vi "reg_visu OPC2.vi"(7 "object_name":string="W1", 9 "Останов\nпрограммы":bool) -> ()   [LabVIEW 2019]
uses:
  projects/Additivs/Regulators/PROG/GM1_201007/enums/AI.ctl
  Heating/ctl/general_init_client.ctl
  OPC/OPC UA Client.ctl
  <vilib>/OPCUA/controls/OPC UA Client Refnum.ctl
  <vilib>/OPCUA/controls/NodeId.ctl
  <vilib>/OPCUA/controls/NodeIds.ctl
  <vilib>/OPCUA/controls/Subscription ID.ctl
  <vilib>/OPCUA/controls/Write Variant Request.ctl
  <vilib>/OPCUA/controls/Write Status.ctl
  <vilib>/OPCUA/controls/Subscription Data Change.ctl
  <vilib>/OPCUA/controls/Data Type.ctl
  <vilib>/OPCUA/controls/OPC UA StatusCode.ctl
  Database/ctl/Coninfo.ctl
  Inputs/Ctl/Parameter State.ctl
  Alarms/Ctl/ALRs_State.ctl
  ctl/Y_short.ctl
  Inputs/Ctl/Parameter State short.ctl
  projects/Additivs/Regulators/PROG/GM1_201007/enums/KFM.ctl
  projects/Additivs/Regulators/PROG/GM1_201007/enums/PAR.ctl
  projects/Additivs/Regulators/PROG/GM1_201007/enums/DI.ctl
  projects/Additivs/Regulators/PROG/GM1_201007/enums/DI_FAST.ctl
  projects/Additivs/Regulators/PROG/GM1_201007/enums/AO.ctl
  projects/Additivs/Regulators/PROG/GM1_201007/enums/DO.ctl
  projects/Additivs/Regulators/PROG/GM1_201007/enums/ALR.ctl
  projects/Additivs/Regulators/PROG/GM1_201007/enums/System.ctl
  projects/Additivs/Regulators/PROG/GM1_201007/enums/REG.ctl
  bronkhorst/bronkhorstColumns.ctl
  <vilib>/picture/picture.llb/imagedata.ctl
  ctl/Ys_short.ctl
  389b3f70-cfa1-4025-b690-dd9bbc3cc1e4.vi
  cf2ac22c-c8a5-4ec0-ba3c-9dae82546773.vi
  Database/PostgreSQL2LabVIEW/libpqUtility/src/PQconnect.vi
  Database/PostgreSQL2LabVIEW/libpqUtility/src/PQclose.vi
  Database/select_initial_all.vi
  <vilib>/NI/AMC/Create Single Message.vi
  <vilib>/NI/AMC/Update Message Routing Info.vi
  <vilib>/NI/AMC/Read Termination Message.vi
  Transform/JSON to array.vi
  Database/PostgreSQL2LabVIEW/libpqlv/src/PQfinish.vi
  Database/PostgreSQL2LabVIEW/libpqlv/src/PQconnectdb.vi
  Database/PostgreSQL2LabVIEW/libpqlv/src/PQerrorMessage.vi
  Database/PostgreSQL2LabVIEW/libpqlv/src/PQstatus.vi
  <vilib>/dlg_ctls.llb/Space Constant.vi
  <vilib>/JDP Science/JSONtext/Find Multiple Items.vi
  <vilib>/JDP Science/JSONtext/String Subset.vi
  <vilib>/JDP Science/JSONtext/support/Strip Quotes and Unescape.vi
  <vilib>/JDP Science/JSONtext/support/Unescape JSON string.vi
  <vilib>/Utility/config.llb/Read Key (String).vi
  <vilib>/OPCUA/client/Multiple Read String Array.vi
  Database/PostgreSQL2LabVIEW/libpqUtility/src/PQgetTable.vi
  Database/Progress.vi
  <vilib>/OPCUA/client/Multiple Read ByteString Array.vi
  <vilib>/NI/AMC/Send Message.vi
  <vilib>/NI/AMC/Globals.vi
  <vilib>/OPCUA/client/Multiple Read String.vi
  <vilib>/JDP Science/JSONtext/JSON text to Variant.vi
  <vilib>/OPCUA/client/Multiple Write Variant.vi
  <vilib>/JDP Science/JSONtext/Parsing/Parse Full Path or Item Name.vi
  <vilib>/JDP Science/JSONtext/Offset/Find Item Locations by Path.vi
  <vilib>/JDP Science/JSONtext/Get Array Elements.vi
  Reg visu/Reg visu.lvclass
  <vilib>/JDP Science/JSONtext/LVClass Serializer/JSONtext LVClass Serializer.lvclass
  Heating/ctl/Z_State.ctl
  Heating/Heating.lvlib
  Heating/ctl/Y_state.ctl
  Heating/ctl/Y_source.ctl
  Heating/ctl/ZM_State.ctl
  <vilib>/NI/AMC/AMC.lvlib
  <vilib>/OPCUA/NI OPC UA Client.lvlib
  Database/PostgreSQL.lvlib
  <vilib>/Utility/config.llb/NI_LVConfig.lvlib
  projects/Additivs/Regulators/PROG/GM1_201007/enums/Param_h0gm1.lvlib
  Inputs/Inputs.lvlib
  control.lvlib
  OPC/OPC addons.lvlib
  Inputs/Ctl/DI short.ctl
  Alarms/Alarms.lvlib
  Heating/ctl/ZY_control.ctl
  Alarms/Ctl/ALR_Status_short.ctl
  Heating/ctl/Y_short.ctl
  Heating/ctl/Z.ctl
  Heating/ctl/ZY_state_short.ctl
  projects/Additivs/Regulators/PROG/GM1_201007/enums/scada_prog_state.ctl
  Heating/ctl/YQ2/YQ2.xctl
  Heating/ctl/Z_OnSwitch/Z_OnSwitch.xctl
  Heating/ctl/ZY_state_OPC.ctl
  7b03969a-a950-4454-9689-61267dd49491.vi
  fdeea6ee-2705-42e7-9783-53477a0f0781.vi
  00ce5b65-c19c-4f2f-b5a6-2d8b920d64b8.vi
  d49def32-a249-4c88-86f5-dd42ff10ee1e.vi
  847353ff-c4dc-4a0d-82d8-8a8c8b1dd027.vi
  96cb8638-67ee-45ab-9e65-4cb433c703bb.vi
  5d0f38f1-9d99-409f-81fc-f0eb7cf3d60e.vi
  fe7cfdb3-b4e0-46ae-bded-47b821cc5e2e.vi
  96416696-a13a-4191-9eaf-5b72f20cf204.vi
  bronkhorst/bronkhorst_reg.lvclass
  Reg visu1/Reg visu/Reg visu1.lvclass
  Heating/ctl/Z_source.ctl
  <vilib>/OPCUA/client/Multiple Read UInt32 Array.vi
  <vilib>/OPCUA/client/Multiple Read Double Array.vi
  <vilib>/OPCUA/client/Multiple Read Int32 Array.vi
  <vilib>/OPCUA/client/Multiple Read Bool Array.vi
panel:
  in  "Stop":bool caption="Останов программы"
  out "GM1QN1_XQ01":dbl caption="расход" format="%#.0f"
  in  "password data DB":string
  in  "password system DB":string
  in  "N 20":i32
  in  "N 19":i32
  in  "N 18":i32=16
  in  "N 17":i32=15
  in  "N 16":i32=14
  in  "N 15":i32=13
  in  "N 14":i32=12
  in  "N 13":i32=11
  in  "N 12":i32=10
  in  "N 11":i32=9
  in  "N 10":i32
  in  "N 9":i32
  in  "N 8":i32=8
  in  "N 7":i32=7
  in  "N 6":i32=6
  in  "N 5":i32=5
  in  "N 4":i32=4
  in  "N 3":i32=3
  in  "N 2":i32=2
  in  "N 1":i32=1
  out "Control Name":string="object_full_name"
  in  "gas 5":string="Осн."
  in  "gas 4":string="ОСНОВНОЙ 2"
  in  "gas 3":string="ОСНОВНОЙ 1"
  in  "HT1 emergency stop":bool caption="Аварийный сброс"
  in  "Reset":bool
  in  "Start":bool
  out "PV 2":dbl(slide) scale=0.0..50.0 scale format="%#_4g"
  in  "tick":u32=100 caption="Время цикла основной программы" min=5 max=1000 step=1
  out "EB3BP1_XQ01":dbl caption="kPa" format="%#.1f"
  in  "AI_enum":T1
  out "CPU %":dbl(slide) scale=0.0..100.0
  in  "message name":string="AI redefine"
  in  "process":bool
  in  "gas":string="РАБОЧИЕ ГАЗЫ"
  in  "gas 2":string="ПНГ1"
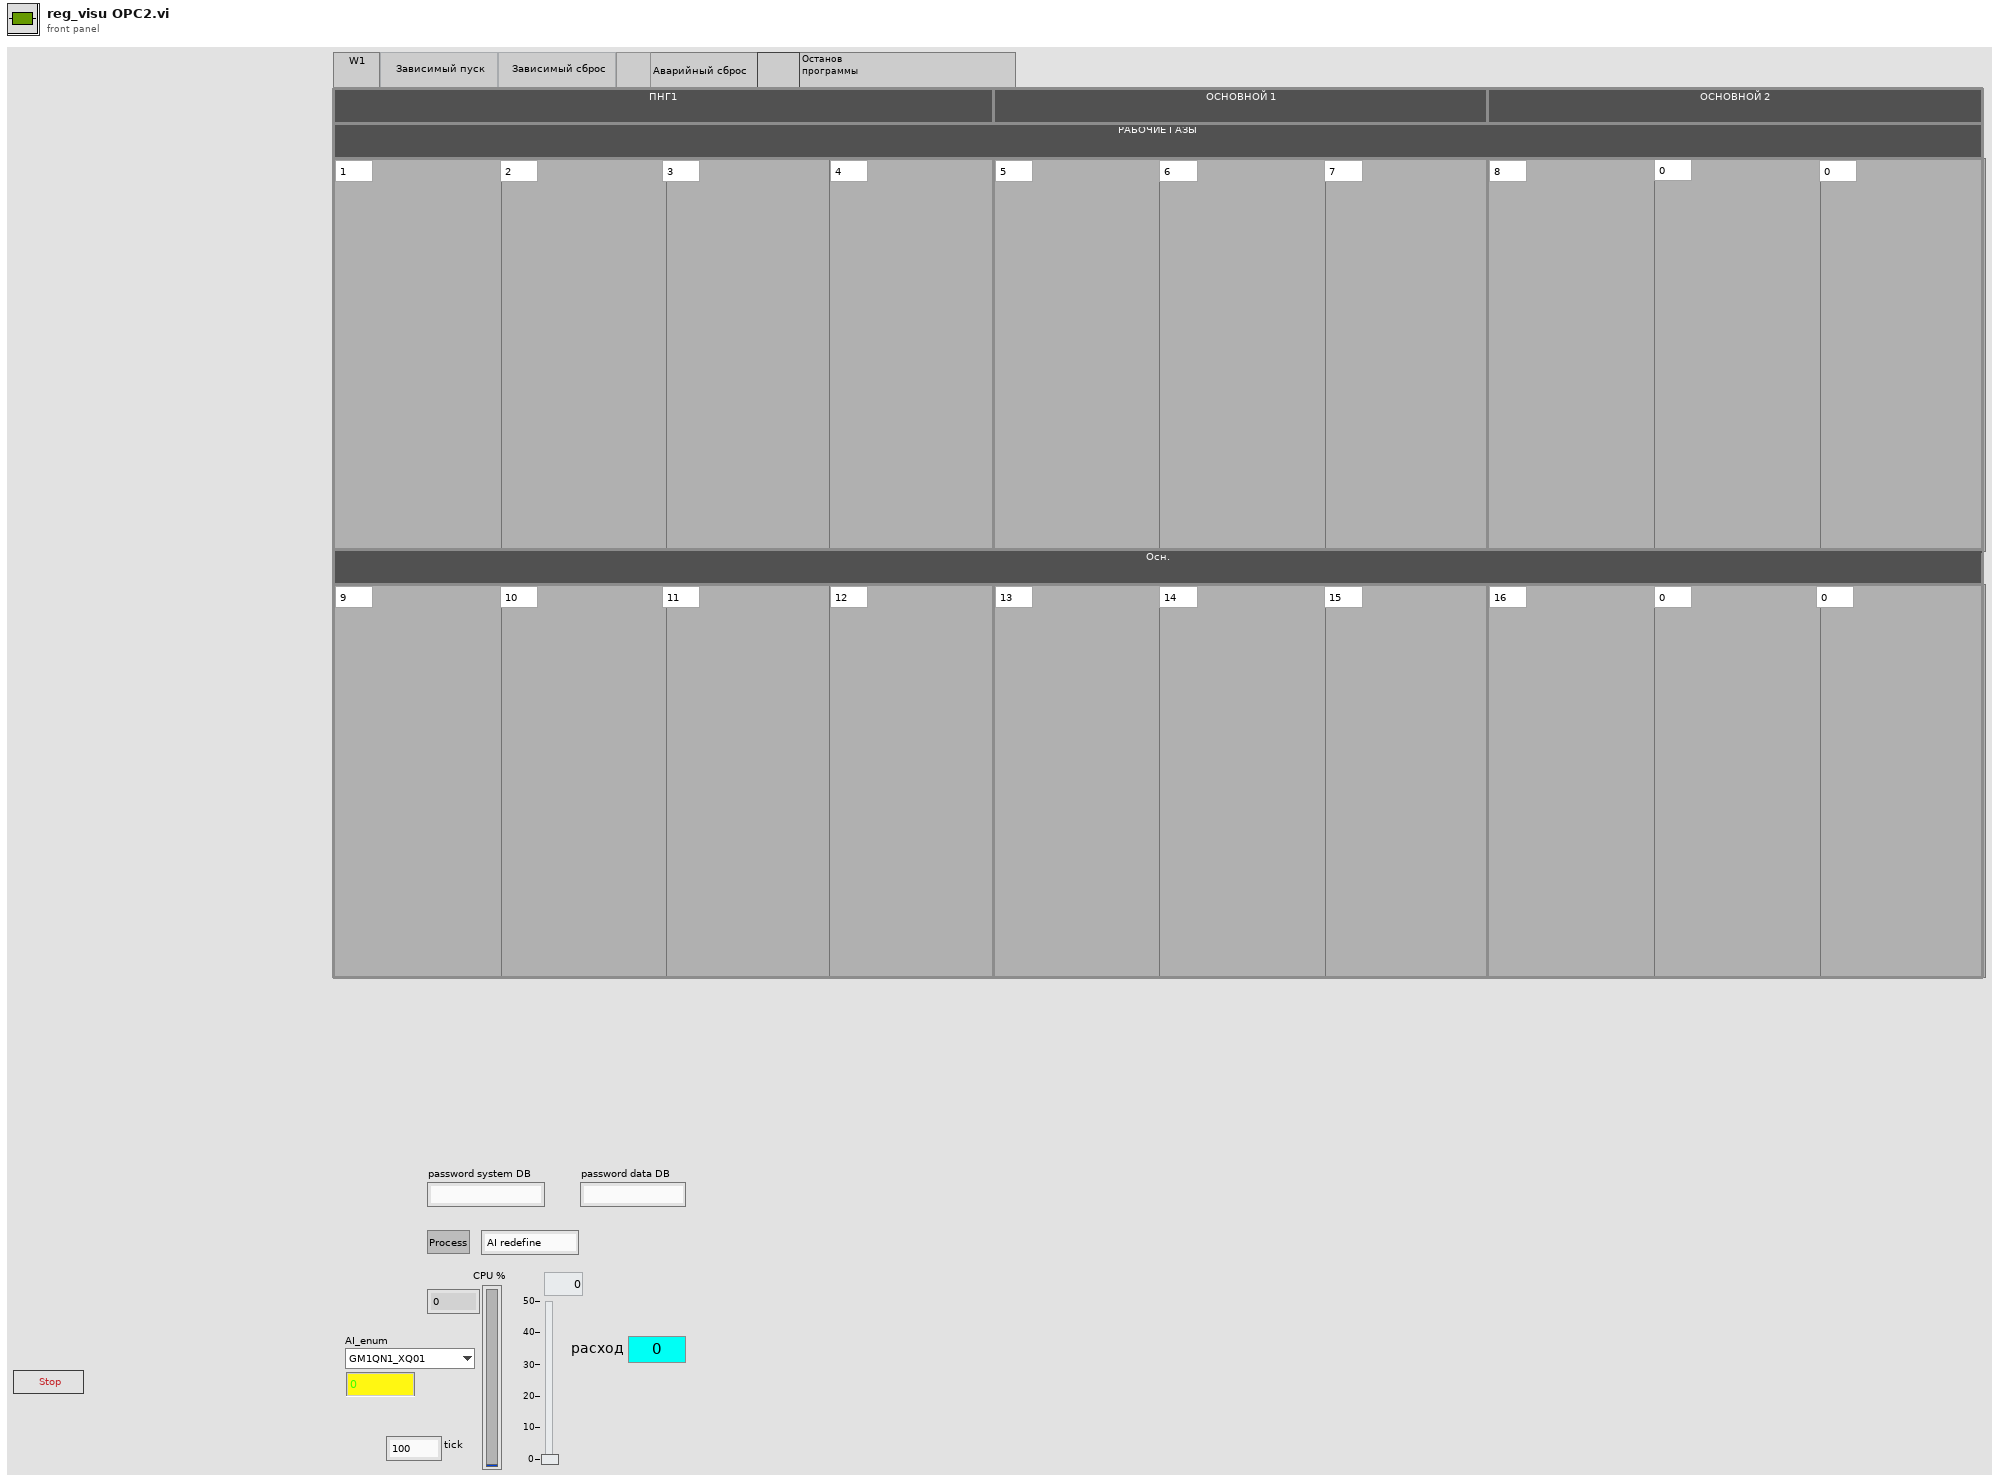
[diagram p1: front panel]
types:
  T1 = typedef "Param_h0gm1.lvlib/AI.ctl" = enum16{"GM1QN1_XQ01", "GM1QN2_XQ01", "GM1QN3_XQ01", "GM1QN4_XQ01", "GM1QN5_XQ01", "GM1QN6_XQ01", "GM1QN7_XQ01", "GM1QN8_XQ01", "GM1QN9_XQ01", "GM1QN10_XQ01", "GM1QN11_XQ01", "GM1QN12_XQ01", "GM1QN13_XQ01", "GM1QN14_XQ01", "GM1QN15_XQ01", "GM1QN16_XQ01", "GM1QN17_XQ01", "GM1QN18_XQ01", "GM1QN19_XQ01", "GM1QN20_XQ01", "GM1QN21_XQ01", "GM1QN22_XQ01", "GM1QN23_XQ01", "GM1QN1_XQ02", "GM1QN2_XQ02", "GM1QN3_XQ02", "GM1QN4_XQ02", "GM1QN5_XQ02", "GM1QN6_XQ02", "GM1QN7_XQ02", "GM1QN8_XQ02", "GM1QN9_XQ02", "GM1QN10_XQ02", "GM1QN11_XQ02", "GM1QN12_XQ02", "GM1QN13_XQ02", "GM1QN14_XQ02", "GM1QN15_XQ02", "GM1QN16_XQ02", "GM1QN17_XQ02", "GM1QN18_XQ02", "GM1QN19_XQ02", "GM1QN20_XQ02", "GM1QN21_XQ02", "GM1QN22_XQ02", "GM1QN23_XQ02"}
  T2 = typedef "Heating.lvlib/general_init_client.ctl" = enum16{"Init Data", "Init TMPs", "Read system DB param", "Read data DB param", "Read OPC param", "Read Enums", "Read Reg param", "Connect to OPC", "Read Param", "Read AI param", "AI references", "AI reorder", "AI reorder1", "AI Descriptions", "AI Descriptions1", "Read DI param", "Read AO param", "Read DO param", "Read ALR param", "Read control param", "Read state param", "Init save progs", "Init ALR Listbox symbols", "Init Y defs", "Init Shared Variables", "Exit"}
  T3 = typedef "AMC.lvlib/Message Queue.ctl" = refnum<queue>
  T4 = typedef "PostgreSQL.lvlib/Coninfo.ctl" = cluster{"host":string, "port":string, "client_encoding":string, "dbname":string, "user":string, "password":string}
  T5 = typedef "bronkhorst_reg.lvclass/bronkhorstColumns.ctl" = enum16{"instrument_range_max", "auto_value", "alr_value", "output_k", "output_set_time", "group", "process_units", "process_gas", "fcode", "fcode_full", "shortname"}
  T6 = typedef "NodeIds.ctl" = T7[]
  T7 = typedef "NodeId.ctl" = string
  T8 = typedef "Inputs.lvlib/DI short.ctl" = cluster{"DI":bool[], "DI_State":T9[], "DI_ALRState":errorcluster[]}
  T9 = typedef "Inputs.lvlib/Parameter State.ctl" = cluster{"code":i32, "visible":bool, "color":u32, "source":string}
  T10 = typedef "Alarms.lvlib/ALRs_State.ctl" = cluster{"ALR not block":bool[], "ALR":bool[], "ALR blocked":bool[], "ALR ON":bool[], "code":i32[], "level":i32[][], "t ms":u32[], "ack state":enum32{"not", "tripped", "reset", "ack"}[], "color":u32[]}
  T11 = typedef "control.lvlib/Y_short.ctl" = cluster{"Y_Source":u8, "Y_SetState":u8, "SP_Set":dbl, "SP":dbl, "PV":dbl, "PV_State":T12, "Y_preSet":dbl, "Y_Set":dbl, "Y":dbl, "Y_State":T12, "YB":bool}
  T12 = typedef "Inputs.lvlib/Parameter State short.ctl" = cluster{"code":i32, "visible":bool, "color":u32}
  T13 = cluster{"connect":bool, "gas":string, "Y_State":T11}
  T14 = cluster{"KFM":string[], "PAR":string[], "AI":string[], "DI":string[], "DI_fast":string[], "AO":string[], "Regs":string[], "DO":string[], "ALR":string[], "System":string[]}
  T15 = cluster{"name":string, "OPC port":string, "security policy":cluster{"message mode":enum16{"None", "Sign", "Sign and Encrypt"}, "security":enum16{"Basic256", "Basic128Rsa15"}}}
  T16 = typedef "OPC addons.lvlib/OPC UA Client.ctl" = cluster{"Client refnum":T17, "Folders":T7[], "node IDs":T6, "subscription IDs":T18[], "requests":T19[], "data change event":refnum<user-event>, "Event Reg":refnum<event-registration>}
  T17 = typedef "OPC UA Client Refnum.ctl" = refnum<k21>
  T18 = typedef "Subscription ID.ctl" = u32
  T19 = typedef "Write Variant Request.ctl" = cluster{"node ID":T7, "value":variant, "timestamp (current time)":timestamp, "node status":T20}
  T20 = typedef "Write Status.ctl" = u32
  T21 = cluster{"object_name":string, "N_KFMs":i32, "N_regs":i32, "Server":cluster{"name":string, "OPC port":string, "security policy":cluster{"message mode":enum16{"None", "Sign", "Sign and Encrypt"}, "security":enum16{"Basic256", "Basic128Rsa15"}}}, "Enums":cluster{"KFM":string[], "PAR":string[], "AI":string[], "DI":string[], "DI_fast":string[], "AO":string[], "Regs":string[], "DO":string[], "ALR":string[], "System":string[]}, "OPC UA":T16, "system DB":T4, "data DB":T4, "CPU_utilization":refnum<k21>, "AI_refs":refnum<vi>[], "AI_events":refnum<event-registration>, "AI_Descriptions":string[][], "DI_Descriptions":string[], "ALR_Descriptions":string[]}
  T22 = cluster{"connect":bool, "gas":string, "Y_State":T11}[]
  T23 = cluster{"AI_reorder_table":i32[], "AI":dbl[], "AIP":dbl[][], "AIState":T9[], "AIALRState":errorcluster[], "DI_reorder_table":i32[], "DI":bool[], "DIP":dbl[][], "DI_State":T9[], "ALR_State":T10, "ALR_Names":string[], "RegsParam":dbl[][], "Regs_State":cluster{"connect":bool, "gas":string, "Y_State":T11}[], "Regs_Descriptions":string[][], "RegRefs":refnum<vi>[], "system msg":string}
  T24 = typedef "NI_LVConfig.lvlib/Config Data RefNum.ctl" = refnum<k1>
  T25 = cluster{"[0]":string, "[1]":string, "[2]":string, "[3]":string, "[4]":string}
  T26 = typedef "Param_h0gm1.lvlib/REG.ctl" = enum16{"GM1QN1", "GM1QN2", "GM1QN3", "GM1QN4", "GM1QN5", "GM1QN6", "GM1QN7", "GM1QN8", "GM1QN9", "GM1QN10", "GM1QN11", "GM1QN12", "GM1QN13", "GM1QN14", "GM1QN15", "GM1QN16", "GM1QN17", "GM1QN18", "GM1QN19", "GM1QN20", "GM1QN21", "GM1QN22", "GM1QN23"}
  T27 = typedef "Param_h0gm1.lvlib/System.ctl" = enum16{"GM3HT1", "GM3HT2", "EB2TB1", "EB2TB2", "EB2TB3", "EB3TB1", "EB3TB2", "EB3TB3"}
  T28 = typedef "Param_h0gm1.lvlib/ALR.ctl" = enum16{"GM1JBA1JA1_CONN", "GM1JBA1JA2_CONN", "GM1JBA2JA1_CONN", "GM1JBA2JA2_CONN", "GM1JBA3JA1_CONN", "GM1QN1XQ01_SERR", "GM1QN2XQ01_SERR", "GM1QN3XQ01_SERR", "GM1QN4XQ01_SERR", "GM1QN5XQ01_SERR", "GM1QN6XQ01_SERR", "GM1QN7XQ01_SERR", "GM1QN8XQ01_SERR", "GM1QN9XQ01_SERR", "GM1QN10XQ01_SERR", "GM1QN11XQ01_SERR", "GM1QN12XQ01_SERR", "GM1QN13XQ01_SERR", "GM1QN14XQ01_SERR", "GM1QN15XQ01_SERR", "GM1QN16XQ01_SERR", "GM1QN17XQ01_SERR", "GM1QN18XQ01_SERR", "GM1QN19XQ01_SERR", "GM1QN20XQ01_SERR", "GM1QN21XQ01_SERR", "GM1QN22XQ01_SERR", "GM1QN23XQ01_SERR"}
  T29 = typedef "Param_h0gm1.lvlib/DO.ctl" = enum16{"GM1FZ1_YB47"}
  T30 = typedef "Param_h0gm1.lvlib/AO.ctl" = enum16{"GM1QN1_YQ01", "GM1QN2_YQ01", "GM1QN3_YQ01", "GM1QN4_YQ01", "GM1QN5_YQ01", "GM1QN6_YQ01", "GM1QN7_YQ01", "GM1QN8_YQ01", "GM1QN9_YQ01", "GM1QN10_YQ01", "GM1QN11_YQ01", "GM1QN12_YQ01", "GM1QN13_YQ01", "GM1QN14_YQ01", "GM1QN15_YQ01", "GM1QN16_YQ01", "GM1QN17_YQ01", "GM1QN18_YQ01", "GM1QN19_YQ01", "GM1QN20_YQ01", "GM1QN21_YQ01", "GM1QN22_YQ01", "GM1QN23_YQ01"}
  T31 = typedef "Param_h0gm1.lvlib/DI_FAST.ctl" = enum16{"W1.KF_XB01", "W1.KF_XB02", "W1.KF_XB03", "W1.KF_XB04", "W1.KF_XB05", "W1.KF_XB06", "W1.KF_XB07", "W1.KF_XB08", "W1.KF_XB09", "W1.KF_XB10", "W1.KF_XB11", "W1.KF_XB12", "W1.KF_XB13", "W1.KF_XB14", "W1.KF_XB15", "W1.KF_XB16"}
  T32 = typedef "Param_h0gm1.lvlib/DI.ctl" = enum16{"GM1FZ1_XB19"}
  T33 = typedef "Param_h0gm1.lvlib/PAR.ctl" = enum16{"GM1QN1_alr_value", "GM1QN1_auto_value", "GM1QN1_output_set_time", "GM1QN1_group", "GM1QN1_process_gas", "GM1QN2_alr_value", "GM1QN2_auto_value", "GM1QN2_output_set_time", "GM1QN2_group", "GM1QN2_process_gas", "GM1QN3_alr_value", "GM1QN3_auto_value", "GM1QN3_output_set_time", "GM1QN3_group", "GM1QN3_process_gas", "GM1QN4_alr_value", "GM1QN4_auto_value", "GM1QN4_output_set_time", "GM1QN4_group", "GM1QN4_process_gas", "GM1QN5_alr_value", "GM1QN5_auto_value", "GM1QN5_output_set_time", "GM1QN5_group", "GM1QN5_process_gas", "GM1QN6_alr_value", "GM1QN6_auto_value", "GM1QN6_output_set_time", "GM1QN6_group", "GM1QN6_process_gas", "GM1QN7_alr_value", "GM1QN7_auto_value", "GM1QN7_output_set_time", "GM1QN7_group", "GM1QN7_process_gas", "GM1QN8_alr_value", "GM1QN8_auto_value", "GM1QN8_output_set_time", "GM1QN8_group", "GM1QN8_process_gas", "GM1QN9_alr_value", "GM1QN9_auto_value", "GM1QN9_output_set_time", "GM1QN9_group", "GM1QN9_process_gas", "GM1QN10_alr_value", "GM1QN10_auto_value", "GM1QN10_output_set_time", "GM1QN10_group", "GM1QN10_process_gas", "GM1QN11_alr_value", "GM1QN11_auto_value", "GM1QN11_output_set_time", "GM1QN11_group", "GM1QN11_process_gas", "GM1QN12_alr_value", "GM1QN12_auto_value", "GM1QN12_output_set_time", "GM1QN12_group", "GM1QN12_process_gas", "GM1QN13_alr_value", "GM1QN13_auto_value", "GM1QN13_output_set_time", "GM1QN13_group", "GM1QN13_process_gas", "GM1QN14_alr_value", "GM1QN14_auto_value", "GM1QN14_output_set_time", "GM1QN14_group", "GM1QN14_process_gas", "GM1QN15_alr_value", "GM1QN15_auto_value", "GM1QN15_output_set_time", "GM1QN15_group", "GM1QN15_process_gas", "GM1QN16_alr_value", "GM1QN16_auto_value", "GM1QN16_output_set_time", "GM1QN16_group", "GM1QN16_process_gas", "GM1QN17_alr_value", "GM1QN17_auto_value", "GM1QN17_output_set_time", "GM1QN17_group", "GM1QN17_process_gas", "GM1QN18_alr_value", "GM1QN18_auto_value", "GM1QN18_output_set_time", "GM1QN18_group", "GM1QN18_process_gas", "GM1QN19_alr_value", "GM1QN19_auto_value", "GM1QN19_output_set_time", "GM1QN19_group", "GM1QN19_process_gas", "GM1QN20_alr_value", "GM1QN20_auto_value", "GM1QN20_output_set_time", "GM1QN20_group", "GM1QN20_process_gas", "GM1QN21_alr_value", "GM1QN21_auto_value", "GM1QN21_output_set_time", "GM1QN21_group", "GM1QN21_process_gas", "GM1QN22_alr_value", "GM1QN22_auto_value", "GM1QN22_output_set_time", "GM1QN22_group", "GM1QN22_process_gas", "GM1QN23_alr_value", "GM1QN23_auto_value", "GM1QN23_output_set_time", "GM1QN23_group", "GM1QN23_process_gas"}
  T34 = typedef "Param_h0gm1.lvlib/KFM.ctl" = enum16{"GM1JBA1_JA1", "GM1JBA1_JA2", "GM1JBA2_JA1", "GM1JBA2_JA2", "GM1JBA3_JA1"}
  T35 = cluster{"message mode":enum16{"None", "Sign", "Sign and Encrypt"}, "security":enum16{"Basic256", "Basic128Rsa15"}}
  T36 = typedef "OPC addons.lvlib/OPC tag.ctl" = cluster{"name":string, "data type":T37, "access level":T38, "description":string, "period":T39}
  T37 = typedef "Data Type.ctl" = u16
  T38 = typedef "OPC addons.lvlib/Access level.ctl" = enum16{"none", "read-only", "write-only", "read/write"}
  T39 = typedef "OPC addons.lvlib/Period.ctl" = enum16{"on_load", "100 ms", "500 ms", "1 s"}
  T40 = cluster{"sampling interval":dbl, "queue size":u32, "discard oldest":bool, "data change filter":cluster{"trigger":enum32{"Status", "StatusValue", "StatusValueTimestamp"}, "deadband type":enum32{"None", "Absolute", "Percent"}, "deadband value":dbl}}[]
  T41 = typedef "OPC UA StatusCode.ctl" = u32
  T42 = cluster{"node ID":T7, "values ":string[], "timestamp":timestamp, "status":T41}[]
  T43 = cluster{"node ID":T7, "values ":string[], "timestamp":timestamp, "status":T41}
  T44 = cluster{"Read Access":enum8{"Allowed", "Required", "None"}, "Write Access":enum8{"Allowed", "Required", "None"}}
  T45 = cluster{"node ID":T7, "values ":u8[][], "timestamp":timestamp, "status":T41}[]
  T46 = cluster{"node ID":T7, "values ":u8[][], "timestamp":timestamp, "status":T41}
  T47 = typedef "Heating.lvlib/ZY_control.ctl" = cluster{"Z_HSw":u8, "Z_HSetState":T48, "Y_HSw":u8, "Y_HSetState":T49, "SP":dbl, "Y_H":dbl, "Reset_ALR":bool}
  T48 = typedef "Heating.lvlib/Z_State.ctl" = enum8{"initialization", "alarm", "disabled", "not ready", "stop ready", "reserv", "switched off", "reserv2", "switched on", "check", "on min", "decrease out", "on", "increase out", "on max"}
  T49 = typedef "Heating.lvlib/Y_state.ctl" = enum8{"initialize", "alarm", "min", "stop", "hand", "auto", "max"}
  T50 = typedef "Heating.lvlib/ZY_state_short.ctl" = cluster{"Z":T51, "Y":T54, "ALR_Status":T56[]}
  T51 = typedef "Heating.lvlib/Z.ctl" = cluster{"Z_Source":T52, "Z_SetState":T48, "Z_State":T48, "Z_State_T":u32, "ZM_State":T53, "ZM_State_T":u32, "ALR  L1":bool, "ALR  L2":bool, "HH_run":u64}
  T52 = typedef "Heating.lvlib/Z_source.ctl" = enum8{"initialize", "local disabled", "local hand", "hand", "auto", "dist"}
  T53 = typedef "Heating.lvlib/ZM_State.ctl" = enum8{"initialization", "stop", "start_cmd", "contactor_on_cmd", "heating", "on", "stop_cmd", "power_down", "contactor_off_cmd", "cooling", "restart_delay"}
  T54 = typedef "Heating.lvlib/Y_short.ctl" = cluster{"Y_Source":T55, "Y_SetState":T49, "SP_Set":dbl, "SP":dbl, "PV":dbl, "Y_Set":dbl, "Y":dbl, "Y_State":T12, "YB":bool}
  T55 = typedef "Heating.lvlib/Y_source.ctl" = enum8{"initialize", "local disabled", "local hand", "hand", "auto", "dist"}
  T56 = typedef "Alarms.lvlib/ALR_Status_short.ctl" = cluster{"status":bool, "code":i32, "level":i32}
  T57 = typedef "imagedata.ctl" = cluster{"image type":i32, "image depth":i32, "image":u8[], "mask":u8[], "colors":u32[], "Rectangle":cluster{"left":i16, "top":i16, "right":i16, "bottom":i16}}
  T58 = typedef "AMC.lvlib/Message.ctl" = cluster{"name":string, "value":string, "attributes":T59, "receiver host":string, "receiver process":string, "source host":string, "source process":string, "priority message":bool, "acknowledge message":bool}
  T59 = typedef "Tools_KeyedArray.lvlib/KeyedArray.ctl" = cluster{"keys":string[], "values":string[]}
  T60 = cluster{"node ID":T7, "value ":string, "timestamp":timestamp, "status":T41}[]
  T61 = typedef "control.lvlib/Ys_short.ctl" = cluster{"connect":bool, "gas":string, "Y_State":T11}[]
  T62 = typedef "Param_h0gm1.lvlib/scada_prog_state.ctl" = enum16{"ReadAIParam", "ReadAIParam1", "ReadDIParam", "AI", "AI1", "AIValues", "AIValues1", "DI", "DiValues", "Alarms", "Messages", "TB1", "TB2", "TB3", "Control EB3", "Outputs", "Exit"}
  T63 = cluster{"connect":bool, "Z_Source":T55, "Z_State_heating":T48}
  T64 = typedef "Heating.lvlib/ZY_state_OPC.ctl" = cluster{"Z":cluster{"Z_Source":u8, "Z_SetState":u8, "Z_State":u8, "Z_State_T":u32, "ZM_State":u8, "ZM_State_T":u32, "ALR  L1":bool, "ALR  L2":bool, "HH_run":i32}, "Y":cluster{"Y_Source":u8, "Y_SetState":u8, "SP_Set":dbl, "SP":dbl, "PV":dbl, "Y_Set":dbl, "Y":dbl, "Y_State":cluster{"code":i32, "visible":bool, "color":u32}, "YB":bool}, "ALR_Status":cluster{"status":bool, "code":i32, "level":i32}[]}
  T65 = typedef "Heating.lvlib/ZY_state_short.ctl" = cluster{"Z":T66, "Y":T54, "ALR_Status":T56[]}
  T66 = typedef "Heating.lvlib/Z.ctl" = cluster{"Z_Source":T55, "Z_SetState":T48, "Z_State":T48, "Z_State_T":u32, "ZM_State":T53, "ZM_State_T":u32, "ALR  L1":bool, "ALR  L2":bool, "HH_run":i32}
  T67 = cluster{"node ID":T7, "values ":dbl[], "timestamp":timestamp, "status":T41}[]
  T68 = cluster{"node ID":T7, "values ":i32[], "timestamp":timestamp, "status":T41}[]
  T69 = cluster{"node ID":T7, "values ":dbl[], "timestamp":timestamp, "status":T41}
  T70 = cluster{"node ID":T7, "values ":i32[], "timestamp":timestamp, "status":T41}
  T71 = typedef "Inputs.lvlib/AI short.ctl" = cluster{"AI":dbl[], "AIState":T9[], "AIALRState":errorcluster[]}
  T72 = cluster{"node ID":T7, "values ":bool[], "timestamp":timestamp, "status":T41}[]
  T73 = cluster{"node ID":T7, "values ":bool[], "timestamp":timestamp, "status":T41}
  T74 = cluster{"node ID":T7, "values ":u32[], "timestamp":timestamp, "status":T41}[]
  T75 = cluster{"node ID":T7, "values ":u32[], "timestamp":timestamp, "status":T41}
  T76 = cluster{"node ID":T7, "value ":string, "timestamp":timestamp, "status":T41}
  T77 = typedef "Heating.lvlib/ZY_state_short.ctl" = cluster{"Z":T66, "Y":T78, "ALR_Status":T56[]}
  T78 = typedef "Heating.lvlib/Y_short.ctl" = cluster{"Y_Source":T55, "Y_SetState":T49, "SP_Set":dbl, "SP":dbl, "PV":dbl, "Y":dbl, "Y_State":T12, "YB":bool}
  T79 = enum32{"invalid app kind", "Development System", "Run Time System", "Student Edition", "Embedded LabVIEW", "Evaluation", "Custom"}
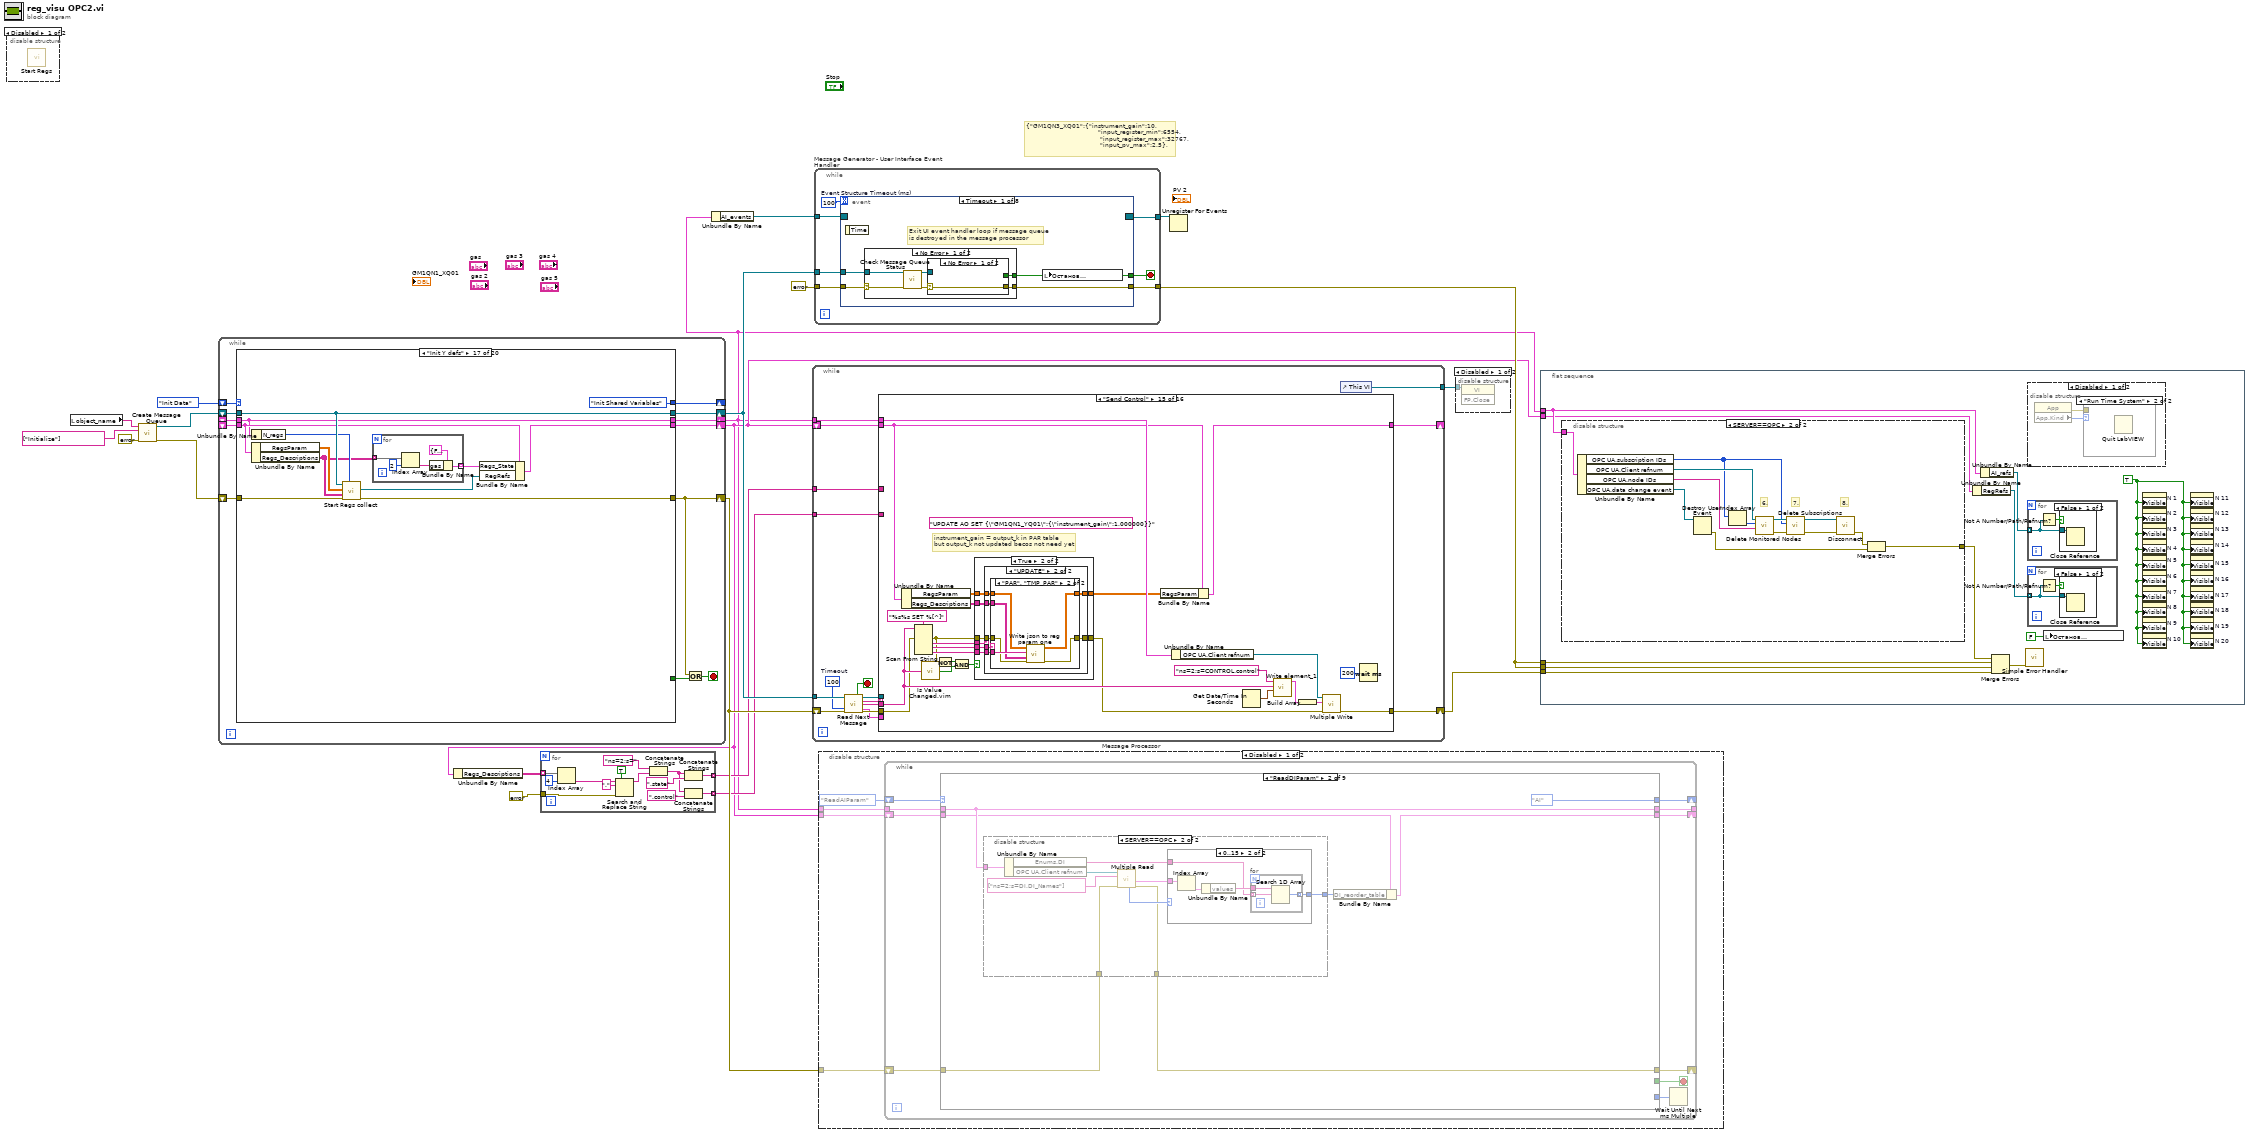
[diagram p0: block diagram]
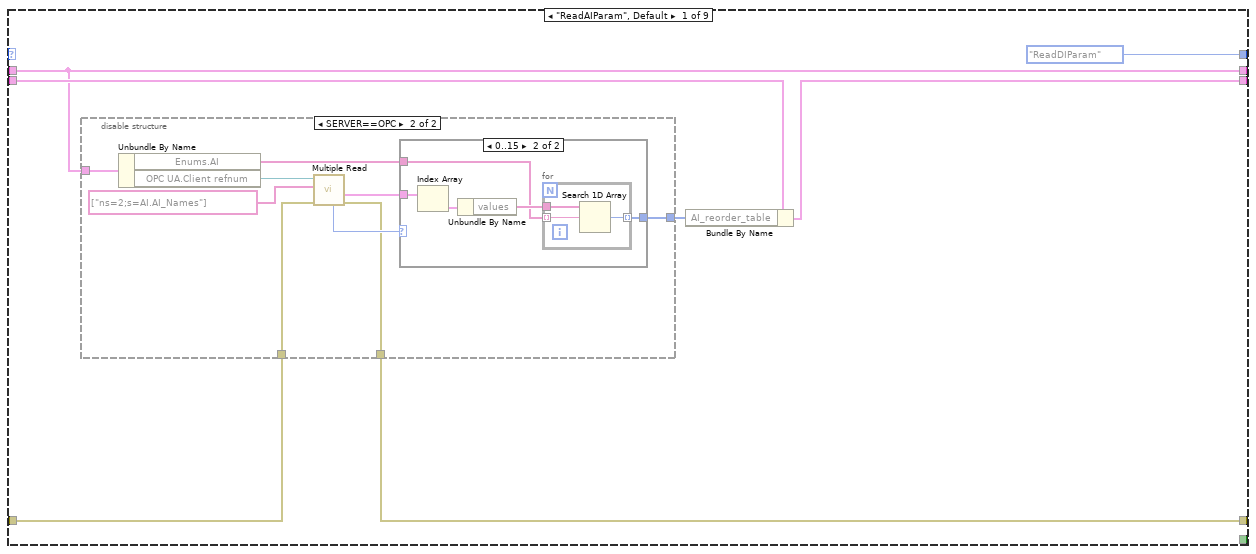
[diagram p2: hidden frame]
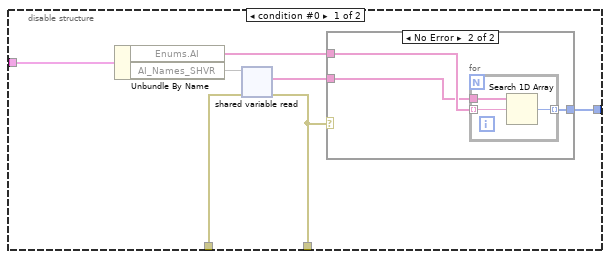
[diagram p3: hidden frame]
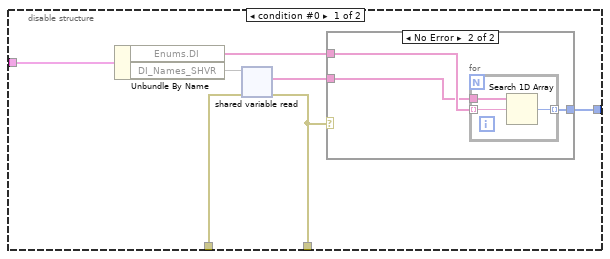
[diagram p6: hidden frame]
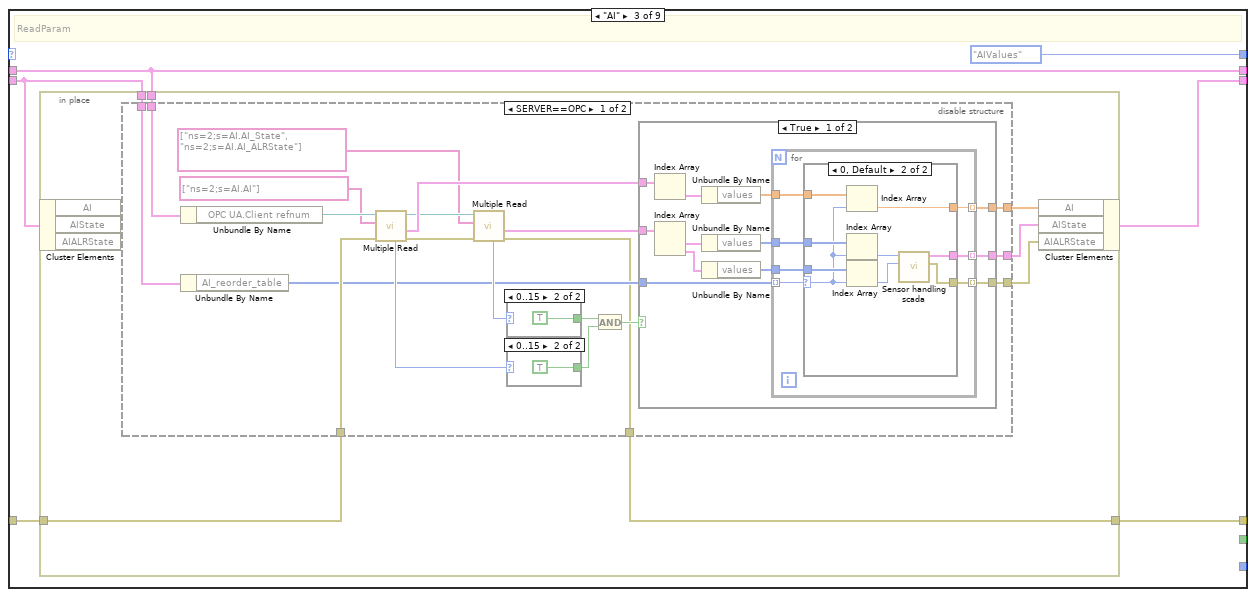
[diagram p9: hidden frame]
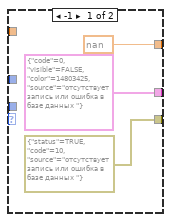
[diagram p12: hidden frame]
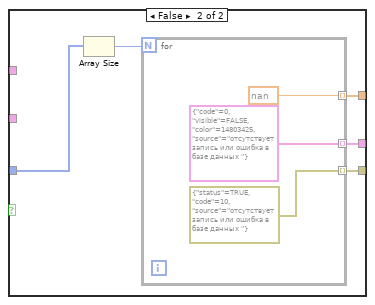
[diagram p13: hidden frame]
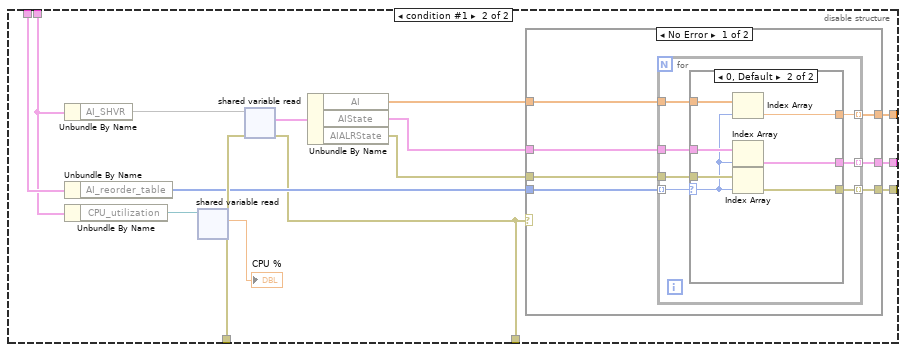
[diagram p14: hidden frame]
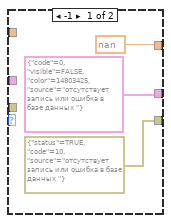
[diagram p15: hidden frame]
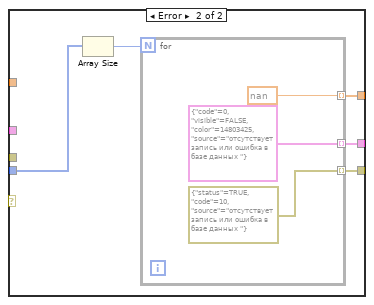
[diagram p16: hidden frame]
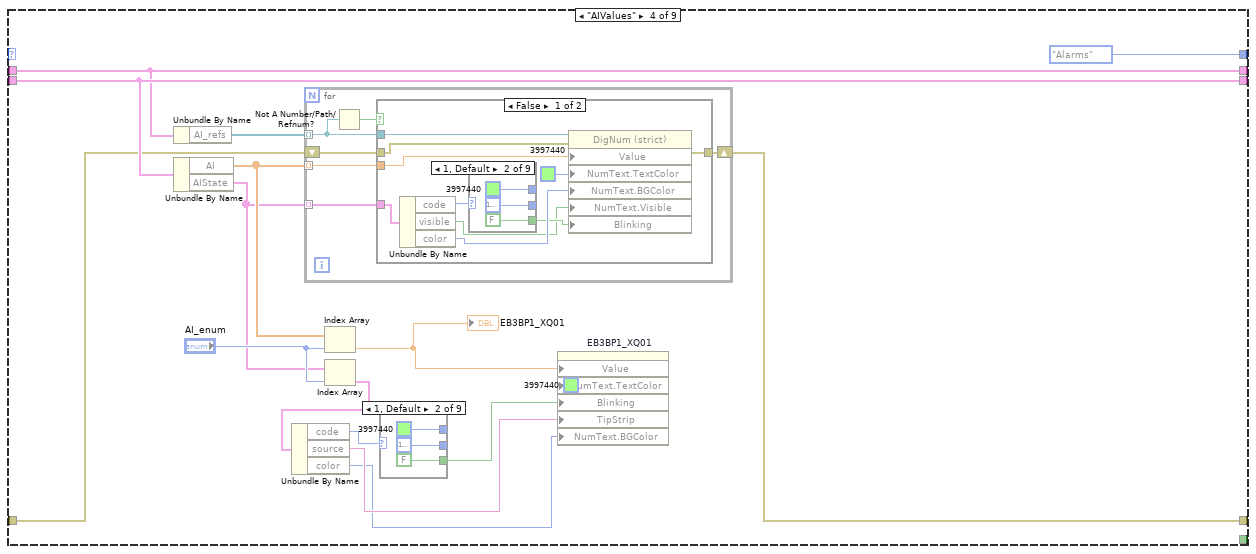
[diagram p17: hidden frame]
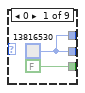
[diagram p18: hidden frame]
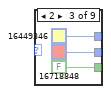
[diagram p19: hidden frame]
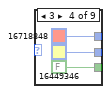
[diagram p20: hidden frame]
diagram:
  # "{\"GM1QN3_XQ01\":{\"instrument_gain\":10,\n                                    \"input_register_min\":6554,\n                                     \"input_register_max\":32767,\n                                     \"input_pv_max\":2.5},"
  n1 = disable-structure shown="Disabled" {
    frame Disabled {
      n2 = call "Start Regs.vi"() -> ()  [unwired: 11 in, 1 out]
    }
    frame Enabled {
    }
  }
  n3 = local read "object_name"() -> (w18:string)
  n4 = call <vilib>:"Create Message Queue.vi"("message queue name"=w18, "initial message names"=string[] ["Initialize"], "error in"=errorcluster {"status"=FALSE, "code"=0, "source"=""}) -> ("message queue out"=w13:T3, "error out"=w15:errorcluster)  [unwired: 11 in]
  n5 = while {
    shift-right: [w21] -> w9
    shift-left: w15 -> [w29]
    shift-right: [w32] -> w2
    shift-left: _ -> [w30]
    shift-right: [w28] -> _
    shift-left: general_init_client."Init Data" -> [w31]
    shift-right: [w25] -> w5
    shift-left: _ -> [w24]
    shift-right: [w22] -> w12
    shift-left: w13 -> [w23]
    stop <- w26 stop-if-true
    n6 = case shown="\"Init Y defs\"" w31 {
      tunnel: [w49 w71 w92 w139 w175 w204 w234 w239 w275 w300 w313 w340 w376 w419 w447 w474 w498 w512 w518 w521] -> w21
      selector: w31 -> [_ _ _ _ _ _ _ _ _ _ _ _ _ _ _ _ _ _ _ w524]
      tunnel: [w50 w69 w88 w135 w176 w218 w233 w240 w279 w299 w314 w342 w377 w421 w449 w487 w494 w509 w519 w522] -> w32
      tunnel: w30 -> [_ w69 w90 w137 w173 w220 w233 w238 w278 w299 w317 w339 w370 w418 w446 w487 w494 w509 w519 w522]
      tunnel: w29 -> [w49 w71 w99 w146 w172 w186 w235 w242 w276 w301 w318 w343 w371 w422 w450 w474 w499 w511 w518 w521]
      tunnel: [general_init_client."Init TMPs" general_init_client."Read system DB param" general_init_client."Read data DB param" general_init_client."Read OPC param" general_init_client."Read Enums" general_init_client."Read Reg param" general_init_client."Connect to OPC" general_init_client."AI references" general_init_client."AI reorder" general_init_client."AI Descriptions" general_init_client."Read DI param" general_init_client."Read ALR param" general_init_client."Read control param" general_init_client."Read state param" general_init_client."Init ALR Listbox symbols" general_init_client."Init Y defs" general_init_client."Init Shared Variables" general_init_client."Exit" general_init_client."Init Data" w523] -> w28
      tunnel: [_ _ _ _ _ _ _ _ _ _ _ _ _ _ _ _ _ _ TRUE _] -> w27
      tunnel: [w47 w64 w101 w148 w178 w222 w232 w243 w282 w298 w316 w341 w369 w420 w448 w490 w496 w508 w516 w526] -> w25
      tunnel: w24 -> [w47 _ w101 w148 w178 w222 w231 w243 w282 w297 w315 w341 w368 w420 w448 w490 w495 w508 w516 w526]
      tunnel: w23 -> [w48 w70 w100 w147 w177 w203 w237 w241 w284 w304 w326 w345 w379 w424 w452 w489 w501 w514 w515 w525]
      tunnel: [w48 w70 w100 w147 w177 w203 w237 w241 w284 w304 w326 w345 w379 w424 w452 w489 w501 w514 w515 w525] -> w22
      frame "Init Data" {
        w33 = refnum<vi>[] []  # AI_refs
        w34 = T4 {"host"="localhosh", "port"="5432", "client_encoding"="LATIN1", "dbname"="system", "user"="postgres", "password"=""}  # data DB
        w35 = refnum<event-registration> refnum  # AI_events
        w37 = 0  # N_regs
        w36 = 0  # N_KFMs
        w38 = T14 {"KFM"=[], "PAR"=[], "AI"=[], "DI"=[], "DI_fast"=[], "AO"=[], "Regs"=[], "DO"=[], "ALR"=[], "System"=[]}  # Enums
        w40 = string[] []  # DI_Descriptions
        w41 = string[][] []  # AI_Descriptions
        w39 = string[] []  # ALR_Descriptions
        w42 = refnum<k21> refnum  # CPU_utilization
        w44 = T15 {"name"="H1", "OPC port"="49580", "security policy"={"message mode"=enum."None", "security"=enum."Basic256"}}  # Server
        w46 = T4 {"host"="localhosh", "port"="5432", "client_encoding"="LATIN1", "dbname"="system", "user"="postgres", "password"=""}  # system DB
        w45 = T16 {"Client refnum"="", "Folders"=[], "node IDs"=[], "subscription IDs"=[], "requests"=[], "data change event"=refnum, "Event Reg"=refnum}  # OPC UA
        n7 = Bundle("object_name"="object_name", "N_KFMs"=w36, "N_regs"=w37, "Server"=w44, "Enums"=w38, "OPC UA"=w45, "system DB"=w46, "data DB"=w34, "CPU_utilization"=w42, "AI_refs"=w33, "AI_events"=w35, "AI_Descriptions"=w41, "DI_Descriptions"=w40, "ALR_Descriptions"=w39) -> (w50:T21)  [unwired: 1 in]
      }
      frame "Init TMPs" {
        w54 = T22 []  # Regs_State
        w55 = refnum<vi>[] []  # RegRefs
        w57 = string[][] []  # Regs_Descriptions
        w58 = dbl[][] []  # RegsParam
        w59 = string[] []  # ALR_Names
        w60 = T10 {"ALR not block"=[], "ALR"=[], "ALR blocked"=[], "ALR ON"=[], "code"=[], "level"=[], "t ms"=[], "ack state"=[], "color"=[]}  # ALR_State
        w56 = ""  # system msg
        w61 = i32[] []  # DI_reorder_table
        w63 = i32[] []  # AI_reorder_table
        w68 = T9[] []  # AIState
        w67 = errorcluster[] []  # AIALRState
        w66 = bool[] []  # DI
        w52 = dbl[][] []  # DIP
        w65 = T9[] []  # DI_State
        w53 = dbl[][] []  # AIP
        w62 = dbl[] []  # AI
        n8 = Bundle("AI_reorder_table"=w63, "AI"=w62, "AIP"=w53, "AIState"=w68, "AIALRState"=w67, "DI_reorder_table"=w61, "DI"=w66, "DIP"=w52, "DI_State"=w65, "ALR_State"=w60, "ALR_Names"=w59, "RegsParam"=w58, "Regs_State"=w54, "Regs_Descriptions"=w57, "RegRefs"=w55, "system msg"=w56) -> (w64:T23)  [unwired: 1 in]
      }
      frame "Read system DB param" {
        n9 = disable-structure shown="Default" {
          disable-tunnel: [w118 w119] -> w93
          frame condition #0 (active) {
            n10 = call <vilib>:"Application Directory.vi"() -> ("Application Directory"=w118:path)
          }
          frame condition #1 {
            n11 = call <vilib>:"Dflt Data Dir.vi"() -> ("App:Default Data Directory"=w119:path)
          }
        }
        n12 = Build Path(base path=w93, name or relative path=path "DB.ini" ("configuration file path")) -> (appended path=w98:path)
        n13 = Unbundle By Name(w90) -> ("system DB"=w82:T4)
        n14 = call <vilib>:"Open Config Data.vi"("error in (no error)"=w99, "configuration file path"=w98) -> ("error out"=w96:errorcluster, "refnum"=w95:T24)  [unwired: 7 in, 1 out]
        n15 = Empty String/Path?(string/path="password system DB") -> (empty?=w87:bool)
        n16 = case shown="True" w87 {
          tunnel: [w103 w104] -> w85
          tunnel: "password system DB" -> [w103 _]
          frame False {
          }
          frame True {
            n17 = String To Byte Array(string="Ъ«Р\u001dЛЈu#ш·/f'") -> (unsigned byte array=w109:u8[])
            n18 = String To Byte Array(string="ЉГ¤.уђF\u0017МЋ\u001aT\u0012Pн_") -> (unsigned byte array=w107:u8[])
            n19 = Exclusive Or(1:w107, 2:w109) -> (0:w106:u8[])
            n20 = Byte Array To String(unsigned byte array=w106) -> (string=w104:string)
          }
        }
        n21 = Cluster To Array(cluster=w82) -> (array=w81:string[])
        n22 = for {
          tunnel: "System_DB" ("key") -> [w114]
          tunnel: w81 -> [w112] mode=indexing
          shift-right: [w111] -> w74
          shift-left: w96 -> [w117]
          shift-right: [w110] -> w73
          shift-left: w95 -> [w116]
          tunnel: string[] ["host", "port", "clint_encoding", "dbname", "user"] -> [w115] mode=indexing
          tunnel: [w113] -> w83 mode=indexing
          n23 = call-poly <vilib>:"Read Key.vi"("section"=w114, "error in (no error)"=w117, "default value"=w112, "key"=w115, "refnum"=w116) -> ("error out"=w111:errorcluster, "value"=w113:string, "refnum out"=w110:T24)  [unwired: 3 in, 1 out]
        }
        n24 = Array To Cluster(array=w83) -> (cluster=w80:T25)
        n25 = call <vilib>:"Close Config Data.vi"("error in (no error)"=w74, "refnum"=w73) -> ("error out"=w92:errorcluster)  [unwired: 8 in, 1 out]
        n26 = Unbundle(w80) -> ("[0]"=w79:string, "[1]"=w78:string, "[2]"=w77:string, "[3]"=w76:string, "[4]"=w75:string)
        n27 = Bundle By Name(cluster=T4 {"host"="localhosh", "port"="5432", "client_encoding"="LATIN1", "dbname"="system", "user"="postgres", "password"=""} ("system DB"), "host"=w79, "port"=w78, "client_encoding"=w77, "dbname"=w76, "user"=w75, "password"=w85) -> (w89:T4)
        n28 = Bundle By Name(cluster=w90, "system DB"=w89) -> (w88:T21)
      }
      frame "Read data DB param" {
        n29 = disable-structure shown="Default" {
          disable-tunnel: [w165 w166] -> w140
          frame condition #0 (active) {
            n30 = call <vilib>:"Application Directory.vi"() -> ("Application Directory"=w165:path)
          }
          frame condition #1 {
            n31 = call <vilib>:"Dflt Data Dir.vi"() -> ("App:Default Data Directory"=w166:path)
          }
        }
        n32 = Build Path(base path=w140, name or relative path=path "DB.ini" ("configuration file path")) -> (appended path=w145:path)
        n33 = Unbundle By Name(w137) -> ("data DB"=w129:T4)
        n34 = call <vilib>:"Open Config Data.vi"("error in (no error)"=w146, "configuration file path"=w145) -> ("error out"=w143:errorcluster, "refnum"=w142:T24)  [unwired: 7 in, 1 out]
        n35 = Empty String/Path?(string/path="password data DB") -> (empty?=w134:bool)
        n36 = case shown="True" w134 {
          tunnel: [w150 w151] -> w132
          tunnel: "password data DB" -> [w150 _]
          frame False {
          }
          frame True {
            n37 = String To Byte Array(string="Ъ«Р\u001dЛЈu#ш·/f'") -> (unsigned byte array=w156:u8[])
            n38 = String To Byte Array(string="ЉГ¤.уђF\u0017МЋ\u001aT\u0012Pн_") -> (unsigned byte array=w154:u8[])
            n39 = Exclusive Or(1:w154, 2:w156) -> (0:w153:u8[])
            n40 = Byte Array To String(unsigned byte array=w153) -> (string=w151:string)
          }
        }
        n41 = Cluster To Array(cluster=w129) -> (array=w128:string[])
        n42 = for {
          tunnel: "Data_DB" ("key") -> [w161]
          tunnel: w128 -> [w159] mode=indexing
          shift-right: [w158] -> w121
          shift-left: w143 -> [w164]
          shift-right: [w157] -> w120
          shift-left: w142 -> [w163]
          tunnel: string[] ["host", "port", "clint_encoding", "dbname", "user"] -> [w162] mode=indexing
          tunnel: [w160] -> w130 mode=indexing
          n43 = call-poly <vilib>:"Read Key.vi"("section"=w161, "error in (no error)"=w164, "default value"=w159, "key"=w162, "refnum"=w163) -> ("error out"=w158:errorcluster, "value"=w160:string, "refnum out"=w157:T24)  [unwired: 3 in, 1 out]
        }
        n44 = Array To Cluster(array=w130) -> (cluster=w127:T25)
        n45 = call <vilib>:"Close Config Data.vi"("error in (no error)"=w121, "refnum"=w120) -> ("error out"=w139:errorcluster)  [unwired: 8 in, 1 out]
        n46 = Unbundle(w127) -> ("[0]"=w126:string, "[1]"=w125:string, "[2]"=w124:string, "[3]"=w123:string, "[4]"=w122:string)
        n47 = Bundle By Name(cluster=T4 {"host"="localhosh", "port"="5432", "client_encoding"="LATIN1", "dbname"="system", "user"="postgres", "password"=""} ("system DB"), "host"=w126, "port"=w125, "client_encoding"=w124, "dbname"=w123, "user"=w122, "password"=w132) -> (w136:T4)
        n48 = Bundle By Name(cluster=w137, "data DB"=w136) -> (w135:T21)
      }
      frame "Read OPC param" {
        n49 = disable-structure shown="Default" {
          disable-tunnel: [w180 w181] -> w170
          frame condition #0 (active) {
            n50 = call <vilib>:"Application Directory.vi"() -> ("Application Directory"=w180:path)
          }
          frame condition #1 {
            n51 = call <vilib>:"Dflt Data Dir.vi"() -> ("App:Default Data Directory"=w181:path)
          }
        }
        n52 = Build Path(base path=w170, name or relative path=path "DB.ini" ("configuration file path")) -> (appended path=w168:path)
        n53 = Unbundle By Name(w173) -> ("Server"=w169:T15)
        n54 = call "Read OPC ini param.vi"("error in (no error)"=w172, "configuration file path"=w168, "key"="Server", "Server in"=w169) -> ("error out"=w175:errorcluster, "Server out"=w174:T15)  [unwired: 6 in]
        n55 = Bundle By Name(cluster=w173, "Server"=w174) -> (w176:T21)
      }
      frame "Read Enums" {
        w190 = REG."GM1QN9"  # REG
        w187 = System."GM3HT1"  # System_enum
        w188 = ALR."GM1JBA1JA1_CONN"  # ALR_enum
        w189 = DO."GM1FZ1_YB47"  # DO_enum
        w191 = AO."GM1QN1_YQ01"  # AO_enum
        w192 = DI_FAST."W1.KF_XB01"  # DI_enum fast
        w193 = DI."GM1FZ1_XB19"  # DI_enum
        w194 = AI."GM1QN1_XQ01"  # AI_enum
        w195 = PAR."GM1QN1_output_set_time"  # PAR_enum
        w196 = KFM."GM1JBA1_JA1"  # KFM_enum
        w217 = T14 {"KFM"=[], "PAR"=[], "AI"=[], "DI"=[], "DI_fast"=[], "AO"=[], "Regs"=[], "DO"=[], "ALR"=[], "System"=[]}  # Enums
        n56 = call <userlib>:"Get Strings from Enum__ogtk.vi"("error in (no error)"=w186, "Enum"=w196) -> ("error out"=w210:errorcluster, "Enum Strings"=w183:string[])  [unwired: 6 in, 2 out]
        n57 = call <userlib>:"Get Strings from Enum__ogtk.vi"("error in (no error)"=w186, "Enum"=w195) -> ("error out"=w209:errorcluster, "Enum Strings"=w216:string[])  [unwired: 6 in, 2 out]
        n58 = call <userlib>:"Get Strings from Enum__ogtk.vi"("error in (no error)"=w186, "Enum"=w194) -> ("error out"=w208:errorcluster, "Enum Strings"=w215:string[])  [unwired: 6 in, 2 out]
        n59 = call <userlib>:"Get Strings from Enum__ogtk.vi"("error in (no error)"=w186, "Enum"=w193) -> ("error out"=w207:errorcluster, "Enum Strings"=w214:string[])  [unwired: 6 in, 2 out]
        n60 = call <userlib>:"Get Strings from Enum__ogtk.vi"("error in (no error)"=w186, "Enum"=w192) -> ("error out"=w206:errorcluster, "Enum Strings"=w213:string[])  [unwired: 6 in, 2 out]
        n61 = call <userlib>:"Get Strings from Enum__ogtk.vi"("error in (no error)"=w186, "Enum"=w191) -> ("error out"=w205:errorcluster, "Enum Strings"=w212:string[])  [unwired: 6 in, 2 out]
        n62 = call <userlib>:"Get Strings from Enum__ogtk.vi"("error in (no error)"=w186, "Enum"=w190) -> ("error out"=w200:errorcluster, "Enum Strings"=w182:string[])  [unwired: 6 in, 2 out]
        n63 = call <userlib>:"Get Strings from Enum__ogtk.vi"("error in (no error)"=w186, "Enum"=w189) -> ("error out"=w199:errorcluster, "Enum Strings"=w201:string[])  [unwired: 6 in, 2 out]
        n64 = call <userlib>:"Get Strings from Enum__ogtk.vi"("error in (no error)"=w186, "Enum"=w188) -> ("error out"=w198:errorcluster, "Enum Strings"=w211:string[])  [unwired: 6 in, 2 out]
        n65 = call <userlib>:"Get Strings from Enum__ogtk.vi"("error in (no error)"=w186, "Enum"=w187) -> ("error out"=w197:errorcluster)  [unwired: 6 in, 3 out]
        n66 = Bundle By Name(cluster=w217, "KFM"=w183, "PAR"=w216, "AI"=w215, "DI"=w214, "DI_fast"=w213, "AO"=w212, "Regs"=w182, "DO"=w201, "ALR"=w211, "System"=string[] []) -> (w219:T14)
        n67 = Array Size(array=w183) -> (size(s)=w185:i32)
        n68 = Array Size(array=w182) -> (size(s)=w184:i32)
        n69 = Merge Errors(w210, w209, w208, w207, w206, w205, w200, w199, w198, w197) -> (w204:errorcluster)
        n70 = Bundle By Name(cluster=w220, "N_KFMs"=w185, "N_regs"=w184, "Enums"=w219) -> (w218:T21)
      }
      frame "Read Reg param" {
        n71 = Unbundle By Name(w233) -> ("Enums.Regs"=w230:string[])
        n72 = Unbundle By Name(w233) -> ("system DB"=w228:T4)
        n73 = call <userlib>:"Get Strings from Enum__ogtk.vi"("error in (no error)"=w235, "Enum"=bronkhorstColumns."fcode" ("ParamColumns")) -> ("error out"=w225:errorcluster, "Enum Strings"=w224:string[])  [unwired: 6 in, 2 out]
        n74 = call "Get bronkhorst param from PGserver.vi"("conninfo"=w228, "error in (no error)"=w225, "RegParamColumns"=w224, "AIParamTable"="bronkhorst_1", "AIParameters"=w230) -> ("error out"=w234:errorcluster, "Names table"=w226:string[][], "Parameters table"=w227:dbl[][])  [unwired: 4 in]
        n75 = Bundle By Name(cluster=w231, "RegsParam"=w227, "Regs_Descriptions"=w226) -> (w232:T23)
      }
      frame "Connect to OPC" {
        n76 = disable-structure shown="SERVER==OPC" {
          disable-tunnel: w242 -> [w264 w270]
          disable-tunnel: [w263 w271] -> w240
          disable-tunnel: [w246 w270] -> w239
          disable-tunnel: w238 -> [w257 w271]
          disable-tunnel: w238 -> [w249 _]
          frame condition #0 (active) {
            w265 = TRUE  # trust any server
            # "1."
            n77 = Unbundle By Name(w249) -> ("Server.name"=w259:string, "Server.OPC port"=w255:string, "Server.security policy"=w245:T35)
            n78 = Concatenate Strings("opc.tcp://" ("server endpoint URL 2"), w259, ":" ("server endpoint URL 2"), w255) -> (w254:string)
            n79 = call <vilib>:"Connect.vi"("trust any server (F)"=w265, "error in (no error)"=w264, "security policy"=w245, "server endpoint URL"=w254) -> ("error out"=w267:errorcluster, "OPC UA client refnum out"=w268:T17)  [unwired: 5 in, 1 out]
            n80 = call <vilib>:"Create Subscription.vi"("error in (no error)"=w267, "publishing interval (1000 ms)"=100.0 ("update rate (1000 ms)"), "OPC UA client refnum in"=w268) -> ("error out"=w247:errorcluster, "OPC UA data change event"=w248:refnum<user-event>, "subscription ID out"=w261:T18, "OPC UA client refnum out"=w269:T17)  [unwired: 4 in, 1 out]
            n81 = call "OPC_server_param.vi"() -> ("Parameters"=w253:T36[])  [unwired: 11 in]
            n82 = call "Select OPC node IDs.vi"("OPC Params"=w253) -> ("parameters"=w250:T40, "requests"=w251:T19[], "node IDs"=w252:string[])  [unwired: 8 in]
            n83 = call <vilib>:"Add Monitored Data Nodes.vi"("monitoring parameters"=w250, "error in (no error)"=w247, "node IDs"=w252, "subscription ID in"=w261, "OPC UA client refnum in"=w269) -> ("error out"=w246:errorcluster, "OPC UA client refnum out"=w260:T17)  [unwired: 3 in, 2 out]
            n84 = Build Array(w261) -> (w262:T18[])
            n85 = Bundle By Name(cluster=w257, "OPC UA.data change event"=w248, "OPC UA.node IDs"=w252, "OPC UA.subscription IDs"=w262, "OPC UA.requests"=w251, "OPC UA.Client refnum"=w260) -> (w263:T21)
          }
          frame condition #1 {
          }
        }
      }
      frame "AI references" {
        n86 = Unbundle By Name(w278) -> ("Enums.AI"=w280:string[])
        n87 = Array Size(array=w280) -> (size(s)=w281:i32)
        n88 = for {
          N: w281 -> [_]
          tunnel: AI."GM1QN1_XQ01" ("AI_enum") -> [w289]
          tunnel: [w286] -> w274 mode=indexing
          tunnel: [w286] -> w272 mode=indexing if=w285
          i -> [w287]
          n89 = Coerce To Type(0:w287, 1:w289) -> (2:w288:T1)
          n90 = case shown="\"GM1QN1_XQ01\"" w288 {
            tunnel: [_ w291] -> w286
            tunnel: [_ TRUE] -> w285
            frame Default {
            }
            frame "GM1QN1_XQ01" {
              n91 = control-ref of="GM1QN1_XQ01"() -> (w291:refnum<vi>)
            }
          }
        }
        n92 = register-events(error in=w276, w272) -> (reference out=w273:refnum<event-registration>, error out=w275:errorcluster)  [unwired: 1 in]
        n93 = Bundle By Name(cluster=w278, "AI_refs"=w274, "AI_events"=w273) -> (w279:T21)
      }
      frame "AI reorder" {
        n94 = Unbundle By Name(w299) -> ("Enums.AI"=w292:string[], "OPC UA.Client refnum"=w294:T17)
        n95 = call-poly <vilib>:"Multiple Read.vi"("error in (no error)"=w301, "node IDs"=T6 ["ns=2;s=AI.AI_Names"] ("OPC UA.node IDs"), "OPC UA client refnum in"=w294) -> ("error out"=w300:errorcluster, "results"=w296:T42, "service status"=w295:T41)  [unwired: 5 in, 1 out]
        n96 = case shown="0..15" w295 {
          tunnel: w296 -> [_ w308]
          tunnel: w292 -> [_ w306]
          tunnel: [_ w305] -> w302
          frame 16.., Default {
          }
          frame 0..15 {
            n97 = Index Array(array=w308) -> (element=w309:T43)  [unwired: 1 in]
            n98 = Unbundle By Name(w309) -> ("values"=w307:string[])
            n99 = for {
              tunnel: w306 -> [w312] mode=indexing
              tunnel: w307 -> [w311]
              tunnel: [w310] -> w305 mode=indexing
              n100 = Search 1D Array(1D array=w311, element=w312) -> (index of element=w310:i32)  [unwired: 1 in]
            }
          }
        }
        n101 = Bundle By Name(cluster=w297, "AI_reorder_table"=w302) -> (w298:T23)
      }
      frame "AI Descriptions" {
        n102 = Unbundle By Name(w317) -> ("Enums.AI"=w322:string[], "system DB"=w320:T4)
        n103 = Unbundle By Name(w317) -> ("AI_refs"=w324:refnum<vi>[])
        n104 = call "Get AI param from PGserver sh2.vi"("conninfo"=w320, "error in (no error)"=w318, "AIParamTable"="fa_1", "AIParameters"=w322) -> ("error out"=w313:errorcluster, "Names table"=w319:string[][], "Parameters table"=w321:dbl[][])  [unwired: 5 in]
        n105 = for {
          tunnel: w319 -> [w336]
          tunnel: w324 -> [w334] mode=indexing
          i -> [w331]
          n106 = Not A Number/Path/Refnum?(number/path/refnum=w334) -> (NaN/Path/Refnum?=w335:bool)
          n107 = Index Array(array=w336, index (row) #1=w331, index (col) #1=2 ("disabled index (col)"), index (row) #2=w331, index (col) #2=3 ("disabled index (col)")) -> (element #1=w330:string, element #2=w328:string)
          n108 = Concatenate Strings(w330, "\r", w328) -> (w327:string)
          n109 = case shown="False" w335 {
            tunnel: w327 -> [w338 _]
            tunnel: w334 -> [w337 _]
            frame False {
              n110 = property on="Property Node" class="DigNum (strict)"(reference=w337, "TipStrip"=w338) -> ()  [unwired: 1 in, 2 out]
            }
            frame True {
            }
          }
        }
        n111 = Bundle By Name(cluster=w315, "AIP"=w321) -> (w316:T23)
        n112 = Bundle By Name(cluster=w317, "AI_Descriptions"=w319) -> (w314:T21)
      }
      frame "Read DI param" {
        n113 = disable-structure shown="SERVER==SHRV, Default" {
          disable-tunnel: w343 -> [w347 w362]
          disable-tunnel: [w346 w360] -> w342
          disable-tunnel: w339 -> [w346 w353]
          disable-tunnel: [w347 w351] -> w340
          disable-tunnel: w339 -> [_ w349]
          frame condition #0 (active) {
          }
          frame condition #1 {
            w348 = T44 {"Read Access"=enum."Allowed", "Write Access"=enum."None"} ("access")
            w357 = "ni.var.psp://" ("server endpoint URL 2")
            n114 = Unbundle By Name(w349) -> ("Server.name"=w356:string)
            n115 = Concatenate Strings(w357, w356, "/InputsVar/DI" ("server endpoint URL 2")) -> (w363:string)
            n116 = shared-variable-open ("AI_ref")(w363, w362, T8 {"DI"=[], "DI_State"=[], "DI_ALRState"=[]} ("DI"), w348) -> (w361:refnum<k21>, w359:errorcluster)
            n117 = Concatenate Strings(w357, w356, "/InputsVar/DI_fcode_full" ("server endpoint URL 2")) -> (w358:string)
            n118 = shared-variable-open ("AI_ref")(w358, w359, string[] [] ("AI"), w348) -> (w352:refnum<k21>, w351:errorcluster)
            n119 = Bundle By Name(cluster=w353, "AI_Descriptions"=w361, "DI_Descriptions"=w352) -> (w360:T21)
          }
        }
      }
      frame "Read ALR param" {
        n120 = Unbundle By Name(w368) -> ("ALR_State"=w374:T10)
        n121 = Unbundle By Name(w370) -> ("Enums.ALR"=w375:string[])
        n122 = Array Size(array=w375) -> (size(s)=w366:i32)
        n123 = call "ALR scada init.vi"("error in (no error)"=w371, "N_param"=w366, "ALR_State in"=w374) -> ("error out"=w372:errorcluster, "ALR_State out"=w373:T10)  [unwired: 7 in]
        n124 = disable-structure shown="SERVER==SHRV, Default" {
          disable-tunnel: w372 -> [w400 w404]
          disable-tunnel: [w399 w412] -> w377
          disable-tunnel: w370 -> [w398 w411]
          disable-tunnel: [w397 w401] -> w376
          disable-tunnel: w370 -> [_ w403]
          frame condition #0 {
            w385 = T44 {"Read Access"=enum."Allowed", "Write Access"=enum."None"} ("access")
            w384 = "ni.var.psp://" ("server endpoint URL 2")
            n125 = Unbundle By Name(w398) -> ("Server.name"=w383:string)
            n126 = Concatenate Strings(w384, w383, "/ALRVar/ALR_State" ("server endpoint URL 2")) -> (w395:string)
            n127 = shared-variable-open ("AI_ref")(w395, w400, T10 {"ALR not block"=[], "ALR"=[], "ALR blocked"=[], "ALR ON"=[], "code"=[], "level"=[], "t ms"=[], "ack state"=[], "color"=[]} ("ALR_State"), w385) -> (w394:refnum<k21>, w393:errorcluster)
            n128 = Concatenate Strings(w384, w383, "/ALRVar/ALR_Descriptions" ("server endpoint URL 2")) -> (w392:string)
            n129 = shared-variable-open ("AI_ref")(w392, w393, string[] [] ("ALR_Names"), w385) -> (w380:refnum<k21>, w386:errorcluster)
            n130 = Concatenate Strings(w384, w383, "/Var/Total" ("server endpoint URL 2")) -> (w388:string)
            n131 = shared-variable-open ("AI_ref")(w388, w386, 0.0 ("CPU_utilization"), w385) -> (w381:refnum<k21>, w397:errorcluster)
            n132 = Bundle By Name(cluster=w398, "ALR_Descriptions"=w394, "ALR_Descriptions_SHRV"=w380, "CPU_utilization"=w381) -> (w399:T21)
          }
          frame condition #1 (active) {
            n133 = Unbundle By Name(w403) -> ("OPC UA.Client refnum"=w407:T17)
            n134 = call-poly <vilib>:"Multiple Read.vi"("error in (no error)"=w404, "node IDs"=T6 ["ns=2;s=ALR.ALR_Descriptions"] ("OPC UA.node IDs"), "OPC UA client refnum in"=w407) -> ("error out"=w401:errorcluster, "results"=w409:T45)  [unwired: 5 in, 2 out]
            n135 = Index Array(array=w409) -> (element=w410:T46)  [unwired: 1 in]
            n136 = Unbundle By Name(w410) -> ("values"=w408:u8[][])
            n137 = for {
              tunnel: w408 -> [w417] mode=indexing
              tunnel: [w415] -> w402 mode=indexing
              tunnel: u8[] [0] ("unsigned byte array") -> [w413]
              n138 = Byte Array To String(unsigned byte array=w417) -> (string=w416:string)
              n139 = Byte Array To String(unsigned byte array=w413) -> (string=w414:string)
              n140 = Match Pattern(string=w416, regular expression=w414) -> (before substring=w415:string)  [unwired: 1 in, 3 out]
            }
            n141 = Bundle By Name(cluster=w411, "ALR_Descriptions"=w402) -> (w412:T21)
          }
        }
        n142 = Initialize Array("", w366) -> (w365:string[])
        n143 = Bundle By Name(cluster=w368, "ALR_State"=w373, "ALR_Names"=w365) -> (w369:T23)
      }
      frame "Read control param" {
        n144 = disable-structure shown="SERVER==SHRV, Default" {
          disable-tunnel: w422 -> [w426 w443]
          disable-tunnel: [w425 w442] -> w421
          disable-tunnel: w418 -> [w425 w439]
          disable-tunnel: [w426 _] -> w419
          disable-tunnel: w418 -> [_ w438]
          frame condition #0 (active) {
          }
          frame condition #1 {
            w427 = T47 {"Z_HSw"=0, "Z_HSetState"=enum."stop ready", "Y_HSw"=0, "Y_HSetState"=enum."hand", "SP"=0.0, "Y_H"=0.0, "Reset_ALR"=FALSE} ("ZY_control")
            w435 = T44 {"Read Access"=enum."Allowed", "Write Access"=enum."Allowed"} ("access")
            w434 = "ni.var.psp://" ("server endpoint URL 2")
            n145 = Unbundle By Name(w438) -> ("Server.name"=w433:string)
            n146 = Concatenate Strings(w434, w433, "/Var/EB2TB1_control" ("server endpoint URL 2")) -> (w444:string)
            n147 = shared-variable-open ("AI_ref")(w444, w443, w427, w435) -> (w430:refnum<k21>, w441:errorcluster)
            n148 = Concatenate Strings(w434, w433, "/Var/EB2TB2_control" ("server endpoint URL 2")) -> (w440:string)
            n149 = shared-variable-open ("AI_ref")(w440, w441, w427, w435) -> (w429:refnum<k21>, w436:errorcluster)
            n150 = Concatenate Strings(w434, w433, "/Var/EB2TB3_control" ("server endpoint URL 2")) -> (w437:string)
            n151 = shared-variable-open ("AI_ref")(w437, w436, w427, w435) -> (w428:refnum<k21>)  [unwired: 1 out]
            n152 = Bundle By Name(cluster=w439, "CPU_utilization"=w430, "AI_Descriptions"=w429, "ALR_Descriptions"=w428) -> (w442:T21)
          }
        }
      }
      frame "Read state param" {
        n153 = disable-structure shown="SERVER==SHRV, Default" {
          disable-tunnel: w450 -> [w454 w471]
          disable-tunnel: [w453 w470] -> w449
          disable-tunnel: w446 -> [w453 w467]
          disable-tunnel: [w454 _] -> w447
          disable-tunnel: w446 -> [_ w466]
          frame condition #0 (active) {
          }
          frame condition #1 {
            w455 = T50 {"Z"={"Z_Source"=enum."hand", "Z_SetState"=enum."stop ready", "Z_State"=enum."initialization", "Z_State_T"=0, "ZM_State"=enum."initialization", "ZM_State_T"=0, "ALR  L1"=FALSE, "ALR  L2"=FALSE, "HH_run"=0}, "Y"={"Y_Source"=enum."hand", "Y_SetState"=enum."hand", "SP_Set"=0.0, "SP"=0.0, "PV"=0.0, "Y_Set"=0.0, "Y"=0.0, "Y_State"={"code"=0, "visible"=FALSE, "color"=0}, "YB"=FALSE}, "ALR_Status"=[]} ("AI")
            w463 = T44 {"Read Access"=enum."Allowed", "Write Access"=enum."Allowed"} ("access")
            w462 = "ni.var.psp://" ("server endpoint URL 2")
            n154 = Unbundle By Name(w466) -> ("Server.name"=w461:string)
            n155 = Concatenate Strings(w462, w461, "/Var/EB2TB1_state" ("server endpoint URL 2")) -> (w472:string)
            n156 = shared-variable-open ("AI_ref")(w472, w471, w455, w463) -> (w458:refnum<k21>, w469:errorcluster)
            n157 = Concatenate Strings(w462, w461, "/Var/EB2TB2_state" ("server endpoint URL 2")) -> (w468:string)
            n158 = shared-variable-open ("AI_ref")(w468, w469, w455, w463) -> (w457:refnum<k21>, w464:errorcluster)
            n159 = Concatenate Strings(w462, w461, "/Var/EB2TB3_state" ("server endpoint URL 2")) -> (w465:string)
            n160 = shared-variable-open ("AI_ref")(w465, w464, w455, w463) -> (w456:refnum<k21>)  [unwired: 1 out]
            n161 = Bundle By Name(cluster=w467, "AI_refs"=w458, "DI_Descriptions"=w457, "EB2TB3_state"=w456) -> (w470:T21)
          }
        }
      }
      frame "Init ALR Listbox symbols" {
        w483 = T57 {"image type"=0, "image depth"=24, "image"=[153, 204, 51, 153, 204, 51, 153, 204, 51, 153, 204, 51, 153, 204, 51, 153, 204, 51, 153, 204, 51, 153, 204, 51, 153, 204, 51, 153, 204, 51, 153, 204, 51, 153, 204, 51, 153, 204, 51, 153, 204, 51, 153, 204, 51, 153, 204, 51, 153, 204, 51, 153, 204, 51, 153, 204, 51, 153, 204, 51, 153, 204, 51, 153, 204, 51, 153, 204, 51, 153, 204, 51, 153, 204, 51, 153, 204, 51, 153, 204, 51, 153, 204, 51, 153, 204, 51, 153, 204, 51, 153, 204, 51, 153, 204, 51, 153, 204, 51, 153, 204, 51, 153, 204, 51, 153, 204, 51, 255, 255, 255, 255, 255, 255, 153, 204, 51, 153, 204, 51, 153, 204, 51, 153, 204, 51, 153, 204, 51, 153, 204, 51, 153, 204, 51, 153, 204, 51, 153, 204, 51, 153, 204, 51, 153, 204, 51, 153, 204, 51, 153, 204, 51, 153, 204, 51, 153, 204, 51, 255, 255, 255, 255, 255, 255, 255, 255, 255, 153, 204, 51, 153, 204, 51, 153, 204, 51, 153, 204, 51, 153, 204, 51, 153, 204, 51, 153, 204, 51, 153, 204, 51, 153, 204, 51, 153, 204, 51, 153, 204, 51, 153, 204, 51, 153, 204, 51, 153, 204, 51, 153, 204, 51, 255, 255, 255, 255, 255, 255, 255, 255, 255, 153, 204, 51, 153, 204, 51, 153, 204, 51, 153, 204, 51, 153, 204, 51, 153, 204, 51, 153, 204, 51, 153, 204, 51, 153, 204, 51, 153, 204, 51, 153, 204, 51, 153, 204, 51, 153, 204, 51, 153, 204, 51, 153, 204, 51, 255, 255, 255, 255, 255, 255, 255, 255, 255, 153, 204, 51, 153, 204, 51, 153, 204, 51, 153, 204, 51, 153, 204, 51, 153, 204, 51, 153, 204, 51, 153, 204, 51, 153, 204, 51, 153, 204, 51, 153, 204, 51, 153, 204, 51, 153, 204, 51, 153, 204, 51, 153, 204, 51, 255, 255, 255, 255, 255, 255, 255, 255, 255, 153, 204, 51, 153, 204, 51, 153, 204, 51, 255, 255, 255, 153, 204, 51, 153, 204, 51, 153, 204, 51, 153, 204, 51, 153, 204, 51, 153, 204, 51, 153, 204, 51, 153, 204, 51, 153, 204, 51, 153, 204, 51, 153, 204, 51, 255, 255, 255, 255, 255, 255, 255, 255, 255, 153, 204, 51, 255, 255, 255, 255, 255, 255, 153, 204, 51, 153, 204, 51, 153, 204, 51, 153, 204, 51, 153, 204, 51, 153, 204, 51, 153, 204, 51, 153, 204, 51, 153, 204, 51, 153, 204, 51, 153, 204, 51, 153, 204, 51, 255, 255, 255, 255, 255, 255, 255, 255, 255, 255, 255, 255, 255, 255, 255, 255, 255, 255, 153, 204, 51, 153, 204, 51, 153, 204, 51, 153, 204, 51, 153, 204, 51, 153, 204, 51, 153, 204, 51, 153, 204, 51, 153, 204, 51, 153, 204, 51, 153, 204, 51, 153, 204, 51, 255, 255, 255, 255, 255, 255, 255, 255, 255, 255, 255, 255, 255, 255, 255, 153, 204, 51, 153, 204, 51, 153, 204, 51, 153, 204, 51, 153, 204, 51, 153, 204, 51, 153, 204, 51, 153, 204, 51, 153, 204, 51, 153, 204, 51, 153, 204, 51, 255, 255, 255, 255, 255, 255, 255, 255, 255, 255, 255, 255, 255, 255, 255, 255, 255, 255, 153, 204, 51, 153, 204, 51, 153, 204, 51, 153, 204, 51, 153, 204, 51, 153, 204, 51, 153, 204, 51, 153, 204, 51, 153, 204, 51, 153, 204, 51, 255, 255, 255, 255, 255, 255, 255, 255, 255, 255, 255, 255, 255, 255, 255, 255, 255, 255, 255, 255, 255, 255, 255, 255, 153, 204, 51, 153, 204, 51, 153, 204, 51, 153, 204, 51, 153, 204, 51, 153, 204, 51, 153, 204, 51, 153, 204, 51, 153, 204, 51, 153, 204, 51, 153, 204, 51, 255, 255, 255, 255, 255, 255, 255, 255, 255, 255, 255, 255, 255, 255, 255, 255, 255, 255, 153, 204, 51, 153, 204, 51, 153, 204, 51, 153, 204, 51, 153, 204, 51, 153, 204, 51, 153, 204, 51, 153, 204, 51, 153, 204, 51, 153, 204, 51, 153, 204, 51, 153, 204, 51, 153, 204, 51, 153, 204, 51, 255, 255, 255, 255, 255, 255, 255, 255, 255, 153, 204, 51, 153, 204, 51, 153, 204, 51, 153, 204, 51, 153, 204, 51, 153, 204, 51, 153, 204, 51, 153, 204, 51, 153, 204, 51, 153, 204, 51, 153, 204, 51, 153, 204, 51, 153, 204, 51, 153, 204, 51, 153, 204, 51, 153, 204, 51, 153, 204, 51, 153, 204, 51, 153, 204, 51, 153, 204, 51, 153, 204, 51, 153, 204, 51, 153, 204, 51, 153, 204, 51, 153, 204, 51, 153, 204, 51, 153, 204, 51, 153, 204, 51, 153, 204, 51, 153, 204, 51, 153, 204, 51, 153, 204, 51, 153, 204, 51, 153, 204, 51, 153, 204, 51, 153, 204, 51, 153, 204, 51, 153, 204, 51, 153, 204, 51, 153, 204, 51, 153, 204, 51, 153, 204, 51, 153, 204, 51, 153, 204, 51, 153, 204, 51, 153, 204, 51, 153, 204, 51, 153, 204, 51, 153, 204, 51, 153, 204, 51, 153, 204, 51, 153, 204, 51, 153, 204, 51, 153, 204, 51], "mask"=[], "colors"=[], "Rectangle"={"left"=0, "top"=0, "right"=17, "bottom"=17}}  # green down arrow
        w475 = T57 {"image type"=0, "image depth"=24, "image"=array[867 elements], "mask"=[], "colors"=[], "Rectangle"={"left"=0, "top"=0, "right"=17, "bottom"=17}}  # gray
        w485 = T57 {"image type"=0, "image depth"=24, "image"=[77, 77, 77, 77, 77, 77, 77, 77, 77, 77, 77, 77, 77, 77, 77, 77, 77, 77, 77, 77, 77, 77, 77, 77, 77, 77, 77, 77, 77, 77, 77, 77, 77, 77, 77, 77, 77, 77, 77, 77, 77, 77, 77, 77, 77, 77, 77, 77, 77, 77, 77, 77, 77, 77, 77, 77, 77, 77, 77, 77, 77, 77, 77, 77, 77, 77, 77, 77, 77, 77, 77, 77, 77, 77, 77, 77, 77, 77, 77, 77, 77, 77, 77, 77, 77, 77, 77, 77, 77, 77, 77, 77, 77, 77, 77, 77, 77, 77, 77, 77, 77, 77, 77, 77, 77, 77, 77, 77, 77, 77, 77, 77, 77, 77, 77, 77, 77, 77, 77, 77, 77, 77, 77, 77, 77, 77, 77, 77, 77, 77, 77, 77, 77, 77, 77, 77, 77, 77, 77, 77, 77, 77, 77, 77, 77, 77, 77, 77, 77, 77, 77, 77, 77, 77, 77, 77, 77, 77, 77, 77, 77, 77, 77, 77, 77, 77, 77, 77, 77, 77, 77, 77, 77, 77, 77, 77, 77, 77, 77, 77, 77, 77, 77, 77, 77, 77, 77, 77, 77, 77, 77, 77, 77, 77, 77, 77, 77, 77, 77, 77, 77, 77, 77, 77, 77, 77, 77, 77, 77, 77, 77, 77, 77, 77, 77, 77, 77, 77, 77, 77, 77, 77, 77, 77, 77, 77, 77, 77, 77, 77, 77, 77, 77, 77, 77, 77, 77, 77, 77, 77, 77, 77, 77, 77, 77, 77, 77, 77, 77, 77, 77, 77, 77, 77, 77, 77, 77, 77, 77, 77, 77, 77, 77, 77, 77, 77, 77, 77, 77, 77, 77, 77, 77, 77, 77, 77, 77, 77, 77, 77, 77, 77, 77, 77, 77, 77, 77, 77, 77, 77, 77, 77, 77, 77, 77, 77, 77, 77, 77, 77, 77, 77, 77, 77, 77, 77, 77, 77, 77, 77, 77, 77, 77, 77, 77, 77, 77, 77, 77, 77, 77, 77, 77, 77, 77, 77, 77, 77, 77, 77, 77, 77, 77, 77, 77, 77, 77, 77, 77, 77, 77, 77, 77, 77, 77, 77, 77, 77, 77, 77, 77, 77, 77, 77, 77, 77, 77, 77, 77, 77, 77, 77, 77, 77, 77, 77, 77, 77, 77, 77, 77, 77, 77, 77, 77, 77, 77, 77, 77, 77, 77, 77, 77, 77, 77, 77, 77, 77, 77, 77, 77, 77, 77, 77, 77, 77, 77, 77, 77, 77, 77, 77, 77, 77, 77, 77, 77, 77, 77, 77, 77, 77, 77, 77, 77, 77, 77, 77, 77, 77, 77, 77, 77, 77, 77, 77, 77, 77, 77, 77, 77, 77, 77, 77, 77, 77, 77, 77, 77, 77, 77, 77, 77, 77, 77, 77, 77, 77, 77, 77, 77, 77, 77, 77, 77, 77, 77, 77, 77, 77, 77, 77, 77, 77, 77, 77, 77, 77, 77, 77, 77, 77, 77, 77, 77, 77, 77, 77, 77, 77, 77, 77, 77, 77, 77, 77, 77, 77, 77, 77, 77, 77, 77, 77, 77, 77, 77, 77, 77, 77, 77, 77, 77, 77, 77, 77, 77, 77, 77, 77, 77, 77, 77, 77, 77, 77, 77, 77, 77, 77, 77, 77, 77, 77, 77, 77, 77, 77, 77, 77, 77, 77, 77, 77, 77, 77, 77, 77, 77, 77, 77, 77, 77, 77, 77, 77, 77, 77, 77, 77, 77, 77, 77, 77, 77, 77, 77, 77, 77, 77, 77, 77, 77, 77, 77, 77, 77, 77, 77, 77, 77, 77, 77, 77, 77, 77, 77, 77, 77, 77, 77, 77, 77, 77, 77, 77, 77, 77, 77, 77, 77, 77, 77, 77, 77, 77, 77, 77, 77, 77, 77, 77, 77, 77, 77, 77, 77, 77, 77, 77, 77, 77, 77, 77, 77, 77, 77, 77, 77, 77, 77, 77, 77, 77, 77, 77, 77, 77, 77, 77, 77, 77, 77, 77, 77, 77, 77, 77, 77, 77, 77, 77, 77, 77, 77, 77, 77, 77, 77, 77, 77, 77, 77, 77, 77, 77, 77, 77, 77, 77, 77, 77, 77, 77, 77, 77, 77, 77, 77, 77, 77, 77, 77, 77, 77, 77, 77, 77, 77, 77, 77, 77, 77, 77, 77, 77, 77, 77, 77, 77, 77, 77, 77, 77, 77, 77, 77, 77, 77, 77, 77, 77, 77, 77, 77, 77, 77, 77, 77, 77, 77, 77, 77, 77, 77, 77, 77, 77, 77, 77, 77, 77, 77, 77, 77, 77, 77, 77, 77, 77, 77, 77, 77, 77, 77, 77, 77, 77, 77, 77, 77, 77, 77, 77, 77, 77, 77, 77, 77, 77, 77, 77, 77, 77, 77, 77, 77, 77, 77, 77, 77, 77, 77, 77, 77, 77, 77, 77, 77, 77, 77, 77, 77, 77, 77, 77, 77, 77, 77, 77, 77, 77, 77, 77, 77, 77, 77, 77, 77, 77, 77, 77, 77, 77, 77, 77, 77, 77, 77, 77, 77, 77, 77, 77, 77, 77, 77, 77, 77, 77, 77, 77, 77, 77, 77, 77, 77, 77, 77, 77, 77, 77, 77, 77, 77, 77, 77, 77, 77, 77, 77, 77, 77, 77, 77, 77, 77, 77, 77, 77, 77, 77, 77, 77, 77, 77, 77, 77, 77, 77, 77, 77, 77, 77, 77, 77, 77, 77, 77, 77, 77, 77, 77, 77, 77, 77, 77], "mask"=[], "colors"=[], "Rectangle"={"left"=0, "top"=0, "right"=17, "bottom"=17}}  # brown
        w484 = T57 {"image type"=0, "image depth"=24, "image"=[77, 77, 77, 77, 77, 77, 77, 77, 77, 77, 77, 77, 77, 77, 77, 77, 77, 77, 77, 77, 77, 77, 77, 77, 77, 77, 77, 77, 77, 77, 77, 77, 77, 77, 77, 77, 77, 77, 77, 77, 77, 77, 77, 77, 77, 77, 77, 77, 77, 77, 77, 77, 77, 77, 77, 77, 77, 77, 77, 77, 77, 77, 77, 77, 77, 77, 77, 77, 77, 77, 77, 77, 77, 77, 77, 77, 77, 77, 77, 77, 77, 77, 77, 77, 77, 77, 77, 77, 77, 77, 77, 77, 77, 77, 77, 77, 77, 77, 77, 77, 77, 77, 77, 77, 77, 77, 77, 77, 77, 77, 77, 77, 77, 77, 77, 77, 77, 77, 77, 77, 77, 77, 77, 77, 77, 77, 77, 77, 77, 77, 77, 77, 77, 77, 77, 77, 77, 77, 77, 77, 77, 77, 77, 77, 77, 77, 77, 77, 77, 77, 77, 77, 77, 77, 77, 77, 77, 77, 77, 77, 77, 77, 77, 77, 77, 77, 77, 77, 77, 77, 77, 77, 77, 77, 77, 77, 77, 77, 77, 77, 195, 195, 195, 195, 195, 195, 255, 255, 255, 255, 255, 255, 255, 255, 255, 77, 77, 77, 77, 77, 77, 77, 77, 77, 77, 77, 77, 77, 77, 77, 77, 77, 77, 77, 77, 77, 77, 77, 77, 77, 77, 77, 77, 77, 77, 255, 255, 255, 255, 255, 255, 255, 255, 255, 255, 255, 255, 255, 255, 255, 255, 255, 255, 255, 255, 255, 77, 77, 77, 77, 77, 77, 77, 77, 77, 77, 77, 77, 77, 77, 77, 77, 77, 77, 77, 77, 77, 77, 77, 77, 77, 77, 77, 77, 77, 77, 77, 77, 77, 255, 255, 255, 255, 255, 255, 255, 255, 255, 255, 255, 255, 255, 255, 255, 221, 221, 221, 77, 77, 77, 77, 77, 77, 77, 77, 77, 77, 77, 77, 77, 77, 77, 77, 77, 77, 77, 77, 77, 77, 77, 77, 77, 77, 77, 77, 77, 77, 77, 77, 77, 77, 77, 77, 255, 255, 255, 255, 255, 255, 255, 255, 255, 255, 255, 255, 195, 195, 195, 77, 77, 77, 77, 77, 77, 77, 77, 77, 77, 77, 77, 77, 77, 77, 77, 77, 77, 77, 77, 77, 77, 77, 77, 77, 77, 77, 77, 77, 77, 77, 77, 77, 255, 255, 255, 255, 255, 255, 255, 255, 255, 255, 255, 255, 255, 255, 255, 127, 127, 127, 77, 77, 77, 77, 77, 77, 77, 77, 77, 77, 77, 77, 77, 77, 77, 77, 77, 77, 77, 77, 77, 77, 77, 77, 77, 77, 77, 77, 77, 77, 255, 255, 255, 255, 255, 255, 255, 255, 255, 77, 77, 77, 255, 255, 255, 255, 255, 255, 77, 77, 77, 77, 77, 77, 77, 77, 77, 77, 77, 77, 77, 77, 77, 77, 77, 77, 77, 77, 77, 77, 77, 77, 77, 77, 77, 77, 77, 77, 255, 255, 255, 255, 255, 255, 255, 255, 255, 77, 77, 77, 77, 77, 77, 77, 77, 77, 255, 255, 255, 77, 77, 77, 77, 77, 77, 77, 77, 77, 77, 77, 77, 77, 77, 77, 77, 77, 77, 77, 77, 77, 77, 77, 77, 77, 77, 77, 255, 255, 255, 255, 255, 255, 255, 255, 255, 77, 77, 77, 77, 77, 77, 77, 77, 77, 77, 77, 77, 77, 77, 77, 77, 77, 77, 77, 77, 77, 77, 77, 77, 77, 77, 77, 77, 77, 77, 77, 77, 77, 77, 77, 77, 77, 77, 77, 255, 255, 255, 255, 255, 255, 255, 255, 255, 77, 77, 77, 77, 77, 77, 77, 77, 77, 77, 77, 77, 77, 77, 77, 77, 77, 77, 77, 77, 77, 77, 77, 77, 77, 77, 77, 77, 77, 77, 77, 77, 77, 77, 77, 77, 77, 77, 77, 255, 255, 255, 255, 255, 255, 255, 255, 255, 77, 77, 77, 77, 77, 77, 77, 77, 77, 77, 77, 77, 77, 77, 77, 77, 77, 77, 77, 77, 77, 77, 77, 77, 77, 77, 77, 77, 77, 77, 77, 77, 77, 77, 77, 77, 77, 77, 77, 255, 255, 255, 255, 255, 255, 255, 255, 255, 77, 77, 77, 77, 77, 77, 77, 77, 77, 77, 77, 77, 77, 77, 77, 77, 77, 77, 77, 77, 77, 77, 77, 77, 77, 77, 77, 77, 77, 77, 77, 77, 77, 77, 77, 77, 77, 77, 77, 77, 77, 77, 255, 255, 255, 255, 255, 255, 77, 77, 77, 77, 77, 77, 77, 77, 77, 77, 77, 77, 77, 77, 77, 77, 77, 77, 77, 77, 77, 77, 77, 77, 77, 77, 77, 77, 77, 77, 77, 77, 77, 77, 77, 77, 77, 77, 77, 77, 77, 77, 77, 77, 77, 77, 77, 77, 77, 77, 77, 77, 77, 77, 77, 77, 77, 77, 77, 77, 77, 77, 77, 77, 77, 77, 77, 77, 77, 77, 77, 77, 77, 77, 77, 77, 77, 77, 77, 77, 77, 77, 77, 77, 77, 77, 77, 77, 77, 77, 77, 77, 77, 77, 77, 77, 77, 77, 77, 77, 77, 77, 77, 77, 77, 77, 77, 77, 77, 77, 77, 77, 77, 77, 77, 77, 77, 77, 77, 77, 77, 77, 77, 77, 77, 77, 77, 77, 77, 77, 77, 77, 77, 77, 77, 77, 77, 77, 77, 77, 77], "mask"=[], "colors"=[], "Rectangle"={"left"=0, "top"=0, "right"=17, "bottom"=17}}  # brown up arrow
        w482 = T57 {"image type"=0, "image depth"=24, "image"=[77, 77, 77, 77, 77, 77, 77, 77, 77, 77, 77, 77, 77, 77, 77, 77, 77, 77, 77, 77, 77, 77, 77, 77, 77, 77, 77, 77, 77, 77, 77, 77, 77, 77, 77, 77, 77, 77, 77, 77, 77, 77, 77, 77, 77, 77, 77, 77, 77, 77, 77, 77, 77, 77, 77, 77, 77, 77, 77, 77, 77, 77, 77, 77, 77, 77, 77, 77, 77, 77, 77, 77, 77, 77, 77, 77, 77, 77, 77, 77, 77, 77, 77, 77, 77, 77, 77, 249, 248, 249, 249, 244, 249, 77, 77, 77, 77, 77, 77, 77, 77, 77, 77, 77, 77, 77, 77, 77, 77, 77, 77, 77, 77, 77, 77, 77, 77, 77, 77, 77, 77, 77, 77, 77, 77, 77, 77, 77, 77, 77, 77, 77, 77, 77, 77, 255, 255, 255, 251, 250, 250, 255, 251, 255, 77, 77, 77, 77, 77, 77, 77, 77, 77, 77, 77, 77, 77, 77, 77, 77, 77, 77, 77, 77, 77, 77, 77, 77, 77, 77, 77, 77, 77, 77, 77, 77, 77, 77, 77, 77, 77, 77, 77, 77, 77, 77, 245, 244, 244, 243, 240, 241, 77, 77, 77, 77, 77, 77, 77, 77, 77, 77, 77, 77, 77, 77, 77, 77, 77, 77, 77, 77, 77, 77, 77, 77, 77, 77, 77, 77, 77, 77, 77, 77, 77, 77, 77, 77, 77, 77, 77, 77, 77, 77, 255, 251, 255, 245, 244, 244, 243, 240, 241, 77, 77, 77, 77, 77, 77, 77, 77, 77, 77, 77, 77, 77, 77, 77, 77, 77, 77, 77, 77, 77, 77, 77, 77, 77, 77, 77, 77, 77, 77, 77, 77, 77, 77, 77, 77, 77, 77, 77, 77, 77, 77, 244, 243, 243, 247, 241, 247, 170, 170, 170, 77, 77, 77, 77, 77, 77, 77, 77, 77, 77, 77, 77, 77, 77, 77, 77, 77, 77, 77, 77, 77, 77, 77, 77, 77, 77, 77, 77, 77, 77, 77, 77, 77, 77, 77, 77, 77, 77, 77, 250, 247, 250, 240, 235, 239, 247, 241, 247, 77, 77, 77, 77, 77, 77, 77, 77, 77, 77, 77, 77, 77, 77, 77, 77, 77, 77, 77, 77, 77, 77, 77, 77, 77, 77, 77, 77, 77, 77, 77, 77, 77, 77, 77, 77, 77, 77, 77, 77, 77, 77, 251, 245, 252, 245, 238, 245, 170, 170, 170, 77, 77, 77, 77, 77, 77, 77, 77, 77, 77, 77, 77, 77, 77, 77, 77, 77, 77, 77, 77, 77, 77, 77, 77, 77, 77, 77, 77, 77, 77, 77, 77, 77, 77, 77, 77, 77, 77, 77, 246, 243, 245, 239, 237, 238, 221, 222, 220, 77, 77, 77, 77, 77, 77, 77, 77, 77, 77, 77, 77, 77, 77, 77, 77, 77, 77, 77, 77, 77, 77, 77, 77, 255, 255, 255, 255, 255, 255, 255, 255, 255, 77, 77, 77, 77, 77, 77, 77, 77, 77, 239, 236, 238, 232, 230, 230, 77, 77, 77, 77, 77, 77, 77, 77, 77, 77, 77, 77, 77, 77, 77, 77, 77, 77, 77, 77, 77, 77, 77, 77, 77, 77, 77, 170, 170, 170, 255, 255, 255, 255, 255, 255, 77, 77, 77, 77, 77, 77, 249, 241, 249, 233, 231, 231, 237, 231, 236, 77, 77, 77, 77, 77, 77, 77, 77, 77, 77, 77, 77, 77, 77, 77, 77, 77, 77, 77, 77, 77, 77, 77, 77, 77, 77, 77, 77, 77, 77, 255, 255, 255, 255, 255, 255, 237, 243, 234, 221, 231, 218, 237, 234, 236, 230, 228, 228, 170, 170, 170, 77, 77, 77, 77, 77, 77, 77, 77, 77, 77, 77, 77, 77, 77, 77, 77, 77, 77, 77, 77, 77, 77, 77, 77, 77, 77, 77, 77, 77, 77, 77, 77, 77, 170, 170, 170, 234, 232, 232, 230, 229, 229, 229, 226, 227, 217, 216, 215, 77, 77, 77, 77, 77, 77, 77, 77, 77, 77, 77, 77, 77, 77, 77, 77, 77, 77, 77, 77, 77, 77, 77, 77, 77, 77, 77, 77, 77, 77, 77, 77, 77, 77, 77, 77, 170, 170, 170, 234, 232, 232, 230, 229, 229, 229, 226, 227, 77, 77, 77, 77, 77, 77, 77, 77, 77, 77, 77, 77, 77, 77, 77, 77, 77, 77, 77, 77, 77, 77, 77, 77, 77, 77, 77, 77, 77, 77, 77, 77, 77, 77, 77, 77, 77, 77, 77, 77, 77, 77, 237, 232, 236, 234, 229, 233, 170, 170, 170, 77, 77, 77, 77, 77, 77, 77, 77, 77, 77, 77, 77, 77, 77, 77, 77, 77, 77, 77, 77, 77, 77, 77, 77, 77, 77, 77, 77, 77, 77, 77, 77, 77, 77, 77, 77, 77, 77, 77, 77, 77, 77, 77, 77, 77, 77, 77, 77, 77, 77, 77, 77, 77, 77, 77, 77, 77, 77, 77, 77, 77, 77, 77, 77, 77, 77, 77, 77, 77, 77, 77, 77, 77, 77, 77, 77, 77, 77, 77, 77, 77, 77, 77, 77, 77, 77, 77, 77, 77, 77, 77, 77, 77, 77, 77, 77, 77, 77, 77, 77, 77, 77, 77, 77, 77, 77, 77, 77, 77, 77, 77, 77, 77, 77, 77, 77, 77, 77, 77, 77, 77, 77, 77, 77, 77, 77, 77, 77, 77], "mask"=[], "colors"=[], "Rectangle"={"left"=0, "top"=0, "right"=17, "bottom"=17}}  # brown ok
        w476 = T57 {"image type"=0, "image depth"=24, "image"=[77, 77, 77, 77, 77, 77, 77, 77, 77, 77, 77, 77, 77, 77, 77, 77, 77, 77, 77, 77, 77, 77, 77, 77, 77, 77, 77, 77, 77, 77, 77, 77, 77, 77, 77, 77, 77, 77, 77, 77, 77, 77, 77, 77, 77, 77, 77, 77, 77, 77, 77, 77, 77, 77, 77, 77, 77, 77, 77, 77, 77, 77, 77, 77, 77, 77, 77, 77, 77, 77, 77, 77, 77, 77, 77, 77, 77, 77, 77, 77, 77, 77, 77, 77, 77, 77, 77, 77, 77, 77, 77, 77, 77, 77, 77, 77, 77, 77, 77, 77, 77, 77, 77, 77, 77, 77, 77, 77, 77, 77, 77, 77, 77, 77, 77, 77, 77, 77, 77, 77, 77, 77, 77, 77, 77, 77, 77, 77, 77, 77, 77, 77, 77, 77, 77, 77, 77, 77, 77, 77, 77, 153, 204, 51, 153, 204, 51, 77, 77, 77, 77, 77, 77, 77, 77, 77, 77, 77, 77, 77, 77, 77, 77, 77, 77, 77, 77, 77, 77, 77, 77, 77, 77, 77, 77, 77, 77, 77, 77, 77, 77, 77, 77, 77, 77, 77, 77, 77, 77, 153, 204, 51, 153, 204, 51, 153, 204, 51, 77, 77, 77, 77, 77, 77, 77, 77, 77, 77, 77, 77, 77, 77, 77, 77, 77, 77, 77, 77, 77, 77, 77, 77, 77, 77, 77, 77, 77, 77, 77, 77, 77, 77, 77, 77, 77, 77, 77, 77, 77, 77, 153, 204, 51, 153, 204, 51, 99, 156, 0, 77, 77, 77, 77, 77, 77, 77, 77, 77, 77, 77, 77, 77, 77, 77, 77, 77, 77, 77, 77, 77, 77, 77, 77, 77, 77, 77, 77, 77, 77, 77, 77, 77, 77, 77, 77, 77, 77, 77, 153, 204, 51, 153, 204, 51, 153, 204, 51, 77, 77, 77, 77, 77, 77, 77, 77, 77, 77, 77, 77, 77, 77, 77, 77, 77, 77, 77, 77, 77, 77, 77, 77, 77, 77, 77, 77, 77, 77, 77, 77, 77, 77, 77, 77, 77, 77, 77, 77, 77, 77, 153, 204, 51, 153, 204, 51, 99, 156, 0, 77, 77, 77, 77, 77, 77, 77, 77, 77, 77, 77, 77, 77, 77, 77, 77, 77, 77, 77, 77, 77, 77, 77, 77, 77, 77, 77, 77, 77, 77, 77, 77, 77, 77, 77, 77, 77, 77, 77, 153, 204, 51, 153, 204, 51, 153, 204, 51, 77, 77, 77, 77, 77, 77, 77, 77, 77, 77, 77, 77, 77, 77, 77, 77, 77, 77, 77, 77, 77, 77, 77, 77, 77, 77, 77, 77, 77, 77, 77, 77, 77, 77, 77, 77, 77, 77, 77, 77, 77, 77, 153, 204, 51, 153, 204, 51, 99, 156, 0, 77, 77, 77, 77, 77, 77, 77, 77, 77, 77, 77, 77, 77, 77, 77, 77, 77, 77, 77, 77, 77, 77, 77, 77, 77, 77, 77, 77, 77, 77, 77, 77, 77, 77, 77, 77, 77, 77, 77, 153, 204, 51, 153, 204, 51, 153, 204, 51, 77, 77, 77, 77, 77, 77, 77, 77, 77, 77, 77, 77, 77, 77, 77, 77, 77, 77, 77, 77, 77, 77, 77, 77, 153, 204, 51, 153, 204, 51, 153, 204, 51, 77, 77, 77, 77, 77, 77, 77, 77, 77, 153, 204, 51, 153, 204, 51, 99, 156, 0, 77, 77, 77, 77, 77, 77, 77, 77, 77, 77, 77, 77, 77, 77, 77, 77, 77, 77, 77, 77, 77, 77, 77, 77, 99, 156, 0, 153, 204, 51, 153, 204, 51, 77, 77, 77, 77, 77, 77, 153, 204, 51, 153, 204, 51, 153, 204, 51, 77, 77, 77, 77, 77, 77, 77, 77, 77, 77, 77, 77, 77, 77, 77, 77, 77, 77, 77, 77, 77, 77, 77, 77, 77, 77, 77, 77, 77, 77, 153, 204, 51, 153, 204, 51, 153, 204, 51, 153, 204, 51, 153, 204, 51, 153, 204, 51, 99, 156, 0, 77, 77, 77, 77, 77, 77, 77, 77, 77, 77, 77, 77, 77, 77, 77, 77, 77, 77, 77, 77, 77, 77, 77, 77, 77, 77, 77, 77, 77, 77, 77, 77, 77, 99, 156, 0, 153, 204, 51, 153, 204, 51, 153, 204, 51, 99, 156, 0, 77, 77, 77, 77, 77, 77, 77, 77, 77, 77, 77, 77, 77, 77, 77, 77, 77, 77, 77, 77, 77, 77, 77, 77, 77, 77, 77, 77, 77, 77, 77, 77, 77, 77, 77, 77, 99, 156, 0, 153, 204, 51, 153, 204, 51, 153, 204, 51, 77, 77, 77, 77, 77, 77, 77, 77, 77, 77, 77, 77, 77, 77, 77, 77, 77, 77, 77, 77, 77, 77, 77, 77, 77, 77, 77, 77, 77, 77, 77, 77, 77, 77, 77, 77, 77, 77, 77, 77, 77, 77, 153, 204, 51, 153, 204, 51, 99, 156, 0, 77, 77, 77, 77, 77, 77, 77, 77, 77, 77, 77, 77, 77, 77, 77, 77, 77, 77, 77, 77, 77, 77, 77, 77, 77, 77, 77, 77, 77, 77, 77, 77, 77, 77, 77, 77, 77, 77, 77, 77, 77, 77, 77, 77, 77, 77, 77, 77, 77, 77, 77, 77, 77, 77, 77, 77, 77, 77, 77, 77, 77, 77, 77, 77, 77, 77, 77, 77, 77, 77, 77, 77, 77, 77, 77], "mask"=[], "colors"=[], "Rectangle"={"left"=0, "top"=0, "right"=17, "bottom"=17}}  # brown ok green down
        w477 = T57 {"image type"=0, "image depth"=24, "image"=[77, 77, 77, 77, 77, 77, 77, 77, 77, 77, 77, 77, 77, 77, 77, 77, 77, 77, 77, 77, 77, 77, 77, 77, 77, 77, 77, 77, 77, 77, 77, 77, 77, 77, 77, 77, 77, 77, 77, 77, 77, 77, 77, 77, 77, 77, 77, 77, 77, 77, 77, 77, 77, 77, 77, 77, 77, 77, 77, 77, 77, 77, 77, 77, 77, 77, 77, 77, 77, 77, 77, 77, 77, 77, 77, 77, 77, 77, 77, 77, 77, 77, 77, 77, 77, 77, 77, 77, 77, 77, 77, 77, 77, 77, 77, 77, 77, 77, 77, 77, 77, 77, 77, 77, 77, 77, 77, 77, 77, 77, 77, 77, 77, 77, 77, 77, 77, 77, 77, 77, 77, 77, 77, 77, 77, 77, 77, 77, 77, 77, 77, 77, 77, 77, 77, 77, 77, 77, 77, 77, 77, 249, 248, 249, 249, 244, 249, 77, 77, 77, 77, 77, 77, 77, 77, 77, 77, 77, 77, 77, 77, 77, 77, 77, 77, 77, 77, 77, 77, 77, 77, 77, 77, 77, 77, 77, 77, 77, 77, 77, 77, 77, 77, 77, 77, 77, 77, 77, 77, 255, 255, 255, 251, 250, 250, 255, 251, 255, 77, 77, 77, 77, 77, 77, 77, 77, 77, 77, 77, 77, 77, 77, 77, 77, 77, 77, 77, 77, 77, 77, 77, 77, 77, 77, 77, 77, 77, 77, 77, 77, 77, 77, 77, 77, 77, 77, 77, 77, 77, 77, 245, 244, 244, 243, 240, 241, 77, 77, 77, 77, 77, 77, 77, 77, 77, 77, 77, 77, 77, 77, 77, 77, 77, 77, 77, 77, 77, 77, 77, 77, 77, 77, 77, 77, 77, 77, 77, 77, 77, 77, 77, 77, 77, 77, 77, 77, 77, 77, 255, 251, 255, 245, 244, 244, 243, 240, 241, 77, 77, 77, 77, 77, 77, 77, 77, 77, 77, 77, 77, 77, 77, 77, 77, 77, 77, 77, 77, 77, 77, 77, 77, 77, 77, 77, 77, 77, 77, 77, 77, 77, 77, 77, 77, 77, 77, 77, 77, 77, 77, 244, 243, 243, 247, 241, 247, 170, 170, 170, 77, 77, 77, 77, 77, 77, 77, 77, 77, 77, 77, 77, 77, 77, 77, 77, 77, 77, 77, 77, 77, 77, 77, 77, 77, 77, 77, 77, 77, 77, 77, 77, 77, 77, 77, 77, 77, 77, 77, 250, 247, 250, 240, 235, 239, 247, 241, 247, 77, 77, 77, 77, 77, 77, 77, 77, 77, 77, 77, 77, 77, 77, 77, 77, 77, 77, 77, 77, 77, 77, 77, 77, 77, 77, 77, 77, 77, 77, 77, 77, 77, 77, 77, 77, 77, 77, 77, 77, 77, 77, 251, 245, 252, 245, 238, 245, 170, 170, 170, 77, 77, 77, 77, 77, 77, 77, 77, 77, 77, 77, 77, 77, 77, 77, 77, 77, 77, 77, 77, 77, 77, 77, 77, 77, 77, 77, 77, 77, 77, 77, 77, 77, 77, 77, 77, 77, 77, 77, 246, 243, 245, 239, 237, 238, 221, 222, 220, 77, 77, 77, 77, 77, 77, 77, 77, 77, 77, 77, 77, 77, 77, 77, 77, 77, 77, 77, 77, 77, 77, 77, 77, 255, 255, 255, 255, 255, 255, 255, 255, 255, 77, 77, 77, 77, 77, 77, 77, 77, 77, 239, 236, 238, 232, 230, 230, 77, 77, 77, 77, 77, 77, 77, 77, 77, 77, 77, 77, 77, 77, 77, 77, 77, 77, 77, 77, 77, 77, 77, 77, 77, 77, 77, 170, 170, 170, 255, 255, 255, 255, 255, 255, 77, 77, 77, 77, 77, 77, 249, 241, 249, 233, 231, 231, 237, 231, 236, 77, 77, 77, 77, 77, 77, 77, 77, 77, 77, 77, 77, 77, 77, 77, 77, 77, 77, 77, 77, 77, 77, 77, 77, 77, 77, 77, 77, 77, 77, 255, 255, 255, 255, 255, 255, 237, 243, 234, 221, 231, 218, 237, 234, 236, 230, 228, 228, 170, 170, 170, 77, 77, 77, 77, 77, 77, 77, 77, 77, 77, 77, 77, 77, 77, 77, 77, 77, 77, 77, 77, 77, 77, 77, 77, 77, 77, 77, 77, 77, 77, 77, 77, 77, 170, 170, 170, 234, 232, 232, 230, 229, 229, 229, 226, 227, 217, 216, 215, 77, 77, 77, 77, 77, 77, 77, 77, 77, 77, 77, 77, 77, 77, 77, 77, 77, 77, 77, 77, 77, 77, 77, 77, 77, 77, 77, 77, 77, 77, 77, 77, 77, 77, 77, 77, 170, 170, 170, 234, 232, 232, 230, 229, 229, 229, 226, 227, 77, 77, 77, 77, 77, 77, 77, 77, 77, 77, 77, 77, 77, 77, 77, 77, 77, 77, 77, 77, 77, 77, 77, 77, 77, 77, 77, 77, 77, 77, 77, 77, 77, 77, 77, 77, 77, 77, 77, 77, 77, 77, 237, 232, 236, 234, 229, 233, 170, 170, 170, 77, 77, 77, 77, 77, 77, 77, 77, 77, 77, 77, 77, 77, 77, 77, 77, 77, 77, 77, 77, 77, 77, 77, 77, 77, 77, 77, 77, 77, 77, 77, 77, 77, 77, 77, 77, 77, 77, 77, 77, 77, 77, 77, 77, 77, 77, 77, 77, 77, 77, 77, 77, 77, 77, 77, 77, 77, 77, 77, 77, 77, 77, 77, 77, 77, 77, 77, 77, 77, 77, 77, 77, 77, 77, 77], "mask"=[], "colors"=[], "Rectangle"={"left"=0, "top"=0, "right"=17, "bottom"=17}}  # brown ok down
        w481 = T57 {"image type"=0, "image depth"=24, "image"=[18, 179, 255, 18, 179, 255, 18, 179, 255, 18, 179, 255, 18, 179, 255, 18, 179, 255, 18, 179, 255, 18, 179, 255, 18, 179, 255, 18, 179, 255, 18, 179, 255, 18, 179, 255, 18, 179, 255, 18, 179, 255, 18, 179, 255, 18, 179, 255, 18, 179, 255, 18, 179, 255, 18, 179, 255, 18, 179, 255, 18, 179, 255, 18, 179, 255, 18, 179, 255, 18, 179, 255, 18, 179, 255, 18, 179, 255, 18, 179, 255, 18, 179, 255, 18, 179, 255, 18, 179, 255, 18, 179, 255, 18, 179, 255, 18, 179, 255, 18, 179, 255, 18, 179, 255, 18, 179, 255, 18, 179, 255, 18, 179, 255, 18, 179, 255, 18, 179, 255, 18, 179, 255, 18, 179, 255, 18, 179, 255, 18, 179, 255, 18, 179, 255, 18, 179, 255, 18, 179, 255, 18, 179, 255, 18, 179, 255, 18, 179, 255, 18, 179, 255, 18, 179, 255, 18, 179, 255, 18, 179, 255, 18, 179, 255, 18, 179, 255, 18, 179, 255, 18, 179, 255, 18, 179, 255, 18, 179, 255, 18, 179, 255, 18, 179, 255, 18, 179, 255, 18, 179, 255, 18, 179, 255, 18, 179, 255, 18, 179, 255, 18, 179, 255, 18, 179, 255, 18, 179, 255, 18, 179, 255, 18, 179, 255, 18, 179, 255, 18, 179, 255, 18, 179, 255, 18, 179, 255, 18, 179, 255, 18, 179, 255, 18, 179, 255, 18, 179, 255, 18, 179, 255, 18, 179, 255, 18, 179, 255, 18, 179, 255, 18, 179, 255, 18, 179, 255, 18, 179, 255, 18, 179, 255, 18, 179, 255, 18, 179, 255, 18, 179, 255, 18, 179, 255, 18, 179, 255, 18, 179, 255, 18, 179, 255, 18, 179, 255, 18, 179, 255, 18, 179, 255, 18, 179, 255, 18, 179, 255, 18, 179, 255, 18, 179, 255, 18, 179, 255, 18, 179, 255, 18, 179, 255, 18, 179, 255, 18, 179, 255, 18, 179, 255, 18, 179, 255, 18, 179, 255, 18, 179, 255, 18, 179, 255, 18, 179, 255, 18, 179, 255, 18, 179, 255, 18, 179, 255, 18, 179, 255, 18, 179, 255, 18, 179, 255, 18, 179, 255, 18, 179, 255, 18, 179, 255, 18, 179, 255, 18, 179, 255, 18, 179, 255, 18, 179, 255, 18, 179, 255, 18, 179, 255, 18, 179, 255, 18, 179, 255, 18, 179, 255, 18, 179, 255, 18, 179, 255, 18, 179, 255, 18, 179, 255, 18, 179, 255, 18, 179, 255, 18, 179, 255, 18, 179, 255, 18, 179, 255, 18, 179, 255, 18, 179, 255, 18, 179, 255, 18, 179, 255, 18, 179, 255, 18, 179, 255, 18, 179, 255, 18, 179, 255, 18, 179, 255, 18, 179, 255, 18, 179, 255, 18, 179, 255, 18, 179, 255, 18, 179, 255, 18, 179, 255, 18, 179, 255, 18, 179, 255, 18, 179, 255, 18, 179, 255, 18, 179, 255, 18, 179, 255, 18, 179, 255, 18, 179, 255, 18, 179, 255, 18, 179, 255, 18, 179, 255, 18, 179, 255, 18, 179, 255, 18, 179, 255, 18, 179, 255, 18, 179, 255, 18, 179, 255, 18, 179, 255, 18, 179, 255, 18, 179, 255, 18, 179, 255, 18, 179, 255, 18, 179, 255, 18, 179, 255, 18, 179, 255, 18, 179, 255, 18, 179, 255, 18, 179, 255, 18, 179, 255, 18, 179, 255, 18, 179, 255, 18, 179, 255, 18, 179, 255, 18, 179, 255, 18, 179, 255, 18, 179, 255, 18, 179, 255, 18, 179, 255, 18, 179, 255, 18, 179, 255, 18, 179, 255, 18, 179, 255, 18, 179, 255, 18, 179, 255, 18, 179, 255, 18, 179, 255, 18, 179, 255, 18, 179, 255, 18, 179, 255, 18, 179, 255, 18, 179, 255, 18, 179, 255, 18, 179, 255, 18, 179, 255, 18, 179, 255, 18, 179, 255, 18, 179, 255, 18, 179, 255, 18, 179, 255, 18, 179, 255, 18, 179, 255, 18, 179, 255, 18, 179, 255, 18, 179, 255, 18, 179, 255, 18, 179, 255, 18, 179, 255, 18, 179, 255, 18, 179, 255, 18, 179, 255, 18, 179, 255, 18, 179, 255, 18, 179, 255, 18, 179, 255, 18, 179, 255, 18, 179, 255, 18, 179, 255, 18, 179, 255, 18, 179, 255, 18, 179, 255, 18, 179, 255, 18, 179, 255, 18, 179, 255, 18, 179, 255, 18, 179, 255, 18, 179, 255, 18, 179, 255, 18, 179, 255, 18, 179, 255, 18, 179, 255, 18, 179, 255, 18, 179, 255, 18, 179, 255, 18, 179, 255, 18, 179, 255, 18, 179, 255, 18, 179, 255, 18, 179, 255, 18, 179, 255, 18, 179, 255, 18, 179, 255, 18, 179, 255, 18, 179, 255, 18, 179, 255, 18, 179, 255, 18, 179, 255, 18, 179, 255, 18, 179, 255, 18, 179, 255, 18, 179, 255, 18, 179, 255, 18, 179, 255, 18, 179, 255, 18, 179, 255, 18, 179, 255, 18, 179, 255, 18, 179, 255, 18, 179, 255, 18, 179, 255, 18, 179, 255, 18, 179, 255, 18, 179, 255, 18, 179, 255, 18, 179, 255, 18, 179, 255, 18, 179, 255, 18, 179, 255, 18, 179, 255, 18, 179, 255, 18, 179, 255, 18, 179, 255, 18, 179, 255, 18, 179, 255, 18, 179, 255], "mask"=[], "colors"=[], "Rectangle"={"left"=0, "top"=0, "right"=17, "bottom"=17}}  # blue
        w486 = T57 {"image type"=0, "image depth"=0, "image"=[], "mask"=[], "colors"=[], "Rectangle"={"left"=0, "top"=0, "right"=0, "bottom"=0}}  # element
        w480 = T57 {"image type"=0, "image depth"=24, "image"=[18, 179, 255, 18, 179, 255, 18, 179, 255, 18, 179, 255, 18, 179, 255, 18, 179, 255, 18, 179, 255, 18, 179, 255, 18, 179, 255, 18, 179, 255, 18, 179, 255, 18, 179, 255, 18, 179, 255, 18, 179, 255, 18, 179, 255, 18, 179, 255, 18, 179, 255, 18, 179, 255, 18, 179, 255, 18, 179, 255, 18, 179, 255, 18, 179, 255, 18, 179, 255, 18, 179, 255, 18, 179, 255, 18, 179, 255, 18, 179, 255, 18, 179, 255, 18, 179, 255, 18, 179, 255, 18, 179, 255, 18, 179, 255, 18, 179, 255, 18, 179, 255, 18, 179, 255, 18, 179, 255, 18, 179, 255, 18, 179, 255, 18, 179, 255, 18, 179, 255, 18, 179, 255, 18, 179, 255, 18, 179, 255, 18, 179, 255, 18, 179, 255, 18, 179, 255, 18, 179, 255, 18, 179, 255, 18, 179, 255, 18, 179, 255, 18, 179, 255, 18, 179, 255, 18, 179, 255, 18, 179, 255, 18, 179, 255, 18, 179, 255, 18, 179, 255, 18, 179, 255, 18, 179, 255, 18, 179, 255, 53, 189, 255, 98, 204, 255, 255, 255, 255, 255, 255, 255, 255, 255, 255, 18, 179, 255, 18, 179, 255, 18, 179, 255, 18, 179, 255, 18, 179, 255, 18, 179, 255, 18, 179, 255, 18, 179, 255, 18, 179, 255, 18, 179, 255, 255, 255, 255, 255, 255, 255, 255, 255, 255, 255, 255, 255, 255, 255, 255, 255, 255, 255, 255, 255, 255, 18, 179, 255, 18, 179, 255, 18, 179, 255, 18, 179, 255, 18, 179, 255, 18, 179, 255, 18, 179, 255, 18, 179, 255, 18, 179, 255, 18, 179, 255, 18, 179, 255, 255, 255, 255, 255, 255, 255, 255, 255, 255, 255, 255, 255, 255, 255, 255, 255, 255, 255, 18, 179, 255, 18, 179, 255, 18, 179, 255, 18, 179, 255, 18, 179, 255, 18, 179, 255, 18, 179, 255, 18, 179, 255, 18, 179, 255, 18, 179, 255, 18, 179, 255, 18, 179, 255, 255, 255, 255, 255, 255, 255, 255, 255, 255, 255, 255, 255, 98, 204, 255, 18, 179, 255, 18, 179, 255, 18, 179, 255, 18, 179, 255, 18, 179, 255, 18, 179, 255, 18, 179, 255, 18, 179, 255, 18, 179, 255, 18, 179, 255, 18, 179, 255, 255, 255, 255, 255, 255, 255, 255, 255, 255, 255, 255, 255, 255, 255, 255, 53, 189, 255, 18, 179, 255, 18, 179, 255, 18, 179, 255, 18, 179, 255, 18, 179, 255, 18, 179, 255, 18, 179, 255, 18, 179, 255, 18, 179, 255, 18, 179, 255, 255, 255, 255, 255, 255, 255, 255, 255, 255, 18, 179, 255, 255, 255, 255, 255, 255, 255, 18, 179, 255, 18, 179, 255, 18, 179, 255, 18, 179, 255, 18, 179, 255, 18, 179, 255, 18, 179, 255, 18, 179, 255, 18, 179, 255, 18, 179, 255, 255, 255, 255, 255, 255, 255, 255, 255, 255, 18, 179, 255, 18, 179, 255, 18, 179, 255, 255, 255, 255, 18, 179, 255, 18, 179, 255, 18, 179, 255, 18, 179, 255, 18, 179, 255, 18, 179, 255, 18, 179, 255, 18, 179, 255, 18, 179, 255, 255, 255, 255, 255, 255, 255, 255, 255, 255, 18, 179, 255, 18, 179, 255, 18, 179, 255, 18, 179, 255, 18, 179, 255, 18, 179, 255, 18, 179, 255, 18, 179, 255, 18, 179, 255, 18, 179, 255, 18, 179, 255, 18, 179, 255, 18, 179, 255, 255, 255, 255, 255, 255, 255, 255, 255, 255, 18, 179, 255, 18, 179, 255, 18, 179, 255, 18, 179, 255, 18, 179, 255, 18, 179, 255, 18, 179, 255, 18, 179, 255, 18, 179, 255, 18, 179, 255, 18, 179, 255, 18, 179, 255, 18, 179, 255, 255, 255, 255, 255, 255, 255, 255, 255, 255, 18, 179, 255, 18, 179, 255, 18, 179, 255, 18, 179, 255, 18, 179, 255, 18, 179, 255, 18, 179, 255, 18, 179, 255, 18, 179, 255, 18, 179, 255, 18, 179, 255, 18, 179, 255, 18, 179, 255, 255, 255, 255, 255, 255, 255, 255, 255, 255, 18, 179, 255, 18, 179, 255, 18, 179, 255, 18, 179, 255, 18, 179, 255, 18, 179, 255, 18, 179, 255, 18, 179, 255, 18, 179, 255, 18, 179, 255, 18, 179, 255, 18, 179, 255, 18, 179, 255, 18, 179, 255, 255, 255, 255, 255, 255, 255, 18, 179, 255, 18, 179, 255, 18, 179, 255, 18, 179, 255, 18, 179, 255, 18, 179, 255, 18, 179, 255, 18, 179, 255, 18, 179, 255, 18, 179, 255, 18, 179, 255, 18, 179, 255, 18, 179, 255, 18, 179, 255, 18, 179, 255, 18, 179, 255, 18, 179, 255, 18, 179, 255, 18, 179, 255, 18, 179, 255, 18, 179, 255, 18, 179, 255, 18, 179, 255, 18, 179, 255, 18, 179, 255, 18, 179, 255, 18, 179, 255, 18, 179, 255, 18, 179, 255, 18, 179, 255, 18, 179, 255, 18, 179, 255, 18, 179, 255, 18, 179, 255, 18, 179, 255, 18, 179, 255, 18, 179, 255, 18, 179, 255, 18, 179, 255, 18, 179, 255, 18, 179, 255, 18, 179, 255, 18, 179, 255, 18, 179, 255, 18, 179, 255, 18, 179, 255, 18, 179, 255], "mask"=[], "colors"=[], "Rectangle"={"left"=0, "top"=0, "right"=17, "bottom"=17}}  # blue up arrow
        w478 = T57 {"image type"=0, "image depth"=24, "image"=[18, 179, 255, 18, 179, 255, 18, 179, 255, 18, 179, 255, 18, 179, 255, 18, 179, 255, 18, 179, 255, 18, 179, 255, 18, 179, 255, 18, 179, 255, 18, 179, 255, 18, 179, 255, 18, 179, 255, 18, 179, 255, 18, 179, 255, 18, 179, 255, 18, 179, 255, 18, 179, 255, 18, 179, 255, 18, 179, 255, 18, 179, 255, 18, 179, 255, 18, 179, 255, 18, 179, 255, 18, 179, 255, 18, 179, 255, 18, 179, 255, 18, 179, 255, 18, 179, 255, 18, 179, 255, 18, 179, 255, 18, 179, 255, 18, 179, 255, 18, 179, 255, 18, 179, 255, 18, 179, 255, 18, 179, 255, 18, 179, 255, 18, 179, 255, 18, 179, 255, 18, 179, 255, 18, 179, 255, 18, 179, 255, 18, 179, 255, 18, 179, 255, 18, 179, 255, 18, 179, 255, 249, 248, 249, 249, 244, 249, 18, 179, 255, 18, 179, 255, 18, 179, 255, 18, 179, 255, 18, 179, 255, 18, 179, 255, 18, 179, 255, 18, 179, 255, 18, 179, 255, 18, 179, 255, 18, 179, 255, 18, 179, 255, 18, 179, 255, 18, 179, 255, 255, 255, 255, 251, 250, 250, 255, 251, 255, 18, 179, 255, 18, 179, 255, 18, 179, 255, 18, 179, 255, 18, 179, 255, 18, 179, 255, 18, 179, 255, 18, 179, 255, 18, 179, 255, 18, 179, 255, 18, 179, 255, 18, 179, 255, 18, 179, 255, 18, 179, 255, 245, 244, 244, 243, 240, 241, 18, 179, 255, 18, 179, 255, 18, 179, 255, 18, 179, 255, 18, 179, 255, 18, 179, 255, 18, 179, 255, 18, 179, 255, 18, 179, 255, 18, 179, 255, 18, 179, 255, 18, 179, 255, 18, 179, 255, 18, 179, 255, 255, 251, 255, 245, 244, 244, 243, 240, 241, 18, 179, 255, 18, 179, 255, 18, 179, 255, 18, 179, 255, 18, 179, 255, 18, 179, 255, 18, 179, 255, 18, 179, 255, 18, 179, 255, 18, 179, 255, 18, 179, 255, 18, 179, 255, 18, 179, 255, 18, 179, 255, 244, 243, 243, 247, 241, 247, 98, 204, 255, 18, 179, 255, 18, 179, 255, 18, 179, 255, 18, 179, 255, 18, 179, 255, 18, 179, 255, 18, 179, 255, 18, 179, 255, 18, 179, 255, 18, 179, 255, 18, 179, 255, 18, 179, 255, 18, 179, 255, 250, 247, 250, 240, 235, 239, 247, 241, 247, 18, 179, 255, 18, 179, 255, 18, 179, 255, 18, 179, 255, 18, 179, 255, 18, 179, 255, 18, 179, 255, 18, 179, 255, 18, 179, 255, 18, 179, 255, 18, 179, 255, 18, 179, 255, 18, 179, 255, 18, 179, 255, 251, 245, 252, 245, 238, 245, 98, 204, 255, 18, 179, 255, 18, 179, 255, 18, 179, 255, 18, 179, 255, 18, 179, 255, 18, 179, 255, 18, 179, 255, 18, 179, 255, 18, 179, 255, 18, 179, 255, 18, 179, 255, 18, 179, 255, 18, 179, 255, 246, 243, 245, 239, 237, 238, 221, 222, 220, 18, 179, 255, 18, 179, 255, 18, 179, 255, 18, 179, 255, 18, 179, 255, 18, 179, 255, 18, 179, 255, 18, 179, 255, 255, 255, 255, 255, 255, 255, 255, 255, 255, 18, 179, 255, 18, 179, 255, 18, 179, 255, 239, 236, 238, 232, 230, 230, 18, 179, 255, 18, 179, 255, 18, 179, 255, 18, 179, 255, 18, 179, 255, 18, 179, 255, 18, 179, 255, 18, 179, 255, 18, 179, 255, 98, 204, 255, 255, 255, 255, 255, 255, 255, 18, 179, 255, 18, 179, 255, 249, 241, 249, 233, 231, 231, 237, 231, 236, 18, 179, 255, 18, 179, 255, 18, 179, 255, 18, 179, 255, 18, 179, 255, 18, 179, 255, 18, 179, 255, 18, 179, 255, 18, 179, 255, 18, 179, 255, 255, 255, 255, 255, 255, 255, 237, 243, 234, 221, 231, 218, 237, 234, 236, 230, 228, 228, 98, 204, 255, 18, 179, 255, 18, 179, 255, 18, 179, 255, 18, 179, 255, 18, 179, 255, 18, 179, 255, 18, 179, 255, 18, 179, 255, 18, 179, 255, 18, 179, 255, 18, 179, 255, 98, 204, 255, 234, 232, 232, 230, 229, 229, 229, 226, 227, 98, 204, 255, 18, 179, 255, 18, 179, 255, 18, 179, 255, 18, 179, 255, 18, 179, 255, 18, 179, 255, 18, 179, 255, 18, 179, 255, 18, 179, 255, 18, 179, 255, 18, 179, 255, 18, 179, 255, 98, 204, 255, 234, 232, 232, 230, 229, 229, 229, 226, 227, 18, 179, 255, 18, 179, 255, 18, 179, 255, 18, 179, 255, 18, 179, 255, 18, 179, 255, 18, 179, 255, 18, 179, 255, 18, 179, 255, 18, 179, 255, 18, 179, 255, 18, 179, 255, 18, 179, 255, 18, 179, 255, 237, 232, 236, 234, 229, 233, 98, 204, 255, 18, 179, 255, 18, 179, 255, 18, 179, 255, 18, 179, 255, 18, 179, 255, 18, 179, 255, 18, 179, 255, 18, 179, 255, 18, 179, 255, 18, 179, 255, 18, 179, 255, 18, 179, 255, 18, 179, 255, 18, 179, 255, 18, 179, 255, 18, 179, 255, 18, 179, 255, 18, 179, 255, 18, 179, 255, 18, 179, 255, 18, 179, 255, 18, 179, 255, 18, 179, 255, 18, 179, 255, 18, 179, 255], "mask"=[], "colors"=[], "Rectangle"={"left"=0, "top"=0, "right"=17, "bottom"=17}}  # blue ok down
        w479 = T57 {"image type"=0, "image depth"=24, "image"=[18, 179, 255, 18, 179, 255, 18, 179, 255, 18, 179, 255, 18, 179, 255, 18, 179, 255, 18, 179, 255, 18, 179, 255, 18, 179, 255, 18, 179, 255, 18, 179, 255, 18, 179, 255, 18, 179, 255, 18, 179, 255, 18, 179, 255, 18, 179, 255, 18, 179, 255, 18, 179, 255, 18, 179, 255, 18, 179, 255, 18, 179, 255, 18, 179, 255, 18, 179, 255, 18, 179, 255, 18, 179, 255, 18, 179, 255, 18, 179, 255, 18, 179, 255, 18, 179, 255, 18, 179, 255, 18, 179, 255, 18, 179, 255, 18, 179, 255, 18, 179, 255, 18, 179, 255, 18, 179, 255, 255, 255, 255, 255, 255, 255, 18, 179, 255, 18, 179, 255, 18, 179, 255, 18, 179, 255, 18, 179, 255, 18, 179, 255, 18, 179, 255, 18, 179, 255, 18, 179, 255, 18, 179, 255, 18, 179, 255, 18, 179, 255, 18, 179, 255, 18, 179, 255, 18, 179, 255, 255, 255, 255, 255, 255, 255, 255, 255, 255, 18, 179, 255, 18, 179, 255, 18, 179, 255, 18, 179, 255, 18, 179, 255, 18, 179, 255, 18, 179, 255, 18, 179, 255, 18, 179, 255, 18, 179, 255, 18, 179, 255, 18, 179, 255, 18, 179, 255, 18, 179, 255, 18, 179, 255, 255, 255, 255, 255, 255, 255, 255, 255, 255, 18, 179, 255, 18, 179, 255, 18, 179, 255, 18, 179, 255, 18, 179, 255, 18, 179, 255, 18, 179, 255, 18, 179, 255, 18, 179, 255, 18, 179, 255, 18, 179, 255, 18, 179, 255, 18, 179, 255, 18, 179, 255, 18, 179, 255, 255, 255, 255, 255, 255, 255, 255, 255, 255, 18, 179, 255, 18, 179, 255, 18, 179, 255, 18, 179, 255, 18, 179, 255, 18, 179, 255, 18, 179, 255, 18, 179, 255, 18, 179, 255, 18, 179, 255, 18, 179, 255, 18, 179, 255, 18, 179, 255, 18, 179, 255, 18, 179, 255, 255, 255, 255, 255, 255, 255, 255, 255, 255, 18, 179, 255, 18, 179, 255, 18, 179, 255, 255, 255, 255, 18, 179, 255, 18, 179, 255, 18, 179, 255, 18, 179, 255, 18, 179, 255, 18, 179, 255, 18, 179, 255, 18, 179, 255, 18, 179, 255, 18, 179, 255, 18, 179, 255, 255, 255, 255, 255, 255, 255, 255, 255, 255, 18, 179, 255, 255, 255, 255, 255, 255, 255, 18, 179, 255, 18, 179, 255, 18, 179, 255, 18, 179, 255, 18, 179, 255, 18, 179, 255, 18, 179, 255, 18, 179, 255, 18, 179, 255, 18, 179, 255, 18, 179, 255, 18, 179, 255, 255, 255, 255, 255, 255, 255, 255, 255, 255, 255, 255, 255, 255, 255, 255, 255, 255, 255, 18, 179, 255, 18, 179, 255, 18, 179, 255, 18, 179, 255, 18, 179, 255, 18, 179, 255, 18, 179, 255, 18, 179, 255, 18, 179, 255, 18, 179, 255, 18, 179, 255, 18, 179, 255, 255, 255, 255, 255, 255, 255, 255, 255, 255, 255, 255, 255, 255, 255, 255, 18, 179, 255, 18, 179, 255, 18, 179, 255, 18, 179, 255, 18, 179, 255, 18, 179, 255, 18, 179, 255, 18, 179, 255, 18, 179, 255, 18, 179, 255, 18, 179, 255, 255, 255, 255, 255, 255, 255, 255, 255, 255, 255, 255, 255, 255, 255, 255, 255, 255, 255, 18, 179, 255, 18, 179, 255, 18, 179, 255, 18, 179, 255, 18, 179, 255, 18, 179, 255, 18, 179, 255, 18, 179, 255, 18, 179, 255, 18, 179, 255, 255, 255, 255, 255, 255, 255, 255, 255, 255, 255, 255, 255, 255, 255, 255, 255, 255, 255, 255, 255, 255, 255, 255, 255, 18, 179, 255, 18, 179, 255, 18, 179, 255, 18, 179, 255, 18, 179, 255, 18, 179, 255, 18, 179, 255, 18, 179, 255, 18, 179, 255, 18, 179, 255, 18, 179, 255, 255, 255, 255, 255, 255, 255, 255, 255, 255, 255, 255, 255, 255, 255, 255, 255, 255, 255, 18, 179, 255, 18, 179, 255, 18, 179, 255, 18, 179, 255, 18, 179, 255, 18, 179, 255, 18, 179, 255, 18, 179, 255, 18, 179, 255, 18, 179, 255, 18, 179, 255, 18, 179, 255, 18, 179, 255, 18, 179, 255, 255, 255, 255, 255, 255, 255, 255, 255, 255, 18, 179, 255, 18, 179, 255, 18, 179, 255, 18, 179, 255, 18, 179, 255, 18, 179, 255, 18, 179, 255, 18, 179, 255, 18, 179, 255, 18, 179, 255, 18, 179, 255, 18, 179, 255, 18, 179, 255, 18, 179, 255, 18, 179, 255, 18, 179, 255, 18, 179, 255, 18, 179, 255, 18, 179, 255, 18, 179, 255, 18, 179, 255, 18, 179, 255, 18, 179, 255, 18, 179, 255, 18, 179, 255, 18, 179, 255, 18, 179, 255, 18, 179, 255, 18, 179, 255, 18, 179, 255, 18, 179, 255, 18, 179, 255, 18, 179, 255, 18, 179, 255, 18, 179, 255, 18, 179, 255, 18, 179, 255, 18, 179, 255, 18, 179, 255, 18, 179, 255, 18, 179, 255, 18, 179, 255, 18, 179, 255, 18, 179, 255, 18, 179, 255, 18, 179, 255, 18, 179, 255, 18, 179, 255, 18, 179, 255, 18, 179, 255, 18, 179, 255, 18, 179, 255, 18, 179, 255, 18, 179, 255], "mask"=[], "colors"=[], "Rectangle"={"left"=0, "top"=0, "right"=17, "bottom"=17}}  # blue down arrow
        n162 = Build Array(w486, w485, w484, w483, w482, w481, w480, w479, w478, w477, w476, w475) -> ()  [unwired: 1 out]
      }
      frame "Init Y defs" {
        n163 = Unbundle By Name(w495) -> ("RegsParam"=w500:dbl[][], "Regs_Descriptions"=w492:string[][])
        n164 = Unbundle By Name(w494) -> ("N_regs"=w493:i32)
        n165 = call "Start Regs collect.vi"("N_regs"=w493, "error in (no error)"=w499, "Regs_Descriptions"=w492, "RegsParam"=w500, "Queue in"=w501) -> ("error out"=w498:errorcluster, "Refs"=w497:refnum<vi>[])  [unwired: 5 in]
        n166 = for {
          tunnel: w492 -> [w507] mode=indexing
          tunnel: [w503] -> w491 mode=indexing
          n167 = Index Array(array=w507, index=2) -> (element=w504:string)
          n168 = Bundle By Name(cluster=T13 {"connect"=FALSE, "gas"="N2", "Y_State"={"Y_Source"=3, "Y_SetState"=0, "SP_Set"=0.0, "SP"=0.0, "PV"=0.0, "PV_State"={"code"=0, "visible"=FALSE, "color"=0}, "Y_preSet"=0.0, "Y_Set"=0.0, "Y"=0.0, "Y_State"={"code"=0, "visible"=FALSE, "color"=0}, "YB"=FALSE}}, "gas"=w504) -> (w503:T13)
        }
        n169 = Bundle By Name(cluster=w495, "Regs_State"=w491, "RegRefs"=w497) -> (w496:T23)
      }
      frame "Init Shared Variables" {
        n170 = Unbundle By Name(w508) -> ("Regs_State"=w510:T22)
        n171 = shared-variable ".\\Var scada.lvlib\\QN_states_short"(w510, error in=w511) -> (error out=w512:errorcluster)
      }
      frame "Exit".. {
      }
      frame Default {
        n172 = Increment(x=w524) -> (x+1=w523:T2)
      }
    }
    n173 = Or(x=w21, y=w27) -> (x .or. y?=w26:bool)
  }
  n174 = Unbundle By Name(w5) -> ("Regs_Descriptions"=w4:string[][])
  n175 = for {
    tunnel: [w537] -> w8 mode=indexing
    tunnel: [w534] -> w7 mode=indexing
    tunnel: w4 -> [w533] mode=indexing
    tunnel: errorcluster {"status"=FALSE, "code"=0, "source"=""} ("error in (no error)") -> [w528]
    n176 = Index Array(array=w533, index=4 ("disabled index (col)")) -> (element=w529:string)
    n177 = Search and Replace String(replace all?=TRUE ("replace all? (F)"), input string=w529, search string=".", error in=w528) -> (result string=w527:string)  [unwired: 4 in, 3 out]
    n178 = Concatenate Strings("ns=2;s=", w527) -> (w536:string)
    n179 = Concatenate Strings(w536, ".control") -> (w534:string)
    n180 = Concatenate Strings(w536, ".state") -> (w537:string)
  }
  n181 = Unbundle By Name(w2) -> ("AI_events"=w1:refnum<event-registration>)
  n182 = while "Message Processor" {
    shift-left: w9 -> [w551]
    shift-right: [w555] -> w11
    tunnel: w12 -> [w552]
    tunnel: w2 -> [w546]
    tunnel: [w545] -> w17
    tunnel: w8 -> [w543]
    tunnel: w7 -> [w542]
    shift-right: [w540] -> _
    shift-left: w5 -> [w541]
    stop <- w554 stop-if-true
    w547 = 100  # Timeout
    n183 = call <vilib>:"Read Next Message.vi"("message queue in"=w552, "timeout (1 ms)"=w547, "error in"=w551) -> ("exit process?"=w554:bool, "message queue out"=w553:T3, "message name"=w549:string, "message value"=w548:string, "message"=w544:T58, "error out"=w550:errorcluster)  [unwired: 5 in, 2 out]
    n184 = case shown="\"Send Control\"" w549 {
      selector: w549 -> [_ _ w621 _ _ _ _ _ _ _ _ _ _ _ _ _]
      tunnel: w553 -> [_ _ _ w628 _ _ w723 _ _ w748 w771 _ w821 _ _ _]
      tunnel: w550 -> [w557 w574 w622 w626 w630 w660 w724 w726 w732 w747 w769 w795 w807 w848 w871 w924]
      tunnel: [w557 w560 w622 w624 w630 w660 w722 w726 w732 w751 w772 w797 w822 w850 w884 w924] -> w555
      tunnel: w548 -> [_ _ _ _ _ _ _ _ w731 _ _ _ _ w833 w872 _]
      tunnel: w546 -> [_ w562 _ _ _ _ _ _ _ w741 w779 w796 w805 w849 w883 _]
      tunnel: w544 -> [_ _ _ _ _ _ _ _ _ _ _ _ _ w847 _ _]
      tunnel: w543 -> [_ w573 _ _ _ _ _ _ _ _ _ _ _ _ _ _]
      tunnel: w542 -> [_ _ _ _ _ _ _ _ _ _ w777 w793 _ _ _ _]
      tunnel: w541 -> [w556 w558 w618 w623 w629 w659 w721 w725 w727 w750 w770 w790 w806 w836 w870 w923]
      tunnel: [w556 w567 w618 w623 w629 w659 w721 w725 w727 w750 w770 w790 w806 w836 w869 w923] -> w540
      frame "---------- Framework Operations ----------" {
        # "Dummy case to add a seperator in the Case Structure menu"
      }
      frame "", "Idle" {
        n185 = Unbundle By Name(w562) -> ("OPC UA.Client refnum"=w561:T17)
        n186 = call-poly <vilib>:"Multiple Read.vi"("error in (no error)"=w574, "node IDs"=w573, "OPC UA client refnum in"=w561) -> ("error out"=w571:errorcluster, "results"=w570:T60, "service status"=w572:T41)  [unwired: 5 in, 1 out]
        n187 = Unbundle By Name(w562) -> ("AI_refs"=w564:refnum<vi>[])  [unwired: 1 out]
        n188 = Unbundle By Name(w558) -> ("AI"=w565:dbl[], "AIState"=w566:T9[], "AIP"=w563:dbl[][])
        n189 = case shown="0..17" w572 {
          tunnel: w571 -> [w579 w594]
          tunnel: [w577 w593] -> w569
          tunnel: w570 -> [_ w597]
          tunnel: [w576 w595] -> w567
          tunnel: w558 -> [w578 w596]
          tunnel: [w575 w592] -> w568
          frame 18.., Default {
            n190 = in-place {
              in-place-border: [w581] -> w575
              n191 = in-place-cluster #1(w578) -> ("Regs_State"=w582:T22)
              n192 = in-place-match #2(w579) -> (w583:errorcluster)
              n193 = Array Size(array=w582) -> (size(s)=w584:i32)
              n194 = for {
                N: w584 -> [_]
                shift-right: [w585] -> w580
                shift-left: w583 -> [w585]
                shift-right: [w586] -> w581
                shift-left: w582 -> [w588]
                i -> [w587]
                n195 = in-place {
                  n196 = in-place-array #3(w588, w587) -> (w590:T13)
                  n197 = Bundle By Name(cluster=w590, "connect"=FALSE) -> (w589:T13)
                  n198 = in-place-array #3(w589) -> (w586:T22)  [unwired: 1 out]
                }
              }
              n199 = in-place-cluster #1("Regs_State"=w581) -> (w576:T23)
              n200 = in-place-match #2(w580) -> (w577:errorcluster)
            }
          }
          frame 0..17 {
            n201 = in-place {
              in-place-border: w597 -> [w602]
              in-place-border: [w598] -> w592
              n202 = in-place-cluster #4(w596) -> ("Regs_State"=w601:T22)
              n203 = in-place-match #5(w594) -> (w600:errorcluster)
              n204 = for {
                shift-right: [w604] -> w599
                shift-left: w600 -> [w605]
                shift-right: [w606] -> w598
                shift-left: w601 -> [w608]
                tunnel: w602 -> [w603] mode=indexing
                i -> [w607]
                n205 = in-place {
                  in-place-border: w603 -> [w609]
                  n206 = in-place-array #6(w608, w607) -> (w616:T13)
                  n207 = in-place-match #7(w605) -> (w611:errorcluster)
                  n208 = Unbundle By Name(w609) -> ("value"=w614:string)
                  n209 = call "From JSON Text.vim"("Data Type and Default Value"=T11 {"Y_Source"=3, "Y_SetState"=0, "SP_Set"=0.0, "SP"=0.0, "PV"=0.0, "PV_State"={"code"=0, "visible"=FALSE, "color"=0}, "Y_preSet"=0.0, "Y_Set"=0.0, "Y"=0.0, "Y_State"={"code"=0, "visible"=FALSE, "color"=0}, "YB"=FALSE} ("Y_State"), "error in (no error)"=w611, "JSON"=w614) -> ("error out"=w610:errorcluster, "Data out"=w612:T11)  [unwired: 7 in]
                  n210 = Bundle By Name(cluster=w616, "Y_State"=w612, "connect"=TRUE) -> (w615:T13)
                  n211 = in-place-array #6(w615) -> (w606:T22)  [unwired: 1 out]
                  n212 = in-place-match #7(w610) -> (w604:errorcluster)
                }
              }
              n213 = in-place-cluster #4("Regs_State"=w598) -> (w595:T23)
              n214 = in-place-match #5(w599) -> (w593:errorcluster)
            }
          }
        }
        n215 = shared-variable ".\\Var scada.lvlib\\QN_states_short"(w568, error in=w569) -> (error out=w559:errorcluster)
        n216 = call "View one AI param scada1.vi"("Sensors refs"=w564, "OPC UA.Client refnum"=w561, "error in (no error)"=w559, "AIP"=w563, "AI_State"=w566, "AITable"=w565) -> ("error out"=w560:errorcluster)  [unwired: 5 in]
      }
      frame "Missing Message Handler", Default {
        # "Call this case if a message is received that is not handled \nby any other case. Typically this is a programming error\nas a result of a typo or unhandled message/missing message handler."
        n217 = Format Into String(format string="DevError: Missing message handler for '%s\" message." ("message"), w621) -> (resulting string=w619:string)  [unwired: 2 in, 1 out]
        n218 = One Button Dialog(message=w619) -> ()  [unwired: 2 out]
      }
      frame "Error" {
        # "Proceed to Exit - Remove this if it is\nnot appropriate for the General Error case"
        # "General Error Case - this case is called if an error is passed using the error cluster below. Typically most new errors should be handed in each individual case and not passed in the rror cluster. If necessary a custom error handler case should be added and called from other cases."
        n219 = call <vilib>:"Simple Error Handler.vi"("error in (no error)"=w626) -> ()  [unwired: 1 in, 8 out]
        n220 = call <vilib>:"Clear Errors.vi"("error in (no error)"=w626) -> ("error out"=w625:errorcluster)  [unwired: 5 in, 1 out]
        n221 = call <vilib>:"Send Local Message.vi"("message queue in"=w628, "message name"="Exit", "error in"=w625) -> ("error out"=w624:errorcluster)  [unwired: 10 in, 2 out]
      }
      frame "---------- Generic Operations ----------" {
        # "Dummy case to add a seperator in the Case Structure menu"
      }
      frame "Initialize" {
        w633 = FALSE
        # "Initialize the state variables and user interface"
        n222 = Unbundle By Name(w659) -> ("RegRefs"=w637:refnum<vi>[])
        n223 = Build Array("N 1", "N 2", "N 3", "N 4", "N 5", "N 6", "N 7", "N 8", "N 9", "N 10", "N 11", "N 12", "N 13", "N 14", "N 15", "N 16", "N 17", "N 18", "N 19", "N 20") -> (w631:i32[])
        n224 = Reverse 1D Array(array=w631) -> (reversed array=w632:i32[])
        n225 = Array Size(array=w632) -> (size(s)=w635:i32)
        n226 = disable-structure shown="Disabled" {
          disable-tunnel: w631 -> [w661 _]
          frame Disabled {
            n227 = for {
              tunnel: w661 -> [w663] mode=indexing
              i -> [w662]
              n228 = case shown="19" w662 {
                tunnel: w663 -> [w664 w665 w666 w667 w668 w669 w670 w671 w672 w673 w674 w675 w676 w677 w678 w679 w680 w681 w682 w683]
                frame 0, Default {
                  n229 = property on="N 1" class="DigNum (strict)"("DefVal"=w664) -> ()  [unwired: 2 in, 2 out]
                }
                frame 1 {
                  n230 = property on="N 2" class="DigNum (strict)"("DefVal"=w665) -> ()  [unwired: 2 in, 2 out]
                }
                frame 2 {
                  n231 = property on="N 3" class="DigNum (strict)"("DefVal"=w666) -> ()  [unwired: 2 in, 2 out]
                }
                frame 3 {
                  n232 = property on="N 4" class="DigNum (strict)"("DefVal"=w667) -> ()  [unwired: 2 in, 2 out]
                }
                frame 4 {
                  n233 = property on="N 5" class="DigNum (strict)"("DefVal"=w668) -> ()  [unwired: 2 in, 2 out]
                }
                frame 5 {
                  n234 = property on="N 6" class="DigNum (strict)"("DefVal"=w669) -> ()  [unwired: 2 in, 2 out]
                }
                frame 6 {
                  n235 = property on="N 7" class="DigNum (strict)"("DefVal"=w670) -> ()  [unwired: 2 in, 2 out]
                }
                frame 7 {
                  n236 = property on="N 8" class="DigNum (strict)"("DefVal"=w671) -> ()  [unwired: 2 in, 2 out]
                }
                frame 8 {
                  n237 = property on="N 9" class="DigNum (strict)"("DefVal"=w672) -> ()  [unwired: 2 in, 2 out]
                }
                frame 9 {
                  n238 = property on="N 10" class="DigNum (strict)"("DefVal"=w673) -> ()  [unwired: 2 in, 2 out]
                }
                frame 10 {
                  n239 = property on="N 11" class="DigNum (strict)"("DefVal"=w674) -> ()  [unwired: 2 in, 2 out]
                }
                frame 11 {
                  n240 = property on="N 12" class="DigNum (strict)"("DefVal"=w675) -> ()  [unwired: 2 in, 2 out]
                }
                frame 12 {
                  n241 = property on="N 13" class="DigNum (strict)"("DefVal"=w676) -> ()  [unwired: 2 in, 2 out]
                }
                frame 13 {
                  n242 = property on="N 14" class="DigNum (strict)"("DefVal"=w677) -> ()  [unwired: 2 in, 2 out]
                }
                frame 14 {
                  n243 = property on="N 15" class="DigNum (strict)"("DefVal"=w678) -> ()  [unwired: 2 in, 2 out]
                }
                frame 15 {
                  n244 = property on="N 16" class="DigNum (strict)"("DefVal"=w679) -> ()  [unwired: 2 in, 2 out]
                }
                frame 16 {
                  n245 = property on="N 17" class="DigNum (strict)"("DefVal"=w680) -> ()  [unwired: 2 in, 2 out]
                }
                frame 17 {
                  n246 = property on="N 18" class="DigNum (strict)"("DefVal"=w681) -> ()  [unwired: 2 in, 2 out]
                }
                frame 18 {
                  n247 = property on="N 19" class="DigNum (strict)"("DefVal"=w682) -> ()  [unwired: 2 in, 2 out]
                }
                frame 19 {
                  n248 = property on="N 20" class="DigNum (strict)"("DefVal"=w683) -> ()  [unwired: 2 in, 2 out]
                }
              }
            }
          }
          frame Enabled {
          }
        }
        n249 = for {
          N: w635 -> [_]
          tunnel: w632 -> [w687]
          tunnel: [w688] -> w658 mode=indexing
          i -> [w684]
          n250 = Index Array(array=w687, index=w684) -> (element=w685:i32)
          n251 = Increment(x=w684) -> (x+1=w686:i32)
          n252 = Search 1D Array(1D array=w687, element=w685, start index (0)=w686) -> (index of element=w692:i32)
          n253 = Equal?(x=w692, y=-1) -> (x = y?=w690:bool)
          n254 = Select(t=w685, s=w690, f=0) -> (s? t:f=w688:i32)
        }
        n255 = Reverse 1D Array(array=w658) -> (reversed array=w636:i32[])
        n256 = Decrement(x=w636) -> (x-1=w634:i32[])
        n257 = for {
          tunnel: w637 -> [w696]
          tunnel: w634 -> [w693] mode=indexing
          i -> [w694]
          n258 = case shown="-1" w693 {
            selector: w693 -> [_ w698]
            tunnel: w696 -> [_ w700]
            tunnel: [refnum<vi> refnum ("VI Ref") w699] -> w695
            frame -1 {
            }
            frame 0, Default {
              n259 = Index Array(array=w700, index=w698) -> (element=w699:refnum<vi>)
            }
          }
          n260 = case shown="0, Default" w694 {
            tunnel: w695 -> [w701 w702 w703 w704 w705 w706 w707 w708 w709 w710 w711 w712 w713 w714 w715 w716 w717 w718 w719 w720]
            frame 0, Default {
              n261 = invoke on="SubP1" class="SubPnl" method="Insert VI"("VI Ref"=w701) -> ()  [unwired: 3 in, 4 out]
            }
            frame 1 {
              n262 = invoke on="SubP2" class="SubPnl" method="Insert VI"("VI Ref"=w702) -> ()  [unwired: 3 in, 4 out]
            }
            frame 2 {
              n263 = invoke on="SubP3" class="SubPnl" method="Insert VI"("VI Ref"=w703) -> ()  [unwired: 3 in, 4 out]
            }
            frame 3 {
              n264 = invoke on="SubP4" class="SubPnl" method="Insert VI"("VI Ref"=w704) -> ()  [unwired: 3 in, 4 out]
            }
            frame 4 {
              n265 = invoke on="SubP5" class="SubPnl" method="Insert VI"("VI Ref"=w705) -> ()  [unwired: 3 in, 4 out]
            }
            frame 5 {
              n266 = invoke on="SubP6" class="SubPnl" method="Insert VI"("VI Ref"=w706) -> ()  [unwired: 3 in, 4 out]
            }
            frame 6 {
              n267 = invoke on="SubP7" class="SubPnl" method="Insert VI"("VI Ref"=w707) -> ()  [unwired: 3 in, 4 out]
            }
            frame 7 {
              n268 = invoke on="SubP8" class="SubPnl" method="Insert VI"("VI Ref"=w708) -> ()  [unwired: 3 in, 4 out]
            }
            frame 8 {
              n269 = invoke on="SubP9" class="SubPnl" method="Insert VI"("VI Ref"=w709) -> ()  [unwired: 3 in, 4 out]
            }
            frame 9 {
              n270 = invoke on="SubP10" class="SubPnl" method="Insert VI"("VI Ref"=w710) -> ()  [unwired: 3 in, 4 out]
            }
            frame 10 {
              n271 = invoke on="SubP11" class="SubPnl" method="Insert VI"("VI Ref"=w711) -> ()  [unwired: 3 in, 4 out]
            }
            frame 11 {
              n272 = invoke on="SubP12" class="SubPnl" method="Insert VI"("VI Ref"=w712) -> ()  [unwired: 3 in, 4 out]
            }
            frame 12 {
              n273 = invoke on="SubP13" class="SubPnl" method="Insert VI"("VI Ref"=w713) -> ()  [unwired: 3 in, 4 out]
            }
            frame 13 {
              n274 = invoke on="SubP14" class="SubPnl" method="Insert VI"("VI Ref"=w714) -> ()  [unwired: 3 in, 4 out]
            }
            frame 14 {
              n275 = invoke on="SubP15" class="SubPnl" method="Insert VI"("VI Ref"=w715) -> ()  [unwired: 3 in, 4 out]
            }
            frame 15 {
              n276 = invoke on="SubP16" class="SubPnl" method="Insert VI"("VI Ref"=w716) -> ()  [unwired: 3 in, 4 out]
            }
            frame 16 {
              n277 = invoke on="SubP17" class="SubPnl" method="Insert VI"("VI Ref"=w717) -> ()  [unwired: 3 in, 4 out]
            }
            frame 17 {
              n278 = invoke on="SubP18" class="SubPnl" method="Insert VI"("VI Ref"=w718) -> ()  [unwired: 3 in, 4 out]
            }
            frame 18 {
              n279 = invoke on="SubP19" class="SubPnl" method="Insert VI"("VI Ref"=w719) -> ()  [unwired: 3 in, 4 out]
            }
            frame 19 {
              n280 = invoke on="SubP20" class="SubPnl" method="Insert VI"("VI Ref"=w720) -> ()  [unwired: 3 in, 4 out]
            }
          }
        }
        n281 = property on="N 1" class="DigNum (strict)"("Visible"=w633) -> ()  [unwired: 2 in, 2 out]
        n282 = property on="N 2" class="DigNum (strict)"("Visible"=w633) -> ()  [unwired: 2 in, 2 out]
        n283 = property on="N 3" class="DigNum (strict)"("Visible"=w633) -> ()  [unwired: 2 in, 2 out]
        n284 = property on="N 4" class="DigNum (strict)"("Visible"=w633) -> ()  [unwired: 2 in, 2 out]
        n285 = property on="N 5" class="DigNum (strict)"("Visible"=w633) -> ()  [unwired: 2 in, 2 out]
        n286 = property on="N 6" class="DigNum (strict)"("Visible"=w633) -> ()  [unwired: 2 in, 2 out]
        n287 = property on="N 7" class="DigNum (strict)"("Visible"=w633) -> ()  [unwired: 2 in, 2 out]
        n288 = property on="N 8" class="DigNum (strict)"("Visible"=w633) -> ()  [unwired: 2 in, 2 out]
        n289 = property on="N 9" class="DigNum (strict)"("Visible"=w633) -> ()  [unwired: 2 in, 2 out]
        n290 = property on="N 10" class="DigNum (strict)"("Visible"=w633) -> ()  [unwired: 2 in, 2 out]
        n291 = property on="N 11" class="DigNum (strict)"("Visible"=w633) -> ()  [unwired: 2 in, 2 out]
        n292 = property on="N 12" class="DigNum (strict)"("Visible"=w633) -> ()  [unwired: 2 in, 2 out]
        n293 = property on="N 13" class="DigNum (strict)"("Visible"=w633) -> ()  [unwired: 2 in, 2 out]
        n294 = property on="N 14" class="DigNum (strict)"("Visible"=w633) -> ()  [unwired: 2 in, 2 out]
        n295 = property on="N 15" class="DigNum (strict)"("Visible"=w633) -> ()  [unwired: 2 in, 2 out]
        n296 = property on="N 16" class="DigNum (strict)"("Visible"=w633) -> ()  [unwired: 2 in, 2 out]
        n297 = property on="N 17" class="DigNum (strict)"("Visible"=w633) -> ()  [unwired: 2 in, 2 out]
        n298 = property on="N 18" class="DigNum (strict)"("Visible"=w633) -> ()  [unwired: 2 in, 2 out]
        n299 = property on="N 19" class="DigNum (strict)"("Visible"=w633) -> ()  [unwired: 2 in, 2 out]
        n300 = property on="N 20" class="DigNum (strict)"("Visible"=w633) -> ()  [unwired: 2 in, 2 out]
      }
      frame "Exit" {
        # "Destroy message queue >> this will halt the UI event handler loop"
        # "Stop the VI\n>> Perform any cleanup tasks in this message case.\n>> Clear display before closing."
        n301 = call <vilib>:"Destroy Message Queue.vi"("message queue in"=w723, "error in"=w724) -> ("error out"=w722:errorcluster)  [unwired: 11 in, 2 out]
      }
      frame "---------- Application Operations ----------" {
        # "Dummy case to add a seperator in the Case Structure menu"
      }
      frame "Process Data" {
        # "Add actions to perform in response to Process button being pressed"
        n302 = Fract/Exp String To Number(string=w731) -> (number=w730:dbl)  [unwired: 4 out]
        n303 = Format Into String(format string="Process Data: %f" ("message"), w730) -> (resulting string=w728:string)  [unwired: 2 in, 1 out]
        n304 = One Button Dialog(message=w728) -> ()  [unwired: 2 out]
      }
      frame "Send auto param" {
        n305 = Unbundle By Name(w750) -> ("RegsParam"=w749:dbl[][])
        n306 = for {
          tunnel: w749 -> [w759] mode=indexing
          shift-right: [w754] -> w736
          shift-left: "UPDATE TMP_PAR SET {" ("string") -> [w755]
          i -> [w756]
          n307 = Increment(x=w756) -> (x+1=w765:i32)
          n308 = Index Array(array=w759, index=1) -> (element=w758:dbl)
          n309 = Number To Decimal String(number=w765) -> (decimal integer string=w764:string)  [unwired: 1 in]
          n310 = Number To Fractional String(use system decimal point (T)=FALSE, number=w758) -> (F-format string=w757:string)  [unwired: 2 in]
          n311 = Concatenate Strings(w755, "\"GM1QN" ("string"), w764, "_auto_value\":{\"value\":" ("string"), w757, "}," ("string")) -> (w754:string)
        }
        n312 = Unbundle By Name(w741) -> ("OPC UA.Client refnum"=w740:T17)
        n313 = String Length(string=w736) -> (length=w739:i32)
        n314 = Decrement(x=w739) -> (x-1=w737:i32)
        n315 = Replace Substring(2:1 ("length (len. of substring)"), 3:w737, 4:"}" ("string"), 5:w736) -> (1:w733:string)  [unwired: 1 out]
        n316 = Get Date/Time In Seconds() -> (seconds since 1Jan1904=w744:timestamp)
        n317 = call "Write element_1.vi"("seconds since 1Jan1904"=w744, "Variant"=w733, "node ID"=T7 "ns=2;s=CONTROL.control") -> ("request out"=w743:T19)  [unwired: 8 in]
        n318 = Build Array(w743) -> (w745:T19[])
        n319 = call-poly <vilib>:"Multiple Write.vi"("error in (no error)"=w747, "requests"=w745, "OPC UA client refnum in"=w740) -> ("error out"=w746:errorcluster)  [unwired: 5 in, 3 out]
        n320 = call <vilib>:"Send Local Message.vi"("message queue in"=w748, "message name"="Send Start On", "error in"=w746) -> ("error out"=w751:errorcluster)  [unwired: 10 in, 2 out]
        n321 = Wait (ms)(milliseconds to wait=u32 200) -> ()  [unwired: 1 out]
      }
      frame "Send Start On" {
        n322 = shared-variable ".\\Var scada.lvlib\\QN_states_short"(error in=w769) -> (w767:T61, error out=w768:errorcluster)
        n323 = Get Date/Time In Seconds() -> (seconds since 1Jan1904=w781:timestamp)
        n324 = for {
          tunnel: w781 -> [w789]
          tunnel: [w788] -> w776 mode=indexing if=w784
          tunnel: "{\"Start\":true}" -> [w787]
          tunnel: w777 -> [w786] mode=indexing
          tunnel: w767 -> [w785] mode=indexing
          w782 = u8 4  # auto
          n325 = Unbundle By Name(w785) -> ("Y_State.Y_Source"=w783:u8)
          n326 = call "Write element_1.vi"("seconds since 1Jan1904"=w789, "Variant"=w787, "node ID"=w786) -> ("request out"=w788:T19)  [unwired: 8 in]
          n327 = Equal?(x=w783, y=w782) -> (x = y?=w784:bool)
        }
        n328 = Unbundle By Name(w779) -> ("OPC UA.Client refnum"=w780:T17)
        n329 = call-poly <vilib>:"Multiple Write.vi"("error in (no error)"=w768, "requests"=w776, "OPC UA client refnum in"=w780) -> ("error out"=w773:errorcluster)  [unwired: 5 in, 3 out]
        n330 = call <vilib>:"Send Local Message.vi"("message queue in"=w771, "message name"="Send Start Off", "error in"=w773) -> ("error out"=w772:errorcluster)  [unwired: 10 in, 2 out]
        n331 = Wait (ms)(milliseconds to wait=u32 200) -> ()  [unwired: 1 out]
      }
      frame "Send Start Off" {
        n332 = Get Date/Time In Seconds() -> (seconds since 1Jan1904=w799:timestamp)
        n333 = Unbundle By Name(w796) -> ("OPC UA.Client refnum"=w798:T17)
        n334 = for {
          tunnel: w799 -> [w803]
          tunnel: [w802] -> w792 mode=indexing
          tunnel: "{\"Start\":false}" -> [w801]
          tunnel: w793 -> [w800] mode=indexing
          n335 = call "Write element_1.vi"("seconds since 1Jan1904"=w803, "Variant"=w801, "node ID"=w800) -> ("request out"=w802:T19)  [unwired: 8 in]
        }
        n336 = call-poly <vilib>:"Multiple Write.vi"("error in (no error)"=w795, "requests"=w792, "OPC UA client refnum in"=w798) -> ("error out"=w797:errorcluster)  [unwired: 5 in, 3 out]
        n337 = Wait (ms)(milliseconds to wait=u32 100) -> ()  [unwired: 1 out]
      }
      frame "Send Reset" {
        n338 = Unbundle By Name(w805) -> ("N_regs"=w804:i32)
        n339 = for {
          N: w804 -> [_]
          shift-right: [w826] -> w812
          shift-left: "UPDATE TMP_PAR SET {" ("string") -> [w827]
          i -> [w825]
          n340 = Increment(x=w825) -> (x+1=w830:i32)
          n341 = Number To Decimal String(number=w830) -> (decimal integer string=w829:string)  [unwired: 1 in]
          n342 = Concatenate Strings(w827, "\"GM1QN" ("string"), w829, "_auto_value\":{\"value\":0}," ("string")) -> (w826:string)
        }
        n343 = Unbundle By Name(w805) -> ("OPC UA.Client refnum"=w816:T17)
        n344 = String Length(string=w812) -> (length=w815:i32)
        n345 = Decrement(x=w815) -> (x-1=w813:i32)
        n346 = Replace Substring(2:1 ("length (len. of substring)"), 3:w813, 4:"}" ("string"), 5:w812) -> (1:w809:string)  [unwired: 1 out]
        n347 = Get Date/Time In Seconds() -> (seconds since 1Jan1904=w819:timestamp)
        n348 = call "Write element_1.vi"("seconds since 1Jan1904"=w819, "Variant"=w809, "node ID"=T7 "ns=2;s=CONTROL.control") -> ("request out"=w818:T19)  [unwired: 8 in]
        n349 = Build Array(w818) -> (w820:T19[])
        n350 = call-poly <vilib>:"Multiple Write.vi"("error in (no error)"=w807, "requests"=w820, "OPC UA client refnum in"=w816) -> ("error out"=w808:errorcluster)  [unwired: 5 in, 3 out]
        n351 = call <vilib>:"Send Local Message.vi"("message queue in"=w821, "message name"="Send Start On", "error in"=w808) -> ("error out"=w822:errorcluster)  [unwired: 10 in, 2 out]
        n352 = Wait (ms)(milliseconds to wait=u32 200) -> ()  [unwired: 1 out]
      }
      frame "Send Y Control" {
        n353 = Unbundle By Name(w847) -> ("attributes.keys"=w845:string[], "attributes.values"=w844:string[])
        n354 = for {
          shift-right: [w858] -> w843
          shift-left: "{" -> [w863]
          tunnel: w845 -> [w861] mode=indexing
          tunnel: w844 -> [w860] mode=indexing
          n355 = Concatenate Strings(w863, "\"", w861, "\":", w860, ",") -> (w858:string)
        }
        n356 = String Length(string=w843) -> (length=w842:i32)
        n357 = Decrement(x=w842) -> (x-1=w841:i32)
        n358 = Search and Replace String(replace all?=TRUE ("replace all? (F)"), input string=w833, search string=".") -> (result string=w832:string)  [unwired: 5 in, 3 out]
        n359 = Replace Substring(2:1 ("length (len. of substring)"), 3:w841, 4:"}", 5:w843) -> (1:w838:string)  [unwired: 1 out]
        n360 = Unbundle By Name(w849) -> ("OPC UA.Client refnum"=w852:T17)
        n361 = Concatenate Strings("ns=2;s=", w832, ".control") -> (w851:string)
        n362 = Get Date/Time In Seconds() -> (seconds since 1Jan1904=w857:timestamp)
        n363 = call "Write element_1.vi"("seconds since 1Jan1904"=w857, "Variant"=w838, "node ID"=w851) -> ("request out"=w856:T19)  [unwired: 8 in]
        n364 = Build Array(w856) -> (w855:T19[])
        n365 = call-poly <vilib>:"Multiple Write.vi"("error in (no error)"=w848, "requests"=w855, "OPC UA client refnum in"=w852) -> ("error out"=w850:errorcluster)  [unwired: 5 in, 3 out]
        n366 = Wait (ms)(milliseconds to wait=u32 200) -> ()  [unwired: 1 out]
      }
      frame "Send Control" {
        (unwired) "UPDATE AO SET {\"GM1QN1_YQ01\":{\"instrument_gain\":1.000000}}" ("Display")
        # "instrument_gain = output_k in PAR table\nbut output_k not updated becos not need yet"
        n367 = Unbundle By Name(w870) -> ("RegsParam"=w867:dbl[][], "Regs_Descriptions"=w866:string[][])
        n368 = Scan From String(format string="%s%s SET %[^]", input string=w872, error in=w871) -> (error out=w873:errorcluster, output 1=w879:string, output 2=w878:string, output 3=w877:string)  [unwired: 4 in, 2 out]
        n369 = call "Is Value Changed.vim"("value"=w872) -> ("changed or first call?"=w875:bool)
        n370 = Not(x=w873) -> (.not. x?=w876:bool)
        n371 = And(x=w876, y=w875) -> (x .and. y?=w874:bool)
        n372 = case shown="True" w874 {
          tunnel: w879 -> [_ w899]
          tunnel: [w891 w896] -> w868
          tunnel: w878 -> [_ w898]
          tunnel: w877 -> [_ w897]
          tunnel: w873 -> [w890 w895]
          tunnel: w867 -> [w889 w894]
          tunnel: w866 -> [_ w893]
          tunnel: [w889 w892] -> w865
          frame False {
            n373 = call <vilib>:"Clear Errors.vi"("error in (no error)"=w890) -> ("error out"=w891:errorcluster)  [unwired: 5 in, 1 out]
          }
          frame True {
            n374 = case shown="\"UPDATE\"" w899 {
              tunnel: w898 -> [_ w907]
              tunnel: w897 -> [_ w906]
              tunnel: w895 -> [w901 w908]
              tunnel: [w901 w905] -> w896
              tunnel: w894 -> [w900 w904]
              tunnel: w893 -> [_ w903]
              tunnel: [w900 w902] -> w892
              frame Default {
              }
              frame "UPDATE" {
                n375 = case shown="\"PAR\", \"TMP_PAR\"" w907 {
                  tunnel: w906 -> [_ w916]
                  tunnel: [w910 w911] -> w905
                  tunnel: w908 -> [w910 w915]
                  tunnel: w904 -> [w909 w914]
                  tunnel: w903 -> [_ w913]
                  tunnel: [w909 w912] -> w902
                  frame Default {
                  }
                  frame "PAR", "TMP_PAR" {
                    n376 = call "Write json to reg param one.vi"("error in (no error)"=w915, "RegsDescriptions"=w913, "JSON Data In"=w916, "RegsParam in"=w914) -> ("error out"=w911:errorcluster, "RegsParam out"=w912:dbl[][])  [unwired: 6 in]
                  }
                }
              }
            }
          }
        }
        n377 = Bundle By Name(cluster=w870, "RegsParam"=w865) -> (w869:T23)
        n378 = Unbundle By Name(w883) -> ("OPC UA.Client refnum"=w885:T17)
        n379 = Get Date/Time In Seconds() -> (seconds since 1Jan1904=w888:timestamp)
        n380 = call "Write element_1.vi"("seconds since 1Jan1904"=w888, "Variant"=w872, "node ID"=T7 "ns=2;s=CONTROL.control") -> ("request out"=w887:T19)  [unwired: 8 in]
        n381 = Build Array(w887) -> (w886:T19[])
        n382 = call-poly <vilib>:"Multiple Write.vi"("error in (no error)"=w868, "requests"=w886, "OPC UA client refnum in"=w885) -> ("error out"=w884:errorcluster)  [unwired: 5 in, 3 out]
        n383 = Wait (ms)(milliseconds to wait=u32 200) -> ()  [unwired: 1 out]
      }
      frame "Replase Panel" {
        n384 = Unbundle By Name(w923) -> ("RegRefs"=w922:refnum<vi>[])
        n385 = disable-structure shown="Disabled" {
          frame Disabled {
            n386 = property on="SubP10" class="SubPnl"() -> ("InsertedVI"=w925:refnum<vi>)  [unwired: 2 in, 2 out]
            n387 = invoke class="VI" method="Ctrl Val.Get"(reference=w925, "Control Name"="object_full_name") -> (error out=w927:errorcluster, "Get Control Value Variant"=w928:variant)  [unwired: 2 in, 2 out]
            n388 = Variant To Data(error in=w927, type="" ("Control Name"), Variant=w928) -> (data=→"Control Name":string)  [unwired: 1 out]
          }
          frame Enabled {
          }
        }
        n389 = invoke on="SubP11" class="SubPnl" method="Remove VI"() -> (error out=w918:errorcluster)  [unwired: 3 in, 2 out]
        n390 = Index Array(array=w922, index=10) -> (element=w917:refnum<vi>)
        n391 = invoke on="SubP10" class="SubPnl" method="Remove VI"(error in=w918) -> (error out=w921:errorcluster)  [unwired: 2 in, 2 out]
        n392 = invoke on="SubP10" class="SubPnl" method="Insert VI"(error in=w921, "VI Ref"=w917) -> (error out=w919:errorcluster)  [unwired: 2 in, 3 out]
        n393 = case shown="Error .." w919 {
          selector: w919 -> [_ w931]
          frame No Error {
          }
          frame Error {
            n394 = call <vilib>:"Simple Error Handler.vi"("error in (no error)"=w931) -> ()  [unwired: 4 in, 5 out]
          }
        }
      }
    }
    n395 = control-ref of="This VI"() -> (w545:refnum<vi>)
  }
  n396 = while "Message Generator - User Interface Event Handler" {
    tunnel: w12 -> [w936]
    tunnel: w1 -> [w935]
    tunnel: [w934] -> w16
    tunnel: [w933] -> w10
    tunnel: errorcluster {"status"=FALSE, "code"=0, "source"=""} ("error out") -> [w932]
    stop <- w937 stop-if-true
    w938 = 100  # Event Structure Timeout (ms)
    n397 = event shown="[0] Timeout" {
      selector: w935 -> [_ _ _ _ _ _ _ _]
      dyn-events: [_ _ _ _ _ _ _ _] -> w934
      timeout: w938 -> [_ _ _ _ _ _ _ _]
      tunnel: [w939 w966 w981 _ _ _ _ _] -> w937
      tunnel: w936 -> [w941 w968 w980 w994 w1007 w1011 w1015 w1019]
      tunnel: [w940 _ w982 w992 w996 w1008 w1012 w1016] -> w933
      tunnel: w932 -> [w942 w967 w983 w993 w997 w1009 w1013 w1017]
      event Timeout {
        # "Exit UI event handler loop if message queue\nis destroyed in the message processor"
        n398 = event-data() -> ()  [unwired: 2 out]
        n399 = case shown="No Error" w942 {
          selector: w942 -> [w947 w955]
          tunnel: w941 -> [w948 w957]
          tunnel: [w944 w958] -> w940
          tunnel: [w943 w952] -> w939
          frame No Error {
            n400 = call <vilib>:"Check Message Queue Status.vi"("message queue in"=w948, "error in"=w947) -> ("message queue out"=w945:T3, "error out"=w946:errorcluster)  [unwired: 9 in, 3 out]
            n401 = case shown="No Error" w946 {
              selector: w946 -> [w949 w951]
              tunnel: [w949 w951] -> w944
              tunnel: w945 -> [_ _]
              tunnel: [_ TRUE] -> w943
              frame No Error {
              }
              frame Error {
              }
            }
          }
          frame Error {
            n402 = call <vilib>:"Clear Errors.vi"("error in (no error)"=w955) -> ("error out"=w956:errorcluster)  [unwired: 5 in, 1 out]
            n403 = call <vilib>:"Check Message Queue Status.vi"("message queue in"=w957, "error in"=w956) -> ("message queue out"=w953:T3, "error out"=w954:errorcluster)  [unwired: 9 in, 3 out]
            n404 = case shown="No Error" w954 {
              selector: w954 -> [w961 w965]
              tunnel: [w962 w965] -> w958
              tunnel: w953 -> [w960 _]
              tunnel: [TRUE TRUE] -> w952
              frame No Error {
                n405 = call <vilib>:"Send Local Message.vi"("message queue in"=w960, "message name"="Exit", "error in"=w961) -> ("error out"=w962:errorcluster)  [unwired: 10 in, 2 out]
              }
              frame Error {
              }
            }
          }
        }
        n406 = local write "Останов\nпрограммы"(w939) -> ()
      }
      event Panel Close? {
        n407 = event-data() -> ()  [unwired: 2 out]
        n408 = Two Button Dialog(message="Остановить программу?\nНагрев останется") -> (T button?=w970:bool)  [unwired: 2 in]
        n409 = case shown="True" w970 {
          selector: w970 -> [w973 w974]
          tunnel: w968 -> [_ w977]
          tunnel: [w972 w976] -> _
          tunnel: w967 -> [w972 w975]
          tunnel: [w973 w974] -> w971
          frame False {
          }
          frame True {
            n410 = local write "Останов\nпрограммы"(w974) -> ()
            n411 = call <vilib>:"Send Local Message.vi"("message queue in"=w977, "message name"="Exit", "error in"=w975) -> ("error out"=w976:errorcluster)  [unwired: 10 in, 2 out]
          }
        }
        n412 = Not(x=w971) -> (.not. x?=w966:bool)
        n413 = event-data("Discard?"=w966) -> ()  [unwired: 1 in, 1 out]
      }
      event "Останов\nпрограммы": Value Change {
        # "Exit the application\n>> Stop this message generator loop"
        n414 = event-data() -> ()  [unwired: 5 out]
        n415 = Two Button Dialog(message="Остановить программу?\nРасходы останутся") -> (T button?=w979:bool)  [unwired: 2 in]
        n416 = case shown="True" w979 {
          selector: w979 -> [w986 w987]
          tunnel: w980 -> [_ w990]
          tunnel: [w985 w989] -> w982
          tunnel: w983 -> [w985 w988]
          tunnel: [w986 w987] -> w981
          frame False {
          }
          frame True {
            n417 = local write "Останов\nпрограммы"(w987) -> ()
            n418 = call <vilib>:"Send Local Message.vi"("message queue in"=w990, "message name"="Exit", "error in"=w988) -> ("error out"=w989:errorcluster)  [unwired: 10 in, 2 out]
          }
        }
      }
      event Menu Selection (User) {
        # "Add run-time menu items to the message\nqueue. The message handler case names must match the menu ItemTag names."
        n419 = event-data() -> ("ItemTag"=w995:string)  [unwired: 1 out]
        n420 = call <vilib>:"Send Local Message.vi"("message queue in"=w994, "message name"=w995, "error in"=w993) -> ("error out"=w992:errorcluster)  [unwired: 10 in, 2 out]
      }
      event "process": Value Change {
        n421 = event-data() -> ()  [unwired: 2 out]
        n422 = Random Number (0-1)() -> (number: 0 to 1=w1004:dbl)
        n423 = Number To Fractional String(number=w1004) -> (F-format string=w1005:string)  [unwired: 3 out]
        n424 = call <vilib>:"Send Local Message.vi"("message queue in"=w1007, "message name"="Process Data", "message value"=w1005, "error in"=w997) -> ("message queue out"=w1003:T3, "error out"=w999:errorcluster)  [unwired: 9 in, 1 out]
        n425 = call <vilib>:"Send Network Message.vi"("message queue in"=w1003, "receiver process"="Control", "receiver host"="192.168.0.70", "receiver port (0)"=u16 9000, "message name"="message name", "error in"=w999) -> ("error out"=w996:errorcluster)  [unwired: 7 in, 2 out]
      }
      event "Start": Value Change {
        n426 = event-data() -> ()  [unwired: 7 out]
        n427 = call <vilib>:"Send Local Message.vi"("message queue in"=w1011, "message name"="Send auto param", "error in"=w1009) -> ("error out"=w1008:errorcluster)  [unwired: 10 in, 2 out]
      }
      event "Reset": Value Change {
        n428 = event-data() -> ()  [unwired: 7 out]
        n429 = call <vilib>:"Send Local Message.vi"("message queue in"=w1015, "message name"="Send Reset", "error in"=w1013) -> ("error out"=w1012:errorcluster)  [unwired: 10 in, 2 out]
      }
      event "HT1 emergency stop": Value Change {
        n430 = event-data() -> ()  [unwired: 7 out]
        n431 = call <vilib>:"Send Local Message.vi"("message queue in"=w1019, "message name"="Send Reset", "error in"=w1017) -> ("error out"=w1016:errorcluster)  [unwired: 10 in, 2 out]
      }
    }
  }
  n432 = disable-structure shown="Disabled" {
    disable-tunnel: w9 -> [w1022 _]
    disable-tunnel: w5 -> [w1021 _]
    disable-tunnel: w2 -> [w1020 _]
    frame Disabled {
      n433 = while {
        shift-right: [w1032] -> _
        shift-left: scada_prog_state."ReadAIParam" ("Enum") -> [w1033]
        tunnel: w1020 -> [w1026]
        shift-right: [w1028] -> _
        shift-left: w1021 -> [w1027]
        shift-right: [w1031] -> _
        shift-left: w1022 -> [w1030]
        tunnel: [w1024] -> _
        stop <- w1029 stop-if-true
        n434 = case shown="\"ReadDIParam\"" w1033 {
          tunnel: [scada_prog_state."ReadDIParam" ("Enum") scada_prog_state."AI" ("Enum") scada_prog_state."AIValues" ("Enum") scada_prog_state."Alarms" ("Enum") scada_prog_state."TB1" ("Enum") scada_prog_state."TB2" ("Enum") scada_prog_state."TB3" ("Enum") scada_prog_state."Exit" ("Enum") scada_prog_state."AI" ("Enum")] -> w1032
          tunnel: [w1035 w1073 w1112 w1241 w1317 w1419 w1492 w1566 w1625] -> w1031
          tunnel: w1030 -> [w1034 w1074 w1111 w1240 w1314 w1424 w1498 w1572 w1625]
          tunnel: [_ _ _ _ _ _ _ _ w1624] -> w1029
          tunnel: [w1038 w1071 w1110 w1243 w1316 w1402 w1495 w1569 w1623] -> w1028
          tunnel: w1027 -> [w1037 w1072 w1109 w1243 w1316 w1421 w1494 w1571 w1623]
          tunnel: w1026 -> [w1036 w1075 w1108 w1242 w1313 w1425 w1499 w1573 w1621]
          tunnel: [_ _ _ _ _ _ _ _ "tick"] -> w1025
          tunnel: [w1036 w1075 w1108 w1242 w1313 w1425 w1499 w1573 w1621] -> w1024
          frame "ReadAIParam", Default {
            n435 = disable-structure shown="SERVER==OPC" {
              disable-tunnel: [w1044 w1054] -> w1039
              disable-tunnel: w1036 -> [w1047 w1062]
              disable-tunnel: w1034 -> [w1045 w1057]
              disable-tunnel: [w1041 w1056] -> w1035
              frame condition #0 {
                n436 = Unbundle By Name(w1047) -> ("Enums.AI"=w1043:string[], "AI_Names_SHVR"=w1046)
                n437 = shared-variable-read(w1046, w1045) -> (w1041:errorcluster, w1042:string[])  [unwired: 2 out]
                n438 = case shown="No Error" w1041 {
                  tunnel: w1042 -> [_ w1048]
                  tunnel: w1043 -> [_ w1050]
                  tunnel: [_ w1049] -> w1044
                  frame Error {
                  }
                  frame No Error {
                    n439 = for {
                      tunnel: w1050 -> [w1053] mode=indexing
                      tunnel: w1048 -> [w1052]
                      tunnel: [w1051] -> w1049 mode=indexing
                      n440 = Search 1D Array(1D array=w1052, element=w1053) -> (index of element=w1051:i32)  [unwired: 1 in]
                    }
                  }
                }
              }
              frame condition #1 (active) {
                n441 = Unbundle By Name(w1062) -> ("Enums.AI"=w1055:string[], "OPC UA.Client refnum"=w1059:T17)
                n442 = call-poly <vilib>:"Multiple Read.vi"("error in (no error)"=w1057, "node IDs"=T6 ["ns=2;s=AI.AI_Names"] ("OPC UA.node IDs"), "OPC UA client refnum in"=w1059) -> ("error out"=w1056:errorcluster, "results"=w1061:T42, "service status"=w1060:T41)  [unwired: 5 in, 1 out]
                n443 = case shown="0..15" w1060 {
                  tunnel: w1061 -> [_ w1066]
                  tunnel: w1055 -> [_ w1064]
                  tunnel: [_ w1063] -> w1054
                  frame 16.., Default {
                  }
                  frame 0..15 {
                    n444 = Index Array(array=w1066) -> (element=w1067:T43)  [unwired: 1 in]
                    n445 = Unbundle By Name(w1067) -> ("values"=w1065:string[])
                    n446 = for {
                      tunnel: w1064 -> [w1070] mode=indexing
                      tunnel: w1065 -> [w1069]
                      tunnel: [w1068] -> w1063 mode=indexing
                      n447 = Search 1D Array(1D array=w1069, element=w1070) -> (index of element=w1068:i32)  [unwired: 1 in]
                    }
                  }
                }
              }
            }
            n448 = Bundle By Name(cluster=w1037, "AI_reorder_table"=w1039) -> (w1038:T23)
          }
          frame "ReadDIParam" {
            n449 = disable-structure shown="SERVER==OPC" {
              disable-tunnel: [w1081 w1091] -> w1076
              disable-tunnel: w1075 -> [w1084 w1099]
              disable-tunnel: w1074 -> [w1082 w1094]
              disable-tunnel: [w1078 w1093] -> w1073
              frame condition #0 {
                n450 = Unbundle By Name(w1084) -> ("Enums.DI"=w1080:string[], "DI_Names_SHVR"=w1083)
                n451 = shared-variable-read(w1083, w1082) -> (w1078:errorcluster, w1079:string[])  [unwired: 2 out]
                n452 = case shown="No Error" w1078 {
                  tunnel: w1079 -> [_ w1085]
                  tunnel: w1080 -> [_ w1087]
                  tunnel: [_ w1086] -> w1081
                  frame Error {
                  }
                  frame No Error {
                    n453 = for {
                      tunnel: w1087 -> [w1090] mode=indexing
                      tunnel: w1085 -> [w1089]
                      tunnel: [w1088] -> w1086 mode=indexing
                      n454 = Search 1D Array(1D array=w1089, element=w1090) -> (index of element=w1088:i32)  [unwired: 1 in]
                    }
                  }
                }
              }
              frame condition #1 (active) {
                n455 = Unbundle By Name(w1099) -> ("Enums.DI"=w1092:string[], "OPC UA.Client refnum"=w1096:T17)
                n456 = call-poly <vilib>:"Multiple Read.vi"("error in (no error)"=w1094, "node IDs"=T6 ["ns=2;s=DI.DI_Names"] ("OPC UA.node IDs"), "OPC UA client refnum in"=w1096) -> ("error out"=w1093:errorcluster, "results"=w1098:T42, "service status"=w1097:T41)  [unwired: 5 in, 1 out]
                n457 = case shown="0..15" w1097 {
                  tunnel: w1098 -> [_ w1103]
                  tunnel: w1092 -> [_ w1101]
                  tunnel: [_ w1100] -> w1091
                  frame 16.., Default {
                  }
                  frame 0..15 {
                    n458 = Index Array(array=w1103) -> (element=w1104:T43)  [unwired: 1 in]
                    n459 = Unbundle By Name(w1104) -> ("values"=w1102:string[])
                    n460 = for {
                      tunnel: w1101 -> [w1107] mode=indexing
                      tunnel: w1102 -> [w1106]
                      tunnel: [w1105] -> w1100 mode=indexing
                      n461 = Search 1D Array(1D array=w1106, element=w1107) -> (index of element=w1105:i32)  [unwired: 1 in]
                    }
                  }
                }
              }
            }
            n462 = Bundle By Name(cluster=w1072, "DI_reorder_table"=w1076) -> (w1071:T23)
          }
          frame "AI" {
            # "ReadParam"
            n463 = in-place {
              in-place-border: w1108 -> [w1120]
              in-place-border: [w1119] -> w1112
              in-place-border: w1111 -> [w1118]
              in-place-border: w1109 -> [w1117]
              n464 = in-place-cluster #8(w1109) -> ()  [unwired: 3 out]
              n465 = disable-structure shown="SERVER==OPC" {
                disable-tunnel: w1117 -> [w1126 w1193]
                disable-tunnel: w1120 -> [w1137 w1192]
                disable-tunnel: [w1124 w1185] -> w1119
                disable-tunnel: w1118 -> [w1136 w1190]
                disable-tunnel: [w1123 w1184] -> w1116
                disable-tunnel: [w1122 w1183] -> w1115
                disable-tunnel: [w1121 w1182] -> w1114
                frame condition #0 (active) {
                  n466 = Unbundle By Name(w1137) -> ("OPC UA.Client refnum"=w1139:T17)
                  n467 = Unbundle By Name(w1126) -> ("AI_reorder_table"=w1125:i32[])
                  n468 = call-poly <vilib>:"Multiple Read.vi"("error in (no error)"=w1136, "node IDs"=T6 ["ns=2;s=AI.AI"] ("OPC UA.node IDs"), "OPC UA client refnum in"=w1139) -> ("error out"=w1134:errorcluster, "results"=w1140:T67, "OPC UA client refnum out"=w1135:T17, "service status"=w1132:T41)  [unwired: 5 in]
                  n469 = call-poly <vilib>:"Multiple Read.vi"("error in (no error)"=w1134, "node IDs"=T6 ["ns=2;s=AI.AI_State", "ns=2;s=AI.AI_ALRState"] ("OPC UA.node IDs"), "OPC UA client refnum in"=w1135) -> ("error out"=w1124:errorcluster, "results"=w1127:T68, "service status"=w1131:T41)  [unwired: 5 in, 1 out]
                  n470 = case shown="0..15" w1131 {
                    tunnel: [_ TRUE] -> w1130
                    frame 16.., Default {
                    }
                    frame 0..15 {
                    }
                  }
                  n471 = case shown="0..15" w1132 {
                    tunnel: [_ TRUE] -> w1129
                    frame 16.., Default {
                    }
                    frame 0..15 {
                    }
                  }
                  n472 = And(x=w1130, y=w1129) -> (x .and. y?=w1128:bool)
                  n473 = case shown="True" w1128 {
                    tunnel: w1140 -> [w1153 _]
                    tunnel: w1127 -> [w1152 _]
                    tunnel: w1125 -> [w1147 w1177]
                    tunnel: [w1145 w1176] -> w1123
                    tunnel: [w1144 w1175] -> w1122
                    tunnel: [w1143 w1174] -> w1121
                    frame True {
                      n474 = Index Array(array=w1153) -> (element=w1154:T69)  [unwired: 1 in]
                      n475 = Index Array(array=w1152) -> (element #1=w1151:T70, element #2=w1149:T70)  [unwired: 2 in]
                      n476 = Unbundle By Name(w1154) -> ("values"=w1150:dbl[])
                      n477 = Unbundle By Name(w1151) -> ("values"=w1148:i32[])
                      n478 = Unbundle By Name(w1149) -> ("values"=w1146:i32[])
                      n479 = for {
                        tunnel: w1150 -> [w1161]
                        tunnel: w1147 -> [w1157] mode=indexing
                        tunnel: [w1160] -> w1145 mode=indexing
                        tunnel: w1146 -> [w1159]
                        tunnel: [w1158] -> w1144 mode=indexing
                        tunnel: w1148 -> [w1156]
                        tunnel: [w1155] -> w1143 mode=indexing
                        n480 = case shown="0, Default" w1157 {
                          selector: w1157 -> [_ w1165]
                          tunnel: w1161 -> [_ w1173]
                          tunnel: [nan ("PV") w1172] -> w1160
                          tunnel: w1159 -> [_ w1171]
                          tunnel: [T9 {"code"=0, "visible"=FALSE, "color"=14803425, "source"="отсутствует запись или ошибка в базе данных "} ("STATE") w1167] -> w1158
                          tunnel: w1156 -> [_ w1170]
                          tunnel: [errorcluster {"status"=TRUE, "code"=10, "source"="отсутствует запись или ошибка в базе данных "} ("ALRSTATE") w1166] -> w1155
                          frame -1 {
                          }
                          frame 0, Default {
                            n481 = Index Array(array=w1173, index=w1165) -> (element=w1172:dbl)
                            n482 = Index Array(array=w1170, index=w1165) -> (element=w1169:i32)
                            n483 = Index Array(array=w1171, index=w1165) -> (element=w1168:i32)
                            n484 = call "Sensor handling scada.vi"("AI_ALRState"=w1168, "AI_State"=w1169) -> ("ALRSTATE"=w1166:errorcluster, "STATE"=w1167:T9)  [unwired: 8 in]
                          }
                        }
                      }
                    }
                    frame False {
                      n485 = Array Size(array=w1177) -> (size(s)=w1178:i32)
                      n486 = for {
                        N: w1178 -> [_]
                        tunnel: [nan ("PV")] -> w1176 mode=indexing
                        tunnel: [T9 {"code"=0, "visible"=FALSE, "color"=14803425, "source"="отсутствует запись или ошибка в базе данных "} ("STATE")] -> w1175 mode=indexing
                        tunnel: [errorcluster {"status"=TRUE, "code"=10, "source"="отсутствует запись или ошибка в базе данных "} ("ALRSTATE")] -> w1174 mode=indexing
                      }
                    }
                  }
                }
                frame condition #1 {
                  n487 = Unbundle By Name(w1192) -> ("AI_SHVR"=w1194)
                  n488 = Unbundle By Name(w1193) -> ("AI_reorder_table"=w1188:i32[])
                  n489 = Unbundle By Name(w1192) -> ("CPU_utilization"=w1191:refnum<k21>)
                  n490 = shared-variable-read(w1191) -> (→"CPU %":dbl)  [unwired: 1 in, 3 out]
                  n491 = shared-variable-read(w1194, w1190) -> (w1185:errorcluster, w1195:T71)  [unwired: 2 out]
                  n492 = Unbundle By Name(w1195) -> ("AI"=w1189:dbl[], "AIState"=w1187:T9[], "AIALRState"=w1186:errorcluster[])
                  n493 = case shown="No Error" w1185 {
                    tunnel: w1189 -> [w1203 _]
                    tunnel: w1188 -> [w1202 w1224]
                    tunnel: w1187 -> [w1201 _]
                    tunnel: w1186 -> [w1200 _]
                    tunnel: [w1199 w1223] -> w1184
                    tunnel: [w1198 w1222] -> w1183
                    tunnel: [w1197 w1221] -> w1182
                    frame No Error {
                      n494 = for {
                        tunnel: w1203 -> [w1210]
                        tunnel: w1202 -> [w1206] mode=indexing
                        tunnel: [w1209] -> w1199 mode=indexing
                        tunnel: w1200 -> [w1208]
                        tunnel: [w1207] -> w1198 mode=indexing
                        tunnel: w1201 -> [w1205]
                        tunnel: [w1204] -> w1197 mode=indexing
                        n495 = case shown="0, Default" w1206 {
                          selector: w1206 -> [_ w1214]
                          tunnel: w1210 -> [_ w1220]
                          tunnel: [nan ("PV") w1219] -> w1209
                          tunnel: w1208 -> [_ w1218]
                          tunnel: [T9 {"code"=0, "visible"=FALSE, "color"=14803425, "source"="отсутствует запись или ошибка в базе данных "} ("STATE") w1216] -> w1207
                          tunnel: w1205 -> [_ w1217]
                          tunnel: [errorcluster {"status"=TRUE, "code"=10, "source"="отсутствует запись или ошибка в базе данных "} ("ALRSTATE") w1215] -> w1204
                          frame -1 {
                          }
                          frame 0, Default {
                            n496 = Index Array(array=w1220, index=w1214) -> (element=w1219:dbl)
                            n497 = Index Array(array=w1217, index=w1214) -> (element=w1216:T9)
                            n498 = Index Array(array=w1218, index=w1214) -> (element=w1215:errorcluster)
                          }
                        }
                      }
                    }
                    frame Error {
                      n499 = Array Size(array=w1224) -> (size(s)=w1225:i32)
                      n500 = for {
                        N: w1225 -> [_]
                        tunnel: [nan ("PV")] -> w1223 mode=indexing
                        tunnel: [T9 {"code"=0, "visible"=FALSE, "color"=14803425, "source"="отсутствует запись или ошибка в базе данных "} ("STATE")] -> w1222 mode=indexing
                        tunnel: [errorcluster {"status"=TRUE, "code"=10, "source"="отсутствует запись или ошибка в базе данных "} ("ALRSTATE")] -> w1221 mode=indexing
                      }
                    }
                  }
                }
              }
              n501 = in-place-cluster #8("AI"=w1116, "AIState"=w1115, "AIALRState"=w1114) -> (w1110:T23)
            }
          }
          frame "AIValues" {
            n502 = Unbundle By Name(w1242) -> ("AI_refs"=w1239:refnum<vi>[])
            n503 = Unbundle By Name(w1243) -> ("AI"=w1232:dbl[], "AIState"=w1231:T9[])
            n504 = for {
              tunnel: w1239 -> [w1270] mode=indexing
              tunnel: w1231 -> [w1274] mode=indexing
              shift-right: [w1272] -> w1241
              shift-left: w1240 -> [w1273]
              tunnel: w1232 -> [w1271] mode=indexing
              n505 = Not A Number/Path/Refnum?(number/path/refnum=w1270) -> (NaN/Path/Refnum?=w1269:bool)
              n506 = case shown="False" w1269 {
                tunnel: w1274 -> [w1284 _]
                tunnel: w1273 -> [w1283 w1309]
                tunnel: [w1282 w1309] -> w1272
                tunnel: w1271 -> [w1281 _]
                tunnel: w1270 -> [w1279 _]
                frame False {
                  n507 = Unbundle By Name(w1284) -> ("code"=w1280:i32, "visible"=w1275:bool, "color"=w1277:u32)
                  n508 = case shown="1, Default" w1280 {
                    tunnel: [w1285 u32 16777216 ("Color Box") u32 16718848 ("Color Box") u32 16449346 ("Color Box") u32 16449346 ("Color Box") u32 16718848 ("Color Box") u32 0 ("Color Box") w1305 w1307] -> _
                    tunnel: [FALSE FALSE FALSE FALSE FALSE FALSE TRUE FALSE FALSE] -> w1276
                    tunnel: [w1285 u32 3997440 ("Color Box") u32 16449346 ("Color Box") u32 16718848 ("Color Box") u32 16718848 ("Color Box") u32 16449346 ("Color Box") u32 16772394 ("Color Box") w1305 w1307] -> _
                    frame 0 {
                      w1285 = u32 13816530 ("Color Box")
                    }
                    frame 1, Default {
                    }
                    frame 2 {
                    }
                    frame 3 {
                    }
                    frame 4 {
                    }
                    frame 5 {
                    }
                    frame 6 {
                    }
                    frame 7 {
                      w1305 = u32 13816530 ("Color Box")
                    }
                    frame 8 {
                      w1307 = u32 13816530 ("Color Box")
                    }
                  }
                  n509 = property on="Property Node" class="DigNum (strict)"(reference=w1279, error in=w1283, "Value"=w1281, "NumText.TextColor"=u32 3997440 ("Color Box"), "NumText.BGColor"=w1277, "NumText.Visible"=w1275, "Blinking"=w1276) -> (error out=w1282:errorcluster)  [unwired: 1 out]
                }
                frame True {
                }
              }
            }
            n510 = Index Array(array=w1232, index="AI_enum") -> (element=w1237:dbl)
            "EB3BP1_XQ01" <- w1237
            n511 = Index Array(array=w1231, index="AI_enum") -> (element=w1235:T9)
            n512 = Unbundle By Name(w1235) -> ("code"=w1236:i32, "source"=w1233:string, "color"=w1229:u32)
            n513 = case shown="1, Default" w1236 {
              tunnel: [w1245 u32 16777216 ("Color Box") u32 16718848 ("Color Box") u32 16449346 ("Color Box") u32 16449346 ("Color Box") u32 16718848 ("Color Box") u32 0 ("Color Box") w1265 w1267] -> _
              tunnel: [FALSE FALSE FALSE FALSE FALSE FALSE TRUE FALSE FALSE] -> w1234
              tunnel: [w1245 u32 3997440 ("Color Box") u32 16449346 ("Color Box") u32 16718848 ("Color Box") u32 16718848 ("Color Box") u32 16449346 ("Color Box") u32 16772394 ("Color Box") w1265 w1267] -> _
              frame 0 {
                w1245 = u32 13816530 ("Color Box")
              }
              frame 1, Default {
              }
              frame 2 {
              }
              frame 3 {
              }
              frame 4 {
              }
              frame 5 {
              }
              frame 6 {
              }
              frame 7 {
                w1265 = u32 13816530 ("Color Box")
              }
              frame 8 {
                w1267 = u32 13816530 ("Color Box")
              }
            }
            n514 = property on="EB3BP1_XQ01" class="DigNum (strict)"("Value"=w1237, "NumText.TextColor"=u32 3997440 ("Color Box"), "Blinking"=w1234, "TipStrip"=w1233, "NumText.BGColor"=w1229) -> ()  [unwired: 2 in, 2 out]
          }
          frame "Alarms" {
            n515 = in-place {
              in-place-border: w1313 -> [w1325]
              n516 = in-place-cluster #9(w1316) -> ("ALR_State"=w1324:T10, "ALR_Names"=w1319:string[])
              n517 = in-place-match #10(w1314) -> (w1321:errorcluster)
              n518 = disable-structure shown="SERVER==OPC" {
                disable-tunnel: w1325 -> [w1330 w1393]
                disable-tunnel: [w1332 w1391] -> _
                disable-tunnel: w1321 -> [w1351 w1384]
                disable-tunnel: [w1333 w1392] -> w1320
                disable-tunnel: [w1334 w1386] -> w1322
                disable-tunnel: [w1342 w1389] -> w1323
                disable-tunnel: w1324 -> [w1329 w1385]
                disable-tunnel: w1319 -> [_ w1386]
                frame condition #0 (active) {
                  n519 = Unbundle By Name(w1330) -> ("OPC UA.Client refnum"=w1326:T17)
                  n520 = call-poly <vilib>:"Multiple Read.vi"("error in (no error)"=w1351, "node IDs"=T6 ["ns=2;s=ALR.ALR_blocked", "ns=2;s=ALR.ALR_ON"] ("OPC UA.node IDs"), "OPC UA client refnum in"=w1326) -> ("error out"=w1354:errorcluster, "results"=w1353:T72, "OPC UA client refnum out"=w1338:T17, "service status"=w1355:T41)  [unwired: 5 in]
                  n521 = case shown="0..15" w1355 {
                    tunnel: w1354 -> [w1376 w1379]
                    tunnel: [w1376 w1379] -> w1346
                    tunnel: w1353 -> [_ w1382]
                    tunnel: [_ TRUE] -> w1345
                    tunnel: [_ w1380] -> w1328
                    tunnel: [_ w1377] -> w1327
                    frame 16.., Default {
                    }
                    frame 0..15 {
                      n522 = Index Array(array=w1382) -> (element #1=w1383:T73, element #2=w1378:T73)  [unwired: 2 in]
                      n523 = Unbundle By Name(w1383) -> ("values"=w1380:bool[])
                      n524 = Unbundle By Name(w1378) -> ("values"=w1377:bool[])
                    }
                  }
                  n525 = call-poly <vilib>:"Multiple Read.vi"("error in (no error)"=w1346, "node IDs"=T6 ["ns=2;s=ALR.t_ms", "ns=2;s=ALR.ack_state", "ns=2;s=ALR.color"] ("OPC UA.node IDs"), "OPC UA client refnum in"=w1326) -> ("error out"=w1348:errorcluster, "results"=w1349:T74, "service status"=w1347:T41)  [unwired: 5 in, 1 out]
                  n526 = case shown="0..15" w1347 {
                    tunnel: w1348 -> [w1364 w1368]
                    tunnel: [w1364 w1368] -> w1336
                    tunnel: w1349 -> [_ w1374]
                    tunnel: [_ w1373] -> w1344
                    tunnel: w1345 -> [_ w1372]
                    tunnel: [_ w1370] -> w1335
                    tunnel: [_ w1367] -> w1343
                    tunnel: [_ w1365] -> w1331
                    frame 16.., Default {
                    }
                    frame 0..15 {
                      n527 = Index Array(array=w1374) -> (element #1=w1375:T75, element #2=w1369:T75, element #3=w1366:T75)  [unwired: 3 in]
                      n528 = Unbundle By Name(w1375) -> ("values"=w1373:u32[])
                      n529 = Unbundle By Name(w1369) -> ("values"=w1367:u32[])
                      n530 = Unbundle By Name(w1366) -> ("values"=w1365:u32[])
                      n531 = And(x=w1372, y=TRUE) -> (x .and. y?=w1370:bool)
                    }
                  }
                  n532 = call-poly <vilib>:"Multiple Read.vi"("error in (no error)"=w1336, "node IDs"=T6 ["ns=2;s=ALR.ALR_Names"] ("OPC UA.node IDs"), "OPC UA client refnum in"=w1338) -> ("error out"=w1340:errorcluster, "results"=w1341:T42, "service status"=w1339:T41)  [unwired: 5 in, 1 out]
                  n533 = case shown="0..15" w1339 {
                    tunnel: w1340 -> [w1356 w1357]
                    tunnel: [w1356 w1357] -> w1333
                    tunnel: w1341 -> [_ w1362]
                    tunnel: [_ w1361] -> w1334
                    tunnel: w1335 -> [_ w1360]
                    tunnel: [_ w1358] -> w1332
                    frame 16.., Default {
                    }
                    frame 0..15 {
                      n534 = Index Array(array=w1362) -> (element=w1363:T43)  [unwired: 1 in]
                      n535 = Unbundle By Name(w1363) -> ("values"=w1361:string[])
                      n536 = And(x=w1360, y=TRUE) -> (x .and. y?=w1358:bool)
                    }
                  }
                  n537 = Bundle By Name(cluster=w1329, "ALR blocked"=w1328, "ALR ON"=w1327, "t ms"=w1344, "ack state"=w1343, "color"=w1331) -> (w1342:T10)
                }
                frame condition #1 {
                  n538 = Unbundle By Name(w1393) -> ("ALR_state_SHRV"=w1388)
                  n539 = shared-variable-read(w1388, w1384) -> (w1390:errorcluster, w1387:T10)  [unwired: 2 out]
                  n540 = case shown="Error .." w1390 {
                    selector: w1390 -> [w1395 w1398]
                    tunnel: [w1396 w1397] -> w1389
                    tunnel: w1387 -> [w1396 _]
                    tunnel: [w1395 w1398] -> w1392
                    tunnel: [TRUE _] -> w1391
                    tunnel: w1385 -> [_ w1397]
                    frame No Error {
                    }
                    frame Error {
                    }
                  }
                }
              }
              n541 = in-place-cluster #9("ALR_State"=w1323, "ALR_Names"=w1322) -> (w1315:T23)
              n542 = in-place-match #10(w1320) -> (w1317:errorcluster)
            }
            n543 = Unbundle By Name(w1315) -> ("ALR_State"=w1312:T10, "ALR_Names"=w1311:string[])
            n544 = Unbundle By Name(w1313) -> ("ALR_Descriptions"=w1310:string[])
            n545 = call "view curr alr state_2.vi"("ALR_Descriptions"=w1310, "ALR_Names"=w1311, "ALR_State"=w1312) -> ()  [unwired: 9 in]
          }
          frame "TB1" {
            n546 = in-place {
              in-place-border: [w1431] -> w1403
              in-place-border: w1425 -> [w1428]
              n547 = in-place-cluster #11(w1421) -> ("TB1_ZY_State"=w1427)
              n548 = in-place-match #12(w1424) -> (w1429:errorcluster)
              n549 = disable-structure shown="SERVER==OPC" {
                disable-tunnel: [w1438 w1455] -> w1431
                disable-tunnel: [w1436 w1458] -> w1426
                disable-tunnel: w1429 -> [w1435 w1460]
                disable-tunnel: [w1434 w1456] -> w1430
                disable-tunnel: w1428 -> [w1433 w1454]
                disable-tunnel: w1427 -> [w1432 w1453]
                frame condition #0 (active) {
                  n550 = Unbundle By Name(w1433) -> ("OPC UA.Client refnum"=w1442:T17)
                  n551 = call-poly <vilib>:"Multiple Read.vi"("error in (no error)"=w1435, "node IDs"=T6 ["ns=2;s=EB2TB1.state"] ("OPC UA.node IDs"), "OPC UA client refnum in"=w1442) -> ("error out"=w1440:errorcluster, "results"=w1439:T60, "service status"=w1441:T41)  [unwired: 5 in, 1 out]
                  n552 = case shown="0..15" w1441 {
                    tunnel: w1440 -> [w1444 w1450]
                    tunnel: [w1444 w1449] -> w1434
                    tunnel: w1439 -> [_ w1448]
                    tunnel: [w1443 w1447] -> w1436
                    tunnel: [_ TRUE] -> w1438
                    tunnel: w1432 -> [w1443 _]
                    frame 16.., Default {
                    }
                    frame 0..15 {
                      n553 = Index Array(array=w1448) -> (element=w1452:T76)  [unwired: 1 in]
                      n554 = Unbundle By Name(w1452) -> ("value"=w1451:string)
                      n555 = call "From JSON Text.vim"("Data Type and Default Value"=T64 {"Z"={"Z_Source"=0, "Z_SetState"=0, "Z_State"=0, "Z_State_T"=0, "ZM_State"=0, "ZM_State_T"=0, "ALR  L1"=FALSE, "ALR  L2"=FALSE, "HH_run"=0}, "Y"={"Y_Source"=0, "Y_SetState"=0, "SP_Set"=0.0, "SP"=0.0, "PV"=0.0, "Y_Set"=0.0, "Y"=0.0, "Y_State"={"code"=0, "visible"=FALSE, "color"=0}, "YB"=FALSE}, "ALR_Status"=[]} ("ZY_State"), "error in (no error)"=w1450, "JSON"=w1451) -> ("error out"=w1449:errorcluster, "Data out"=w1447:T64)  [unwired: 7 in]
                    }
                  }
                }
                frame condition #1 {
                  n556 = Unbundle By Name(w1454) -> ("EB2TB1_state"=w1461)
                  n557 = shared-variable-read(w1461, w1460) -> (w1459:errorcluster, w1457:T77)  [unwired: 2 out]
                  n558 = case shown="No Error" w1459 {
                    selector: w1459 -> [w1463 w1466]
                    tunnel: [w1464 T65 {"Z"={"Z_Source"=enum."initialize", "Z_SetState"=enum."initialization", "Z_State"=enum."initialization", "Z_State_T"=0, "ZM_State"=enum."initialization", "ZM_State_T"=0, "ALR  L1"=FALSE, "ALR  L2"=FALSE, "HH_run"=0}, "Y"={"Y_Source"=enum."initialize", "Y_SetState"=enum."initialize", "SP_Set"=0.0, "SP"=0.0, "PV"=0.0, "Y_Set"=0.0, "Y"=0.0, "Y_State"={"code"=0, "visible"=FALSE, "color"=0}, "YB"=FALSE}, "ALR_Status"=[]} ("AI")] -> w1458
                    tunnel: w1457 -> [w1464 _]
                    tunnel: [w1463 w1466] -> w1456
                    tunnel: [TRUE _] -> w1455
                    tunnel: w1453 -> [_ _]
                    frame No Error {
                    }
                    frame Error {
                    }
                  }
                }
              }
              n559 = in-place-cluster #11("TB1_ZY_State"=w1426) -> (w1402:T23)
              n560 = in-place-match #12(w1430) -> (w1419:errorcluster)
            }
            n561 = disable-structure shown="Enabled" {
              disable-tunnel: [w1469 TRUE ("timer end")] -> w1410
              frame Disabled {
                n562 = property on="Property Node" class="Z_OnSwitch (strict)"() -> ("timer end"=w1469:bool)  [unwired: 2 in, 2 out]
              }
              frame Enabled {
              }
            }
            n563 = Unbundle By Name(w1402) -> ("ALR  L1"=w1423, "ALR  L2"=w1422)
            n564 = Unbundle By Name(w1402) -> ("Y_SetState"=w1401, "Y"=w1400)
            n565 = disable-structure shown="Enabled" {
              disable-tunnel: [w1467 TRUE ("timer end")] -> w1399
              frame Disabled {
                n566 = property on="Property Node" class="YQ2 (strict)"() -> ("timer end"=w1467:bool)  [unwired: 2 in, 2 out]
              }
              frame Enabled {
              }
            }
            n567 = Unbundle By Name(w1402) -> ("Z_Source"=w1412, "Z_State"=w1411)
            n568 = Bundle By Name(cluster=T63 {"connect"=FALSE, "Z_Source"=enum."initialize", "Z_State_heating"=enum."initialization"} ("source"), "connect"=w1403, "Z_Source"=w1412, "Z_State_heating"=w1411) -> (w1413:T63)
            n569 = Bundle By Name(cluster=cluster{"connect":bool, "Y_State":T49, "Y":dbl} {"connect"=FALSE, "Y_State"=enum."initialize", "Y"=0.0} ("source"), "connect"=w1403, "Y_State"=w1401, "Y"=w1400) -> (w1404:cluster{"connect":bool, "Y_State":T49, "Y":dbl})
            n570 = Not(x=w1410) -> (.not. x?=w1417:bool)
            n571 = Not(x=w1399) -> (.not. x?=w1408:bool)
            n572 = call "Is Value Changed.vim"("value"=w1413) -> ("changed or first call?"=w1416:bool)
            n573 = feedback #13() -> (w1418:bool)  [unwired: 1 in]
            n574 = feedback-in #13(w1417) -> ()
            n575 = property on="Property Node" class="Bool (strict)"("Visible"=w1423) -> ()  [unwired: 2 in, 2 out]
            n576 = property on="Property Node" class="Bool (strict)"("Visible"=w1422) -> ()  [unwired: 2 in, 2 out]
            n577 = call "Is Value Changed.vim"("value"=w1404) -> ("changed or first call?"=w1407:bool)
            n578 = feedback #14() -> (w1409:bool)  [unwired: 1 in]
            n579 = feedback-in #14(w1408) -> ()
            n580 = Compound Arithmetic op=OR(w1416, w1417, w1418) -> (w1414:bool)
            n581 = Compound Arithmetic op=OR(w1407, w1408, w1409) -> (w1405:bool)
            n582 = case shown="True" w1414 {
              tunnel: w1413 -> [_ w1471]
              frame False {
              }
              frame True {
                n583 = property on="Property Node" class="Z_OnSwitch (strict)"("State"=w1471) -> ()  [unwired: 2 in, 2 out]
              }
            }
            n584 = case shown="True" w1405 {
              tunnel: w1404 -> [_ w1472]
              frame False {
              }
              frame True {
                n585 = property on="Property Node" class="YQ2 (strict)"("State"=w1472) -> ()  [unwired: 2 in, 2 out]
              }
            }
          }
          frame "TB2" {
            n586 = in-place {
              in-place-border: [w1505] -> w1475
              in-place-border: w1499 -> [w1502]
              n587 = in-place-cluster #15(w1494) -> ("TB2_ZY_State"=w1501)
              n588 = in-place-match #16(w1498) -> (w1503:errorcluster)
              n589 = disable-structure shown="SERVER==OPC" {
                disable-tunnel: [w1512 w1529] -> w1505
                disable-tunnel: [w1510 w1532] -> w1500
                disable-tunnel: w1503 -> [w1509 w1534]
                disable-tunnel: [w1508 w1530] -> w1504
                disable-tunnel: w1502 -> [w1507 w1528]
                disable-tunnel: w1501 -> [w1506 w1527]
                frame condition #0 (active) {
                  n590 = Unbundle By Name(w1507) -> ("OPC UA.Client refnum"=w1516:T17)
                  n591 = call-poly <vilib>:"Multiple Read.vi"("error in (no error)"=w1509, "node IDs"=T6 ["ns=2;s=EB2TB2.state"] ("OPC UA.node IDs"), "OPC UA client refnum in"=w1516) -> ("error out"=w1514:errorcluster, "results"=w1513:T60, "service status"=w1515:T41)  [unwired: 5 in, 1 out]
                  n592 = case shown="0..15" w1515 {
                    tunnel: w1514 -> [w1518 w1524]
                    tunnel: [w1518 w1523] -> w1508
                    tunnel: w1513 -> [_ w1522]
                    tunnel: [w1517 w1521] -> w1510
                    tunnel: [_ TRUE] -> w1512
                    tunnel: w1506 -> [w1517 _]
                    frame 16.., Default {
                    }
                    frame 0..15 {
                      n593 = Index Array(array=w1522) -> (element=w1526:T76)  [unwired: 1 in]
                      n594 = Unbundle By Name(w1526) -> ("value"=w1525:string)
                      n595 = call "From JSON Text.vim"("Data Type and Default Value"=T64 {"Z"={"Z_Source"=0, "Z_SetState"=0, "Z_State"=0, "Z_State_T"=0, "ZM_State"=0, "ZM_State_T"=0, "ALR  L1"=FALSE, "ALR  L2"=FALSE, "HH_run"=0}, "Y"={"Y_Source"=0, "Y_SetState"=0, "SP_Set"=0.0, "SP"=0.0, "PV"=0.0, "Y_Set"=0.0, "Y"=0.0, "Y_State"={"code"=0, "visible"=FALSE, "color"=0}, "YB"=FALSE}, "ALR_Status"=[]} ("ZY_State"), "error in (no error)"=w1524, "JSON"=w1525) -> ("error out"=w1523:errorcluster, "Data out"=w1521:T64)  [unwired: 7 in]
                    }
                  }
                }
                frame condition #1 {
                  n596 = Unbundle By Name(w1528) -> ("EB2TB2_state"=w1535)
                  n597 = shared-variable-read(w1535, w1534) -> (w1533:errorcluster, w1531:T77)  [unwired: 2 out]
                  n598 = case shown="No Error" w1533 {
                    selector: w1533 -> [w1537 w1540]
                    tunnel: [w1538 T65 {"Z"={"Z_Source"=enum."initialize", "Z_SetState"=enum."initialization", "Z_State"=enum."initialization", "Z_State_T"=0, "ZM_State"=enum."initialization", "ZM_State_T"=0, "ALR  L1"=FALSE, "ALR  L2"=FALSE, "HH_run"=0}, "Y"={"Y_Source"=enum."initialize", "Y_SetState"=enum."initialize", "SP_Set"=0.0, "SP"=0.0, "PV"=0.0, "Y_Set"=0.0, "Y"=0.0, "Y_State"={"code"=0, "visible"=FALSE, "color"=0}, "YB"=FALSE}, "ALR_Status"=[]} ("AI")] -> w1532
                    tunnel: w1531 -> [w1538 _]
                    tunnel: [w1537 w1540] -> w1530
                    tunnel: [TRUE _] -> w1529
                    tunnel: w1527 -> [_ _]
                    frame No Error {
                    }
                    frame Error {
                    }
                  }
                }
              }
              n599 = in-place-cluster #15("TB2_ZY_State"=w1500) -> (w1495:T23)
              n600 = in-place-match #16(w1504) -> (w1492:errorcluster)
            }
            n601 = disable-structure shown="Enabled" {
              disable-tunnel: [w1541 TRUE ("timer end")] -> w1483
              frame Disabled {
                n602 = property on="Property Node" class="Z_OnSwitch (strict)"() -> ("timer end"=w1541:bool)  [unwired: 2 in, 2 out]
              }
              frame Enabled {
              }
            }
            n603 = Unbundle By Name(w1495) -> ("Y_SetState"=w1476, "Y"=w1474)
            n604 = disable-structure shown="Enabled" {
              disable-tunnel: [w1543 TRUE ("timer end")] -> w1473
              frame Disabled {
                n605 = property on="Property Node" class="YQ2 (strict)"() -> ("timer end"=w1543:bool)  [unwired: 2 in, 2 out]
              }
              frame Enabled {
              }
            }
            n606 = Unbundle By Name(w1495) -> ("ALR  L1"=w1497, "ALR  L2"=w1496)
            n607 = Unbundle By Name(w1495) -> ("Z_Source"=w1485, "Z_State"=w1484)
            n608 = Bundle By Name(cluster=cluster{"connect":bool, "Y_State":T49, "Y":dbl} {"connect"=FALSE, "Y_State"=enum."initialize", "Y"=0.0} ("source"), "connect"=w1475, "Y_State"=w1476, "Y"=w1474) -> (w1477:cluster{"connect":bool, "Y_State":T49, "Y":dbl})
            n609 = Bundle By Name(cluster=T63 {"connect"=FALSE, "Z_Source"=enum."initialize", "Z_State_heating"=enum."initialization"} ("source"), "connect"=w1475, "Z_Source"=w1485, "Z_State_heating"=w1484) -> (w1486:T63)
            n610 = Not(x=w1473) -> (.not. x?=w1481:bool)
            n611 = Not(x=w1483) -> (.not. x?=w1490:bool)
            n612 = property on="Property Node" class="Bool (strict)"("Visible"=w1497) -> ()  [unwired: 2 in, 2 out]
            n613 = property on="Property Node" class="Bool (strict)"("Visible"=w1496) -> ()  [unwired: 2 in, 2 out]
            n614 = call "Is Value Changed.vim"("value"=w1477) -> ("changed or first call?"=w1480:bool)
            n615 = feedback #17() -> (w1482:bool)  [unwired: 1 in]
            n616 = feedback-in #17(w1481) -> ()
            n617 = call "Is Value Changed.vim"("value"=w1486) -> ("changed or first call?"=w1489:bool)
            n618 = feedback #18() -> (w1491:bool)  [unwired: 1 in]
            n619 = feedback-in #18(w1490) -> ()
            n620 = Compound Arithmetic op=OR(w1480, w1481, w1482) -> (w1478:bool)
            n621 = Compound Arithmetic op=OR(w1489, w1490, w1491) -> (w1487:bool)
            n622 = case shown="True" w1487 {
              tunnel: w1486 -> [_ w1545]
              frame False {
              }
              frame True {
                n623 = property on="Property Node" class="Z_OnSwitch (strict)"("State"=w1545) -> ()  [unwired: 2 in, 2 out]
              }
            }
            n624 = case shown="True" w1478 {
              tunnel: w1477 -> [_ w1546]
              frame False {
              }
              frame True {
                n625 = property on="Property Node" class="YQ2 (strict)"("State"=w1546) -> ()  [unwired: 2 in, 2 out]
              }
            }
          }
          frame "TB3" {
            n626 = in-place {
              in-place-border: [w1579] -> w1548
              in-place-border: w1573 -> [w1576]
              n627 = in-place-cluster #19(w1571) -> ("TB3_ZY_State"=w1575)
              n628 = in-place-match #20(w1572) -> (w1577:errorcluster)
              n629 = disable-structure shown="SERVER==OPC" {
                disable-tunnel: [w1586 w1603] -> w1579
                disable-tunnel: [w1584 w1606] -> w1574
                disable-tunnel: w1577 -> [w1583 w1608]
                disable-tunnel: [w1582 w1604] -> w1578
                disable-tunnel: w1576 -> [w1581 w1602]
                disable-tunnel: w1575 -> [w1580 w1601]
                frame condition #0 (active) {
                  n630 = Unbundle By Name(w1581) -> ("OPC UA.Client refnum"=w1590:T17)
                  n631 = call-poly <vilib>:"Multiple Read.vi"("error in (no error)"=w1583, "node IDs"=T6 ["ns=2;s=EB2TB3.state"] ("OPC UA.node IDs"), "OPC UA client refnum in"=w1590) -> ("error out"=w1588:errorcluster, "results"=w1587:T60, "service status"=w1589:T41)  [unwired: 5 in, 1 out]
                  n632 = case shown="0..15" w1589 {
                    tunnel: w1588 -> [w1592 w1598]
                    tunnel: [w1592 w1597] -> w1582
                    tunnel: w1587 -> [_ w1596]
                    tunnel: [w1591 w1595] -> w1584
                    tunnel: [_ TRUE] -> w1586
                    tunnel: w1580 -> [w1591 _]
                    frame 16.., Default {
                    }
                    frame 0..15 {
                      n633 = Index Array(array=w1596) -> (element=w1600:T76)  [unwired: 1 in]
                      n634 = Unbundle By Name(w1600) -> ("value"=w1599:string)
                      n635 = call "From JSON Text.vim"("Data Type and Default Value"=T64 {"Z"={"Z_Source"=0, "Z_SetState"=0, "Z_State"=0, "Z_State_T"=0, "ZM_State"=0, "ZM_State_T"=0, "ALR  L1"=FALSE, "ALR  L2"=FALSE, "HH_run"=0}, "Y"={"Y_Source"=0, "Y_SetState"=0, "SP_Set"=0.0, "SP"=0.0, "PV"=0.0, "Y_Set"=0.0, "Y"=0.0, "Y_State"={"code"=0, "visible"=FALSE, "color"=0}, "YB"=FALSE}, "ALR_Status"=[]} ("ZY_State"), "error in (no error)"=w1598, "JSON"=w1599) -> ("error out"=w1597:errorcluster, "Data out"=w1595:T64)  [unwired: 7 in]
                    }
                  }
                }
                frame condition #1 {
                  n636 = Unbundle By Name(w1602) -> ("EB2TB3_state"=w1609)
                  n637 = shared-variable-read(w1609, w1608) -> (w1607:errorcluster, w1605:T77)  [unwired: 2 out]
                  n638 = case shown="Error .." w1607 {
                    selector: w1607 -> [w1611 w1614]
                    tunnel: [w1612 T65 {"Z"={"Z_Source"=enum."initialize", "Z_SetState"=enum."initialization", "Z_State"=enum."initialization", "Z_State_T"=0, "ZM_State"=enum."initialization", "ZM_State_T"=0, "ALR  L1"=FALSE, "ALR  L2"=FALSE, "HH_run"=0}, "Y"={"Y_Source"=enum."initialize", "Y_SetState"=enum."initialize", "SP_Set"=0.0, "SP"=0.0, "PV"=0.0, "Y_Set"=0.0, "Y"=0.0, "Y_State"={"code"=0, "visible"=FALSE, "color"=0}, "YB"=FALSE}, "ALR_Status"=[]} ("AI")] -> w1606
                    tunnel: w1605 -> [w1612 _]
                    tunnel: [w1611 w1614] -> w1604
                    tunnel: [TRUE _] -> w1603
                    tunnel: w1601 -> [_ _]
                    frame No Error {
                    }
                    frame Error {
                    }
                  }
                }
              }
              n639 = in-place-cluster #19("TB3_ZY_State"=w1574) -> (w1569:T23)
              n640 = in-place-match #20(w1578) -> (w1566:errorcluster)
            }
            n641 = disable-structure shown="Enabled" {
              disable-tunnel: [w1615 TRUE ("timer end")] -> w1557
              frame Disabled {
                n642 = property on="Property Node" class="Z_OnSwitch (strict)"() -> ("timer end"=w1615:bool)  [unwired: 2 in, 2 out]
              }
              frame Enabled {
              }
            }
            n643 = Unbundle By Name(w1569) -> ("Y_SetState"=w1550, "Y"=w1549)
            n644 = Unbundle By Name(w1569) -> ("ALR  L1"=w1568, "ALR  L2"=w1567)
            n645 = disable-structure shown="Enabled" {
              disable-tunnel: [w1617 TRUE ("timer end")] -> w1547
              frame Disabled {
                n646 = property on="Property Node" class="YQ2 (strict)"() -> ("timer end"=w1617:bool)  [unwired: 2 in, 2 out]
              }
              frame Enabled {
              }
            }
            n647 = Unbundle By Name(w1569) -> ("Z_Source"=w1559, "Z_State"=w1558)
            n648 = Bundle By Name(cluster=cluster{"connect":bool, "Y_State":T49, "Y":dbl} {"connect"=FALSE, "Y_State"=enum."initialize", "Y"=0.0} ("source"), "connect"=w1548, "Y_State"=w1550, "Y"=w1549) -> (w1551:cluster{"connect":bool, "Y_State":T49, "Y":dbl})
            n649 = Bundle By Name(cluster=T63 {"connect"=FALSE, "Z_Source"=enum."initialize", "Z_State_heating"=enum."initialization"} ("source"), "connect"=w1548, "Z_Source"=w1559, "Z_State_heating"=w1558) -> (w1560:T63)
            n650 = Not(x=w1547) -> (.not. x?=w1555:bool)
            n651 = Not(x=w1557) -> (.not. x?=w1564:bool)
            n652 = property on="Property Node" class="Bool (strict)"("Visible"=w1568) -> ()  [unwired: 2 in, 2 out]
            n653 = property on="Property Node" class="Bool (strict)"("Visible"=w1567) -> ()  [unwired: 2 in, 2 out]
            n654 = call "Is Value Changed.vim"("value"=w1551) -> ("changed or first call?"=w1554:bool)
            n655 = feedback #21() -> (w1556:bool)  [unwired: 1 in]
            n656 = feedback-in #21(w1555) -> ()
            n657 = call "Is Value Changed.vim"("value"=w1560) -> ("changed or first call?"=w1563:bool)
            n658 = feedback #22() -> (w1565:bool)  [unwired: 1 in]
            n659 = feedback-in #22(w1564) -> ()
            n660 = Compound Arithmetic op=OR(w1554, w1555, w1556) -> (w1552:bool)
            n661 = Compound Arithmetic op=OR(w1563, w1564, w1565) -> (w1561:bool)
            n662 = case shown="True" w1561 {
              tunnel: w1560 -> [_ w1619]
              frame False {
              }
              frame True {
                n663 = property on="Property Node" class="Z_OnSwitch (strict)"("State"=w1619) -> ()  [unwired: 2 in, 2 out]
              }
            }
            n664 = case shown="True" w1552 {
              tunnel: w1551 -> [_ w1620]
              frame False {
              }
              frame True {
                n665 = property on="Property Node" class="YQ2 (strict)"("State"=w1620) -> ()  [unwired: 2 in, 2 out]
              }
            }
          }
          frame "Exit" {
            n666 = local read "Останов\nпрограммы"() -> (w1624:bool)
          }
        }
        n667 = Wait Until Next ms Multiple(millisecond multiple=w1025) -> ()  [unwired: 1 out]
      }
    }
    frame Enabled {
    }
  }
  n668 = Unregister For Events(event registration refnum=w16) -> ()  [unwired: 1 in, 1 out]
  n669 = disable-structure shown="Disabled" {
    disable-tunnel: w17 -> [w1627 _]
    frame Disabled {
      n670 = invoke class="VI" method="FP.Close"(reference=w1627) -> ()  [unwired: 2 in, 3 out]
    }
    frame Enabled {
    }
  }
  n671 = flat-sequence {
    tunnel: w11 -> [w1638]
    tunnel: w10 -> [w1636]
    tunnel: w10 -> [w1635]
    tunnel: w2 -> [w1632]
    tunnel: w5 -> [w1630]
    frame #0 {
      w1628 = TRUE
      n672 = disable-structure shown="SERVER==OPC" {
        disable-tunnel: w1632 -> [w1663 w1691]
        disable-tunnel: [w1677 w1683] -> w1631
        frame condition #0 {
          n673 = Unbundle By Name(w1663) -> ("EB2TB3_control"=w1662, "EB2TB3_state"=w1661, "EB3TB1_control"=w1660, "EB3TB1_state"=w1659, "EB3TB2_control"=w1658, "EB3TB2_state"=w1657, "EB3TB3_control"=w1656, "EB3TB3_state"=w1655)
          n674 = Close Variable Connection(11:w1662) -> (0:w1652:errorcluster)  [unwired: 1 in]
          n675 = Close Variable Connection(11:w1661) -> (0:w1651:errorcluster)  [unwired: 1 in]
          n676 = Close Variable Connection(11:w1660) -> (0:w1650:errorcluster)  [unwired: 1 in]
          n677 = Close Variable Connection(11:w1659) -> (0:w1649:errorcluster)  [unwired: 1 in]
          n678 = Close Variable Connection(11:w1658) -> (0:w1648:errorcluster)  [unwired: 1 in]
          n679 = Close Variable Connection(11:w1657) -> (0:w1647:errorcluster)  [unwired: 1 in]
          n680 = Close Variable Connection(11:w1656) -> (0:w1646:errorcluster)  [unwired: 1 in]
          n681 = Close Variable Connection(11:w1655) -> (0:w1645:errorcluster)  [unwired: 1 in]
          n682 = Merge Errors(w1652, w1651, w1650, w1649, w1648, w1647, w1646, w1645) -> (w1644:errorcluster)
          n683 = Unbundle By Name(w1663) -> ("AI_SHVR"=w1682, "AI_Names_SHVR"=w1681, "DI_SHVR"=w1680, "DI_Names_SHVR"=w1679, "ALR_state_SHRV"=w1673, "ALR_Descriptions_SHRV"=w1672, "EB2TB1_control"=w1667, "EB2TB1_state"=w1666, "EB2TB2_control"=w1665, "EB2TB2_state"=w1664)
          n684 = Close Variable Connection(11:w1682) -> (0:w1678:errorcluster)  [unwired: 1 in]
          n685 = Close Variable Connection(11:w1681) -> (0:w1676:errorcluster)  [unwired: 1 in]
          n686 = Close Variable Connection(11:w1680) -> (0:w1675:errorcluster)  [unwired: 1 in]
          n687 = Close Variable Connection(11:w1679) -> (0:w1674:errorcluster)  [unwired: 1 in]
          n688 = Close Variable Connection(11:w1673) -> (0:w1671:errorcluster)  [unwired: 1 in]
          n689 = Close Variable Connection(11:w1672) -> (0:w1670:errorcluster)  [unwired: 1 in]
          n690 = Close Variable Connection(11:w1667) -> (0:w1669:errorcluster)  [unwired: 1 in]
          n691 = Close Variable Connection(11:w1666) -> (0:w1668:errorcluster)  [unwired: 1 in]
          n692 = Close Variable Connection(11:w1665) -> (0:w1654:errorcluster)  [unwired: 1 in]
          n693 = Close Variable Connection(11:w1664) -> (0:w1653:errorcluster)  [unwired: 1 in]
          n694 = Merge Errors(w1678, w1676, w1675, w1674, w1671, w1670, w1669, w1668, w1654, w1653, w1644) -> (w1677:errorcluster)
        }
        frame condition #1 (active) {
          # "7."
          # "8."
          # "6."
          n695 = Unbundle By Name(w1691) -> ("OPC UA.subscription IDs"=w1688:T18[], "OPC UA.Client refnum"=w1690:T17, "OPC UA.node IDs"=w1689:T6, "OPC UA.data change event"=w1686:refnum<user-event>)
          n696 = Destroy User Event(user event=w1686) -> (error out=w1684:errorcluster)  [unwired: 1 in]
          n697 = Index Array(array=w1688) -> (element=w1687:T18)  [unwired: 1 in]
          n698 = call <vilib>:"Delete Monitored Nodes.vi"("node IDs"=w1689, "subscription ID in"=w1687, "OPC UA client refnum in"=w1690) -> ("error out"=w1693:errorcluster, "OPC UA client refnum out"=w1692:T17)  [unwired: 4 in, 3 out]
          n699 = call <vilib>:"Delete Subscriptions.vi"("error in (no error)"=w1693, "subscription IDs"=w1688, "OPC UA client refnum in"=w1692) -> ("error out"=w1695:errorcluster, "OPC UA client refnum out"=w1694:T17)  [unwired: 6 in, 1 out]
          n700 = call <vilib>:"Disconnect.vi"("error in (no error)"=w1695, "OPC UA client refnum in"=w1694) -> ("error out"=w1685:errorcluster)  [unwired: 9 in]
          n701 = Merge Errors(w1685, w1684) -> (w1683:errorcluster)
        }
      }
      n702 = Unbundle By Name(w1630) -> ("RegRefs"=w1629:refnum<vi>[])
      n703 = Unbundle By Name(w1632) -> ("AI_refs"=w1633:refnum<vi>[])
      n704 = Merge Errors(w1631, w1635, w1636, w1638) -> (w1637:errorcluster)
      n705 = call <vilib>:"Simple Error Handler.vi"("error in (no error)"=w1637) -> ()  [unwired: 4 in, 5 out]
      n706 = disable-structure shown="Disabled" {
        frame Disabled {
          n707 = property class="App"() -> (error out=w1642:errorcluster, "App.Kind"=w1643:T79)  [unwired: 2 in, 1 out]
          n708 = case shown="\"Run Time System\"" w1643 {
            tunnel: w1642 -> [_ _]
            frame Default {
            }
            frame "Run Time System" {
              n709 = Quit LabVIEW() -> ()  [unwired: 1 in]
            }
          }
        }
        frame Enabled {
        }
      }
      n710 = for {
        tunnel: w1633 -> [w1697] mode=indexing
        n711 = Not A Number/Path/Refnum?(number/path/refnum=w1697) -> (NaN/Path/Refnum?=w1696:bool)
        n712 = case shown="False" w1696 {
          tunnel: w1697 -> [w1698 _]
          frame False {
            n713 = Close Reference(reference=w1698) -> ()  [unwired: 1 in, 1 out]
          }
          frame True {
          }
        }
      }
      n714 = for {
        tunnel: w1629 -> [w1640] mode=indexing
        n715 = Not A Number/Path/Refnum?(number/path/refnum=w1640) -> (NaN/Path/Refnum?=w1639:bool)
        n716 = case shown="False" w1639 {
          tunnel: w1640 -> [w1641 _]
          frame False {
            n717 = Close Reference(reference=w1641) -> ()  [unwired: 1 in, 1 out]
          }
          frame True {
          }
        }
      }
      n718 = local write "Останов\nпрограммы"(FALSE ("stop")) -> ()
      n719 = property on="N 1" class="DigNum (strict)"("Visible"=w1628) -> ()  [unwired: 2 in, 2 out]
      n720 = property on="N 2" class="DigNum (strict)"("Visible"=w1628) -> ()  [unwired: 2 in, 2 out]
      n721 = property on="N 3" class="DigNum (strict)"("Visible"=w1628) -> ()  [unwired: 2 in, 2 out]
      n722 = property on="N 4" class="DigNum (strict)"("Visible"=w1628) -> ()  [unwired: 2 in, 2 out]
      n723 = property on="N 5" class="DigNum (strict)"("Visible"=w1628) -> ()  [unwired: 2 in, 2 out]
      n724 = property on="N 6" class="DigNum (strict)"("Visible"=w1628) -> ()  [unwired: 2 in, 2 out]
      n725 = property on="N 7" class="DigNum (strict)"("Visible"=w1628) -> ()  [unwired: 2 in, 2 out]
      n726 = property on="N 8" class="DigNum (strict)"("Visible"=w1628) -> ()  [unwired: 2 in, 2 out]
      n727 = property on="N 9" class="DigNum (strict)"("Visible"=w1628) -> ()  [unwired: 2 in, 2 out]
      n728 = property on="N 10" class="DigNum (strict)"("Visible"=w1628) -> ()  [unwired: 2 in, 2 out]
      n729 = property on="N 11" class="DigNum (strict)"("Visible"=w1628) -> ()  [unwired: 2 in, 2 out]
      n730 = property on="N 12" class="DigNum (strict)"("Visible"=w1628) -> ()  [unwired: 2 in, 2 out]
      n731 = property on="N 13" class="DigNum (strict)"("Visible"=w1628) -> ()  [unwired: 2 in, 2 out]
      n732 = property on="N 14" class="DigNum (strict)"("Visible"=w1628) -> ()  [unwired: 2 in, 2 out]
      n733 = property on="N 15" class="DigNum (strict)"("Visible"=w1628) -> ()  [unwired: 2 in, 2 out]
      n734 = property on="N 16" class="DigNum (strict)"("Visible"=w1628) -> ()  [unwired: 2 in, 2 out]
      n735 = property on="N 17" class="DigNum (strict)"("Visible"=w1628) -> ()  [unwired: 2 in, 2 out]
      n736 = property on="N 18" class="DigNum (strict)"("Visible"=w1628) -> ()  [unwired: 2 in, 2 out]
      n737 = property on="N 19" class="DigNum (strict)"("Visible"=w1628) -> ()  [unwired: 2 in, 2 out]
      n738 = property on="N 20" class="DigNum (strict)"("Visible"=w1628) -> ()  [unwired: 2 in, 2 out]
    }
  }
